vi "TI sbRIO Main (RT).vi"() -> ()   [LabVIEW 2013]
uses:
  Type Defs/Controller Names.ctl
  Controls/Alarm Config.ctl
  Controls/Alarm Definition.ctl
  Controls/Alarm Profile Config.ctl
  Type Defs/App Config.ctl
  SubVIs/Data Logger/Data Log Init.ctl
  Type Defs/Sequence States.ctl
  Type Defs/Controller List.ctl
  Controls/Tank CMDs.ctl
  Controls/Controller Config.ctl
  Controls/Pump Data.ctl
  Controls/Tank Data.ctl
  Controls/HMI Cluster.ctl
  Controls/HMI Header.ctl
  Controls/HMI Tog Buttons.ctl
  Controls/HMI Mom Buttons.ctl
  Controls/App Global Mode.ctl
  SubVIs/Data Logger/Data Logger Mode.ctl
  SubVIs/Data Logger/Data Log Start.ctl
  Controls/Power Supply Global Mode.ctl
  Controls/RPi HMI Mode.ctl
  Controls/Email Mode.ctl
  Type Defs/Pump Data Mode.ctl
  SubVIs/Watlow Modbus/Modbus Mode.ctl
  SubVIs/Watlow Modbus/Modbus Variable.ctl
  Controls/HMI Global Mode.ctl
  <vilib>/FPGAPlugInAG/sbRIO-9626/niLvFpga_Open_sbRIO-9626.vi
  <vilib>/Utility/error.llb/Error Cluster From Error Code.vi
  <vilib>/rvi/errors/niLvFpgaAdjustHostInterfaceError.vi
  <vilib>/Utility/file.llb/Write To Spreadsheet File (string).vi
  <vilib>/rvi/interface/nirviOpenFPGA/nirviOpenFPGA.xnode
  Controls/FPGA_Reference.ctl
  FPGA/bitfiles/TI sbRIO PWM (FPGA) v1.0.lvbitx
  <vilib>/rvi/interface/nirviReadWriteControl/nirviReadWriteControl.xnode
  NiFpgaLv.dll
  <vilib>/Utility/config.llb/NI_LVConfig.lvlib
panel:
  out "Read Inputs (ms)":u32
  out "Update Screen (ms)":u32
  out "Run Step (ms)":u32
  in  "Fuel Change Tab":enum32{"Page 1", "Page 2"}(tab)
  in  "pb.Fuel Change OK":bool
  in  "Reset Tab":enum32{"Page 1", "Page 2"}(tab)
  in  "pb.Reset OK":bool
  in  "pb.Reset Cancel":bool
  in  "Save As Tab":enum32{"Page 1", "Page 2"}(tab)
  in  "New Profile Name:":string
  in  "pb.Save As OK":bool
  in  "pb.Save As Cancel":bool
  in  "Alarm Tab":enum32{"Page 1", "Page 2"}(tab)
  out "Alarm Message":string
  in  "pb.Alarm OK":bool
  in  "Set Time Tab":enum32{"Page 1", "Page 2"}(tab)
  in  "pb.Set Time OK":bool
  in  "pb.Set Time Cancel":bool
  in  "New Time":dbl format="%<%H:%M:%S>t"
  in  "Pump Timers Tab":enum32{"Page 1", "Page 2"}(tab)
  in  "pb.Time Reset All":bool
  out "Elapsed Time:":dbl[](array[numeric])=[7.1, 7.1, 7.1, 458133.45, 458138.85000000003, 458126.75] format="%<%H:%M:%S>t"
  in  "pb.Resets":bool[](array[boolean])=[FALSE, FALSE, FALSE, FALSE, FALSE, FALSE]
  in  "pb.Sets":bool[](array[boolean])=[FALSE, FALSE, FALSE, FALSE, FALSE, FALSE]
  out "CPU Usage:":dbl=7.74131899555212 format="%.1f"
  in  "Live Data Tab":enum32{"Page 1", "Page 2"}(tab)
  in  "Controller\nCMD":dbl[](array[numeric])=[0.0, 0.0, 0.0, 0.0, 0.0, 0.0] min=0.0 max=1.0 step=1.0 format="%#.2f"
  out "Speed":dbl[](array[numeric]) caption="Speed\n(RPM)" format="%#.0f"
  out "ControllerCurrent":dbl[](array[numeric])=[0.015201568603515625, 0.00335693359375, 0.003021240234375, 0.12260055541992188, 0.06085968017578125, 0.052234649658203125] caption="Controller\nCurrent\n(DC)" format="%.1f"
  out "PumpCurrent":dbl[](array[numeric])=[0.015201568603515625, 0.00335693359375, 0.003021240234375, 0.12260055541992188, 0.06085968017578125, 0.052234649658203125] caption="Pump\nCurrent\n(DC)" format="%.1f"
  out "Flow":dbl[](array[numeric])=[0.0, 0.0, 0.0, 0.125, 0.0625, 0.0625] caption="Flow\n(L/H)" format="%#.0f"
  out "Pressure":dbl[](array[numeric])=[0.015201568603515625, 0.00335693359375, 0.003021240234375, 0.12260055541992188, 0.06085968017578125, 0.052234649658203125] caption="Pressure\n(kPa)" format="%#.0f"
  out "Ave. Speed":dbl=7.74131899555212 format="%.1f"
  out "Voltages":dbl[](array[numeric])=[0.015201568603515625, 0.00335693359375, 0.003021240234375, 0.12260055541992188, 0.06085968017578125, 0.052234649658203125] caption="Pump\nVoltage\n(V)" format="%.1f"
  in  "App Config":T1={"Location"="Tanks 162-163", "Profiles Path"=path "c:/Profiles", "Current Profile"="", "CA Number"="", "Cycles Completed"=0, "Controller Type:"=enum."Kuhnke", "Stagger Time (ms)"=0, "Tank 1 Fuel"="", "Tank 2 Fuel"="", "Serial Numbers"={"Position 1 SN"="", "Position 2 SN"="", "Poaition 3 SN"="", "Position 4 SN"="", "Position 5 SN"="", "Position 6 SN"=""}, "Pumps Present"={"Pump 1"=FALSE, "Pump 2"=FALSE, "Pump 3"=FALSE, "Pump 4"=FALSE, "Pump 5"=FALSE, "Pump 6"=FALSE}, "VoltCtrlRef"="", "VoltageSelect"=FALSE, "Watlow Present"=TRUE, "Temp 1"=0.0, "Temp 2"=0.0, "V_Run PI?"=FALSE, "Voltage Limits"={"V_Step"=1e-05, "V_CmdMax"=0.0, "V_CmdMin"=0.0}, "Voltage Far PI"={"V_FarSlew"=10.0, "V_FarKp"=0.0, "V_FarKi"=0.0}, "Voltage Mid PI"={"V_MidSlew"=10.0, "V_MidKp"=0.0, "V_MidKi"=0.0}, "Voltage Close PI"={"V_CloseSlew"=10.0, "V_CloseKp"=0.0, "V_CloseKi"=0.0}, "Voltage Scale"={"V_FFm"=0.0, "V_FFb"=0.0}, "Voltage Cutoffs"={"V_MidCutoff"=0.0, "V_CloseCutoff"=0.0}, "Pressure Scale"={"Pres_FFm"=1e-05, "Pres_FFb"=0.0}, "Temp Format"=0, "Temp Tolerance"=0.0, "Target Voltage"=0.0, "Target Pressure"=0.0, "Data Log Init"={"Data Path"=path "u:/Data", "Data Log Rate (S/s)"=1, "AKLH Rate (Hours/S)"=0.1, "Sync Time Offset (min)"=180, "IP Last 3"=0, "WebDAV IP"="10.31.176.36"}, "Email Handler IP"="10.30.189.34", "ADC Check"=FALSE}
  in  "Monitoring Tab":enum32{"Page 1", "Page 2"}(tab)
  out "Avg Press:":dbl=7.74131899555212
  in  "pb.E Stop":bool
  in  "Ignition Relay":T4
  in  "Power Relay":T4
  out "Temp2":dbl caption="Tank 2 Temp (C):" format="%.1f"
  out "Temp1":dbl caption="Tank 1 Temp (C):" format="%.1f"
  out "PS Actual (V):":dbl format="%.2f"
  in  "Power Supply Cmd:":dbl min=0.0 max=20.0 format="%#.2f"
  in  "PressureCMD":dbl caption="Pressure Cmd:" min=0.0 max=825.0 format="%#.2f"
  in  "Pumps Present":T4={"Pump 1"=TRUE, "Pump 2"=TRUE, "Pump 3"=TRUE, "Pump 4"=TRUE, "Pump 5"=TRUE, "Pump 6"=TRUE}
  in  "Tank 1 Temp Cmd:":dbl caption="deg C"
  in  "Tank 2 Temp Cmd:":dbl caption="deg C"
  in  "Title Tab":enum32{"Page 1", "Page 2"}(tab)
  in  "Title":string="TI Automotive sbRIO, v3.0"
  out "Time/Date":string
  in  "Login":bool
  in  "pb.Stop Profile":bool
  in  "Main Tab":T5(tab)
  out "Email Alarms Disabled":bool
  in  "Target Pressure:":dbl
  in  "Target Voltage:":dbl
  out "Recording":bool
  in  "Controller Type:":T2
  in  "Tank 1 Fuel Type:":string
  in  "Tank 2 Fuel Type:":string
  in  "Stagger Time (ms):":i32
  in  "CA Number:":string
  in  "Profile Name:":string(combo)="test"
  in  "pb.Save As":bool
  out "Current Step:":i32=2
  out "Step Time Left:":dbl=0.21101045608520508
  out "Cycles Completed:":u32=17
  in  "pb.Cycle Reset":bool
  out "Location:":string
  in  "pb.Run Profile":bool
  in  "Serial Numbers":T6
  in  "Profile:":string[][](table)=[["1", "2.0", "0.0", "0.0", "0.0", "67.6", "67.6", "67.6"], ["2", "1.0", "0.0", "0.0", "0.0", "10.0", "10.0", "10.0"]]
  in  "Disable Alarm Email":bool
  in  "Temp Tolerance":dbl=3.0 min=0.0 max=999999.0 step=1.0
  in  "Thermocouple":enum16{"2 TC/2 Tanks", "1 TC/1 Tank"}(ring)
  out "ADC Errors":i32
  in  "pb.Tare Pressure":bool
  in  "Data Log Enabled":bool=TRUE
  in  "RPMhyst":fxp<+,25,6>=1.0
  in  "pb.FuelChange":bool
  in  "Alarm Config":T7
  in  "WebDAV Push":bool
  in  "Concat Data":bool
  in  "Cutoffs":cluster{"Mid Range":dbl, "Close Range":dbl} {"Close Range" min=-100000.0 max=100000.0 step=1e-05 format="%#.5f"; "Mid Range" min=-100000.0 max=100000.0 step=1e-05 format="%#.5f"}
  in  "Mid PI":cluster{"Slew Rate":dbl, "Kp":dbl, "Ki":dbl}={"Slew Rate"=10.0, "Kp"=0.0, "Ki"=0.0} {"Ki" min=-100000.0 max=100000.0 step=1e-05 format="%#.5f"; "Kp" min=-100000.0 max=100000.0 step=1e-05 format="%#.5f"; "Slew Rate" min=0.0 max=1000000.0 step=0.01 format="%#.5f"}
  in  "Close PI":cluster{"Slew Rate":dbl, "Kp":dbl, "Ki":dbl}={"Slew Rate"=10.0, "Kp"=0.0, "Ki"=0.0} {"Ki" min=-100000.0 max=100000.0 step=1e-05 format="%#.5f"; "Kp" min=-100000.0 max=100000.0 step=1e-05 format="%#.5f"; "Slew Rate" min=0.0 max=1000000.0 step=0.01 format="%#.5f"}
  in  "Pressure Scale":cluster{"M":dbl, "B":dbl}={"M"=1e-05, "B"=0.0} {"B" min=-100000.0 max=100000.0 step=1e-05 format="%#.5f"; "M" min=-100000.0 max=100000.0 step=1e-05 format="%#.5f"}
  in  "Closed Loop Voltage":bool
  in  "Voltage Limits":cluster{"Step":dbl, "Max":dbl, "Min":dbl}={"Step"=1e-05, "Max"=0.0, "Min"=0.0} {"Min" min=0.0 max=10.0 step=1e-05 format="%#.5f"; "Max" min=0.0 max=10.0 step=1e-05 format="%#.5f"; "Step" min=0.0 max=100.0 step=1e-05 format="%#.5f"}
  in  "Far PI":cluster{"Slew Rate":dbl, "Kp":dbl, "Ki":dbl}={"Slew Rate"=10.0, "Kp"=0.0, "Ki"=0.0} {"Ki" min=-100000.0 max=100000.0 step=1e-05 format="%#.5f"; "Kp" min=-100000.0 max=100000.0 step=1e-05 format="%#.5f"; "Slew Rate" min=0.0 max=1000000.0 step=0.01 format="%#.5f"}
  in  "Voltage Scale":cluster{"M":dbl, "B":dbl} {"B" min=-100000.0 max=100000.0 step=1e-05 format="%#.5f"; "M" min=-100000.0 max=100000.0 step=1e-05 format="%#.5f"}
  # "Fuel Change was logged."
  # "Are you sure you want to reset?"
  # "Enter a new elapsed time."
  # "Pump Timers"
  # "Live Data"
  # "Manual Control"
  # "V"
  # "kPa"
  # "degC"
  # "degC"
  # "Voltage Control"
  # "Pressure Control"
  # "Data Server"
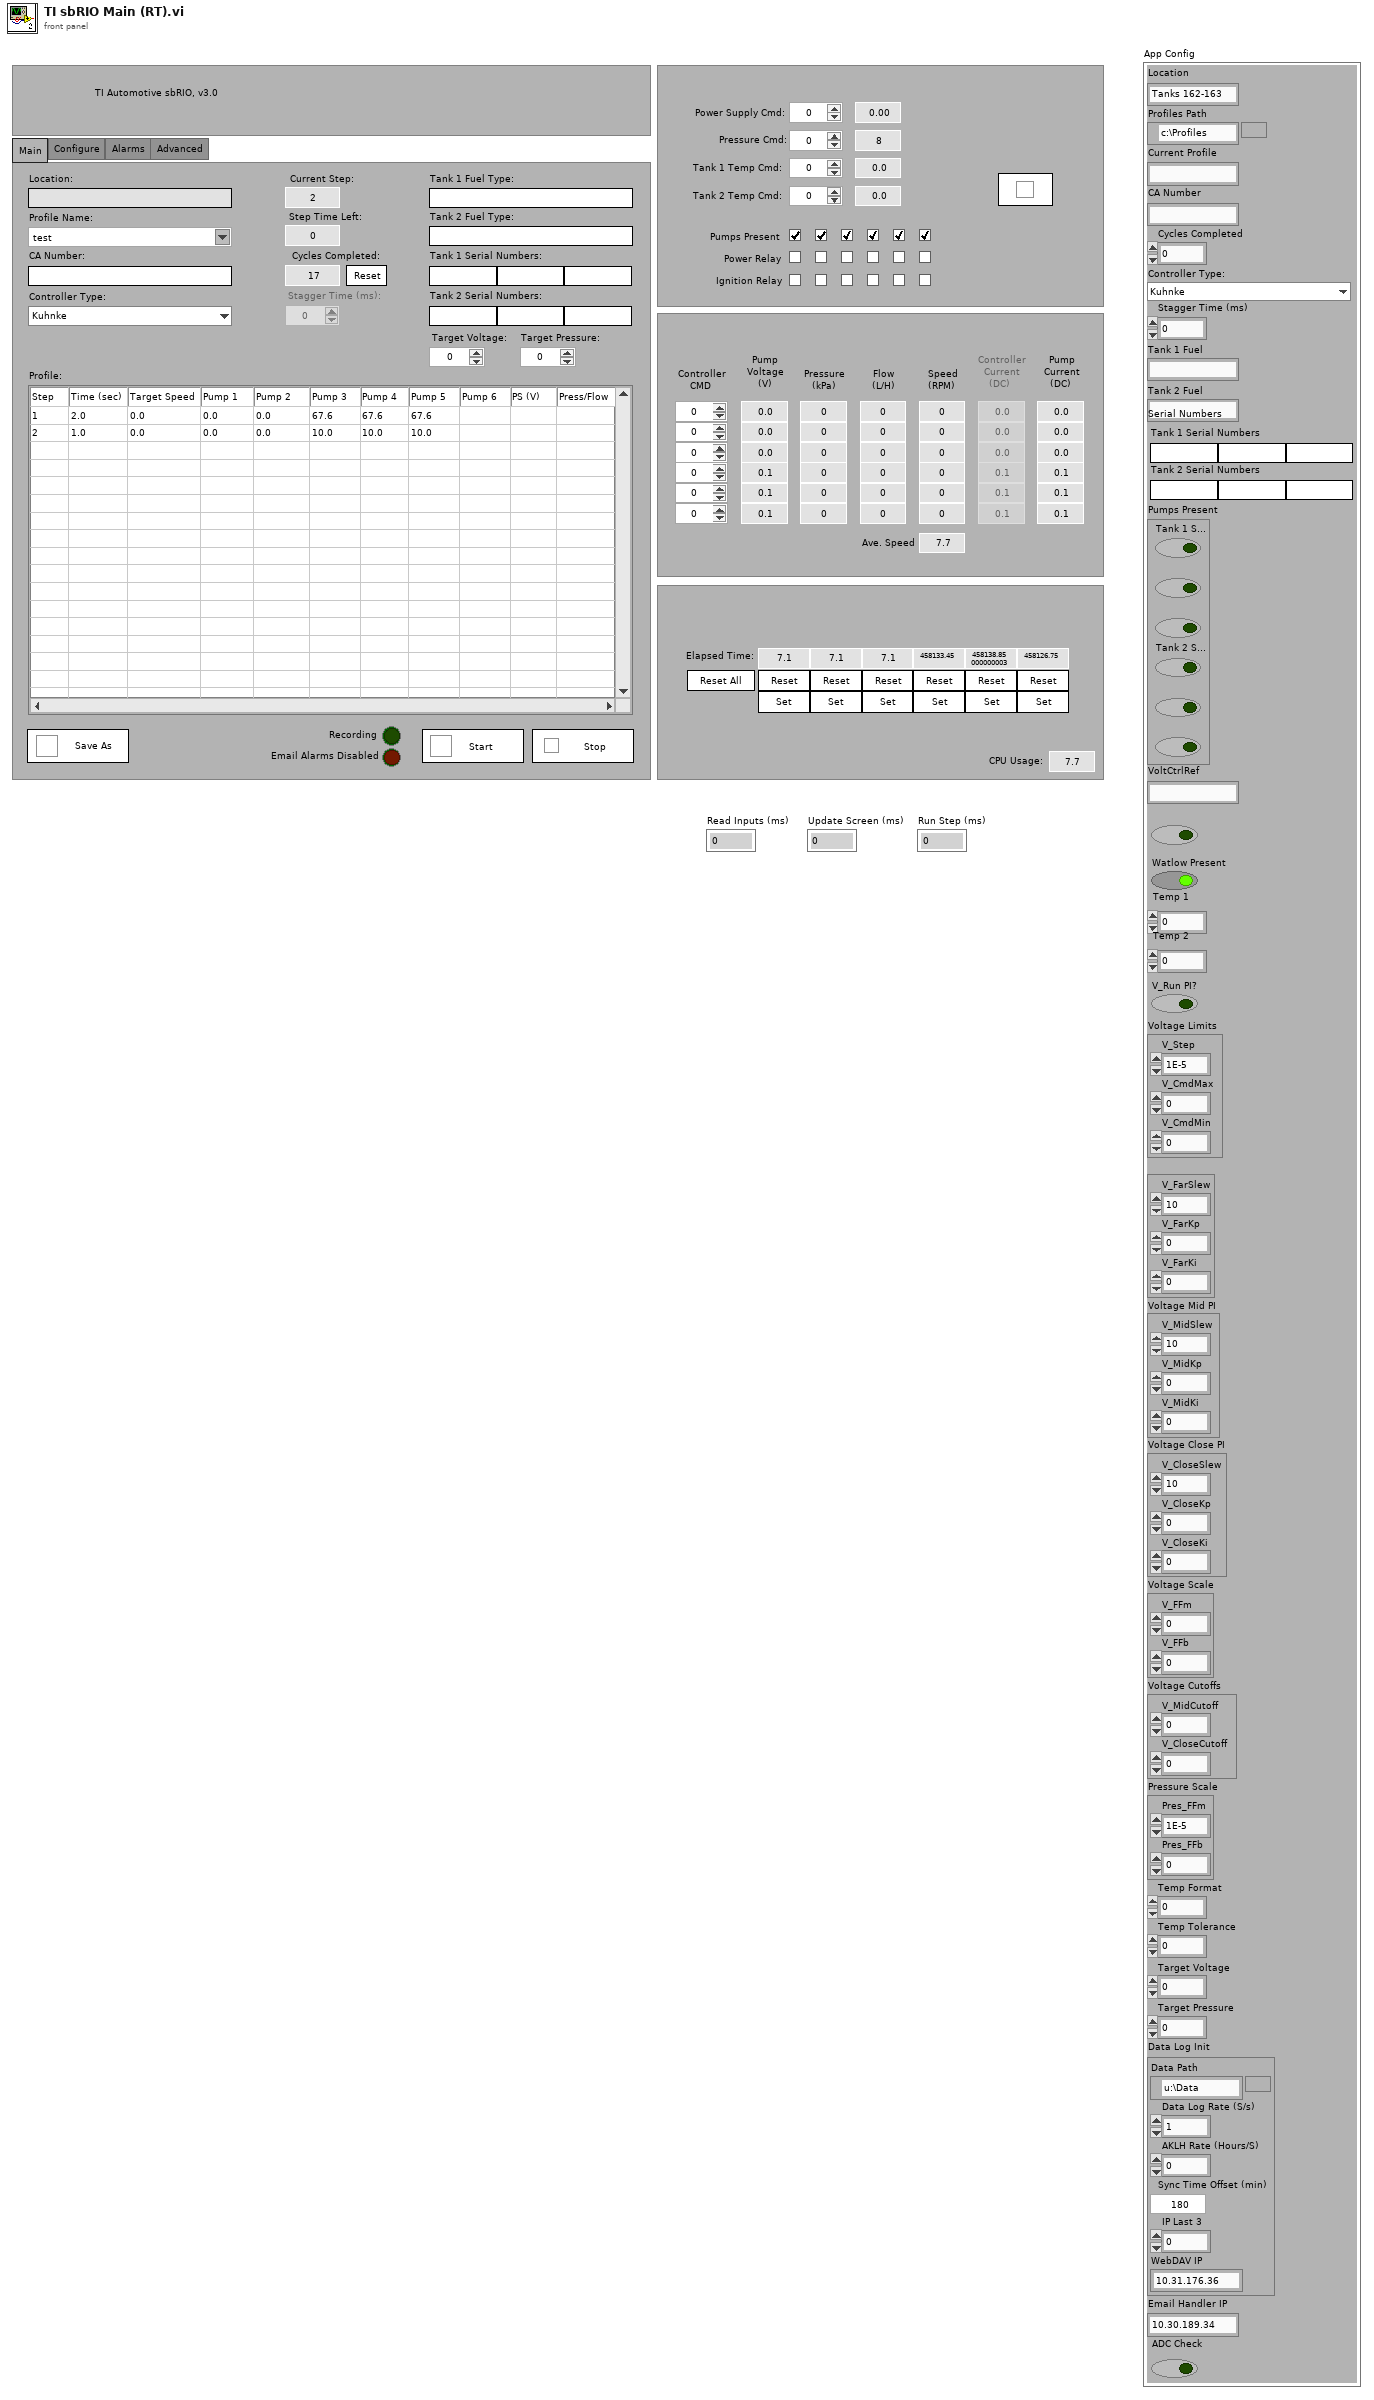
[diagram p1: front panel]
types:
  T1 = typedef "App Config.ctl" = cluster{"Location":string, "Profiles Path":path, "Current Profile":string, "CA Number":string, "Cycles Completed":u32, "Controller Type:":T2, "Stagger Time (ms)":i32, "Tank 1 Fuel":string, "Tank 2 Fuel":string, "Serial Numbers":cluster{"Position 1 SN":string, "Position 2 SN":string, "Poaition 3 SN":string, "Position 4 SN":string, "Position 5 SN":string, "Position 6 SN":string}, "Pumps Present":cluster{"Pump 1":bool, "Pump 2":bool, "Pump 3":bool, "Pump 4":bool, "Pump 5":bool, "Pump 6":bool}, "VoltCtrlRef":string, "VoltageSelect":bool, "Watlow Present":bool, "Temp 1":dbl, "Temp 2":dbl, "V_Run PI?":bool, "Voltage Limits":cluster{"V_Step":dbl, "V_CmdMax":dbl, "V_CmdMin":dbl}, "Voltage Far PI":cluster{"V_FarSlew":dbl, "V_FarKp":dbl, "V_FarKi":dbl}, "Voltage Mid PI":cluster{"V_MidSlew":dbl, "V_MidKp":dbl, "V_MidKi":dbl}, "Voltage Close PI":cluster{"V_CloseSlew":dbl, "V_CloseKp":dbl, "V_CloseKi":dbl}, "Voltage Scale":cluster{"V_FFm":dbl, "V_FFb":dbl}, "Voltage Cutoffs":cluster{"V_MidCutoff":dbl, "V_CloseCutoff":dbl}, "Pressure Scale":cluster{"Pres_FFm":dbl, "Pres_FFb":dbl}, "Temp Format":i32, "Temp Tolerance":dbl, "Target Voltage":dbl, "Target Pressure":dbl, "Data Log Init":T3, "Email Handler IP":string, "ADC Check":bool}
  T2 = typedef "Controller Names.ctl" = enum16{"Kuhnke", "Helbako BLDC", "Conti", "Hella BLDC OL PWM", "Hella BLDC Turbine OL PWM", "Hella BLDC Pressure", "Helbako (old)", "TI PWM", "PSA", "Hella Gas", "Hella Diesel", "8 Comm", "10 Comm", "8 Comm Hella", "10 Comm Hella", "8 Comm Omron", "10 Comm Omron", "8 Comm Nissan", "10 Comm Nissan"}
  T3 = typedef "Data Log Init.ctl" = cluster{"Data Path":path, "Data Log Rate (S/s)":u32, "AKLH Rate (Hours/S)":dbl, "Sync Time Offset (min)":u32, "IP Last 3":u32, "WebDAV IP":string}
  T4 = cluster{"Pump 1":bool, "Pump 2":bool, "Pump 3":bool, "Pump 4":bool, "Pump 5":bool, "Pump 6":bool}
  T5 = enum32{"Main", "Configure", "Alarms", "Advanced"}
  T6 = cluster{"Position 1 SN":string, "Position 2 SN":string, "Position 3 SN":string, "Position 4 SN":string, "Position 5 SN":string, "Position 6 SN":string}
  T7 = typedef "Alarm Config.ctl" = cluster{"Alarms:":T8[], "Profile Sync:":T9}
  T8 = typedef "Alarm Definition.ctl" = cluster{"Description:":string, "Enabled:":bool, "Data Index:":i32, "Data Type:":string, "Low Limit:":dbl, "High Limit:":dbl, "Trip Time:":u32, "Profile Sync:":bool}
  T9 = typedef "Alarm Profile Config.ctl" = cluster{"Trip Time:":u32, "Consecutive Trips:":i32}
  T10 = typedef "HMI Cluster.ctl" = cluster{"Error":errorcluster, "COM Ref":refnum<visa-resource-name>, "Pump Data":T11, "Tank Data":cluster{"PS Actual (V):":dbl, "Temp1":dbl, "Temp2":dbl}, "Power Relays":cluster{"Pump 1":bool, "Pump 2":bool, "Pump 3":bool, "Pump 4":bool, "Pump 5":bool, "Pump 6":bool}, "Pump CMDs":dbl[], "HMI Header":T12, "Tank CMDs":T13, "HMI Tog Buttons":T14, "In Test":bool, "HMI Command":bool, "HMI Mom Buttons":T15, "Controller Config":T16, "Alarm":bool, "Alarm Message 1":string, "Alarm Message 2":string, "Recording":bool, "Serial Numbers":string[], "Pumps Present":bool[]}
  T11 = typedef "Pump Data.ctl" = cluster{"Voltages":dbl[], "PumpCurrent":dbl[], "Speed":dbl[], "ControllerCurrent":dbl[], "Pressure":dbl[], "Flow":dbl[], "Elapsed Time:":dbl[], "Avg Pressure":dbl, "Avg Speed":dbl}
  T12 = typedef "HMI Header.ctl" = cluster{"Line 1":string, "Line 2":string, "Line 3":string, "Line 4":string}
  T13 = typedef "Tank CMDs.ctl" = cluster{"PS CMD":dbl, "Press CMD":dbl, "Temp 1 CMD":dbl, "Temp 2 CMD":dbl}
  T14 = typedef "HMI Tog Buttons.ctl" = cluster{"Start Test":bool, "Toggle Spare 1":bool, "Toggle Spare 2":bool, "Toggle Spare 3":bool, "Toggle Spare 4":bool, "Toggle Spare 5":bool}
  T15 = typedef "HMI Mom Buttons.ctl" = cluster{"Stop":bool, "Reset Timers":bool, "Log Fuel Change":bool, "Alarm Dismiss":bool}
  T16 = typedef "Controller Config.ctl" = cluster{"Controller Name":T2, "CommSeg":i32, "PWM?":bool, "Frequency":i32, "Low Command":dbl, "High Command":dbl, "Stop Command":dbl, "Command Step":dbl, "Solenoid Stop?":bool, "Controller?":bool, "Invert PWM":bool}
  T17 = typedef "Tank Data.ctl" = cluster{"PS Actual (V):":dbl, "Temp1":dbl, "Temp2":dbl}
  T18 = typedef "Controller List.ctl" = cluster{"Controller Name":T2, "CommSeg":i32, "PWM?":bool, "Frequency":i32, "Low Command":dbl, "High Command":dbl, "Stop Command":dbl, "Command Step":dbl, "Solenoid Stop?":bool, "Controller?":bool, "Invert PWM":bool}[]
  T19 = typedef "Sequence States.ctl" = enum16{"Main", "Init Files", "Init", "Unused", "Save As", "Start Profile", "Check Step Time", "Alarm", "Alarm Dismiss", "Run Step", "Stop Profile", "Cycle Reset", "Time Reset", "Time Reset All", "Time Set", "Tare CTs", "Save Profile", "Open Profile", "Get Profiles", "Update Screen", "Update Controls", "Save App Config", "Write Outputs", "Disable Background", "Enable Background", "Get/Release Control", "Log Fuel Change", "Fuel Change Popup", "Read Inputs", "Remote Timer Reset", "Controller Change", "Get Alarms", "Init Alarms", "Save Alarms", "Voltage Selection", "Set Watlow Temp 1", "Set Watlow Temp 2", "Get Pressure", "Write Tare Pressure", "Adjust Controls", "Reinit ADC", "Write Initial Times", "Write Pumps Present", "HMI Command", "Save Pump Times"}
  T20 = cluster{"Error":errorcluster, "Profile":string[][], "App Config":T1, "Profiles":string[], "Current Step":i32, "Step Time Left":dbl, "Run Profile":bool, "Step Start Time":dbl, "Step Time":dbl, " # of Steps":i32, "Screen Timer":u32, "Last Profile Time":dbl, "Controller CMDs":dbl[], "Client?":bool, "pb.Run Profile":bool, "pb.Resets":bool[], "pb.Sets":bool[], "Update Profile":bool, "Initial Times":dbl[], "Alarm":bool, "Pressure Offsets":dbl[], "Login":bool, "Stagger Counter":i32, "New Step":bool, "TenHz Path":path, "Inputs Timer":u32, "Main Tab":enum32{"Page 1", "Page 2"}, "Stop Cmd":dbl, "Tank Data":T17, "Voltage Enable":bool, "Power Relay":cluster{"Pump 1":bool, "Pump 2":bool, "Pump 3":bool, "Pump 4":bool, "Pump 5":bool, "Pump 6":bool}, "Ignition Relay":cluster{"Pump 1":bool, "Pump 2":bool, "Pump 3":bool, "Pump 4":bool, "Pump 5":bool, "Pump 6":bool}, "Controller List":T18, "Alarm Config":T7, "Alarm Config Path":path, "Trip Counters":i32[], "Previous Times":u32[], "Alarm Message 1":string, "Alarm Message 2":string, "Restart Alarm":bool, "Prev ON Times":u32[], "CalArray":dbl[][], "Tank CMDs":T13, "Controller Config":T16, "Fuel Log Path":path, "Pump Data":T11, "Alarm Latch":bool, "Time/Date":string, "Recording":bool, "HMI":T10, "WebDAV Push":bool, "Email Alarms Disabled":bool, "Concat Data":bool}
  T21 = typedef "FPGA_Reference.ctl" = refnum<k20>
  T22 = typedef "App Global Mode.ctl" = enum16{"Read", "Write Client", "Write Login"}
  T23 = typedef "Data Logger Mode.ctl" = enum16{"Init", "Main", "Start", "Stop"}
  T24 = enum16{"open", "replace", "create", "open or create", "replace or create", "replace or create with confirmation"}
  T25 = enum8{"Enabled", "Disabled", "Disabled and Grayed Out"}
  T26 = typedef "Data Log Start.ctl" = cluster{"App Config":T1, "Profile":string[][], "Controller Type":string, "Tank CMDs":T13}
  T27 = typedef "Power Supply Global Mode.ctl" = enum16{"Write Setpoint", "Write FreezePID", "Read"}
  T28 = typedef "RPi HMI Mode.ctl" = enum16{"Init", "Write Data", "Read from RPi", "Write to RPi"}
  T29 = typedef "Email Mode.ctl" = enum16{"Trigger Email", "Send Email"}
  T30 = typedef "Pump Data Mode.ctl" = enum16{"Read", "Write Data", "Write Cal", "Write Watlow Data", "Write Pressure Offsets", "Write Initial Times", "Write Pumps Present"}
  T31 = typedef "Modbus Variable.ctl" = enum16{"Temperature", "Setpoint"}
  T32 = typedef "Modbus Mode.ctl" = enum16{"Init", "Tank 1 Write", "Tank 2 Write", "Tank 1 Read", "Tank 2 Read"}
  T33 = typedef "HMI Global Mode.ctl" = enum16{"Read", "Write Cluster", "Reset Cmd"}
  T34 = cluster{"Position 1 SN":string, "Position 2 SN":string, "Poaition 3 SN":string, "Position 4 SN":string, "Position 5 SN":string, "Position 6 SN":string}
  T35 = cluster{"V_Step":dbl, "V_CmdMax":dbl, "V_CmdMin":dbl}
  T36 = cluster{"V_FarSlew":dbl, "V_FarKp":dbl, "V_FarKi":dbl}
  T37 = cluster{"V_MidSlew":dbl, "V_MidKp":dbl, "V_MidKi":dbl}
  T38 = cluster{"V_CloseSlew":dbl, "V_CloseKp":dbl, "V_CloseKi":dbl}
  T39 = typedef "NI_LVConfig.lvlib/Config Data RefNum.ctl" = refnum<k1>
  T40 = cluster{"Controller Name":T2, "CommSeg":i32, "PWM?":bool, "Frequency":i32, "Low Command":dbl, "High Command":dbl, "Stop Command":dbl, "Command Step":dbl, "Solenoid Stop?":bool, "Controller?":bool, "Invert PWM":bool}[]
  T41 = cluster{"Controller Name":T2, "CommSeg":i32, "PWM?":bool, "Frequency":i32, "Low Command":dbl, "High Command":dbl, "Stop Command":dbl, "Command Step":dbl, "Solenoid Stop?":bool, "Controller?":bool, "Invert PWM":bool}
  T42 = cluster{"[0]":bool, "[1]":bool, "[2]":bool, "[3]":bool, "[4]":bool, "[5]":bool}
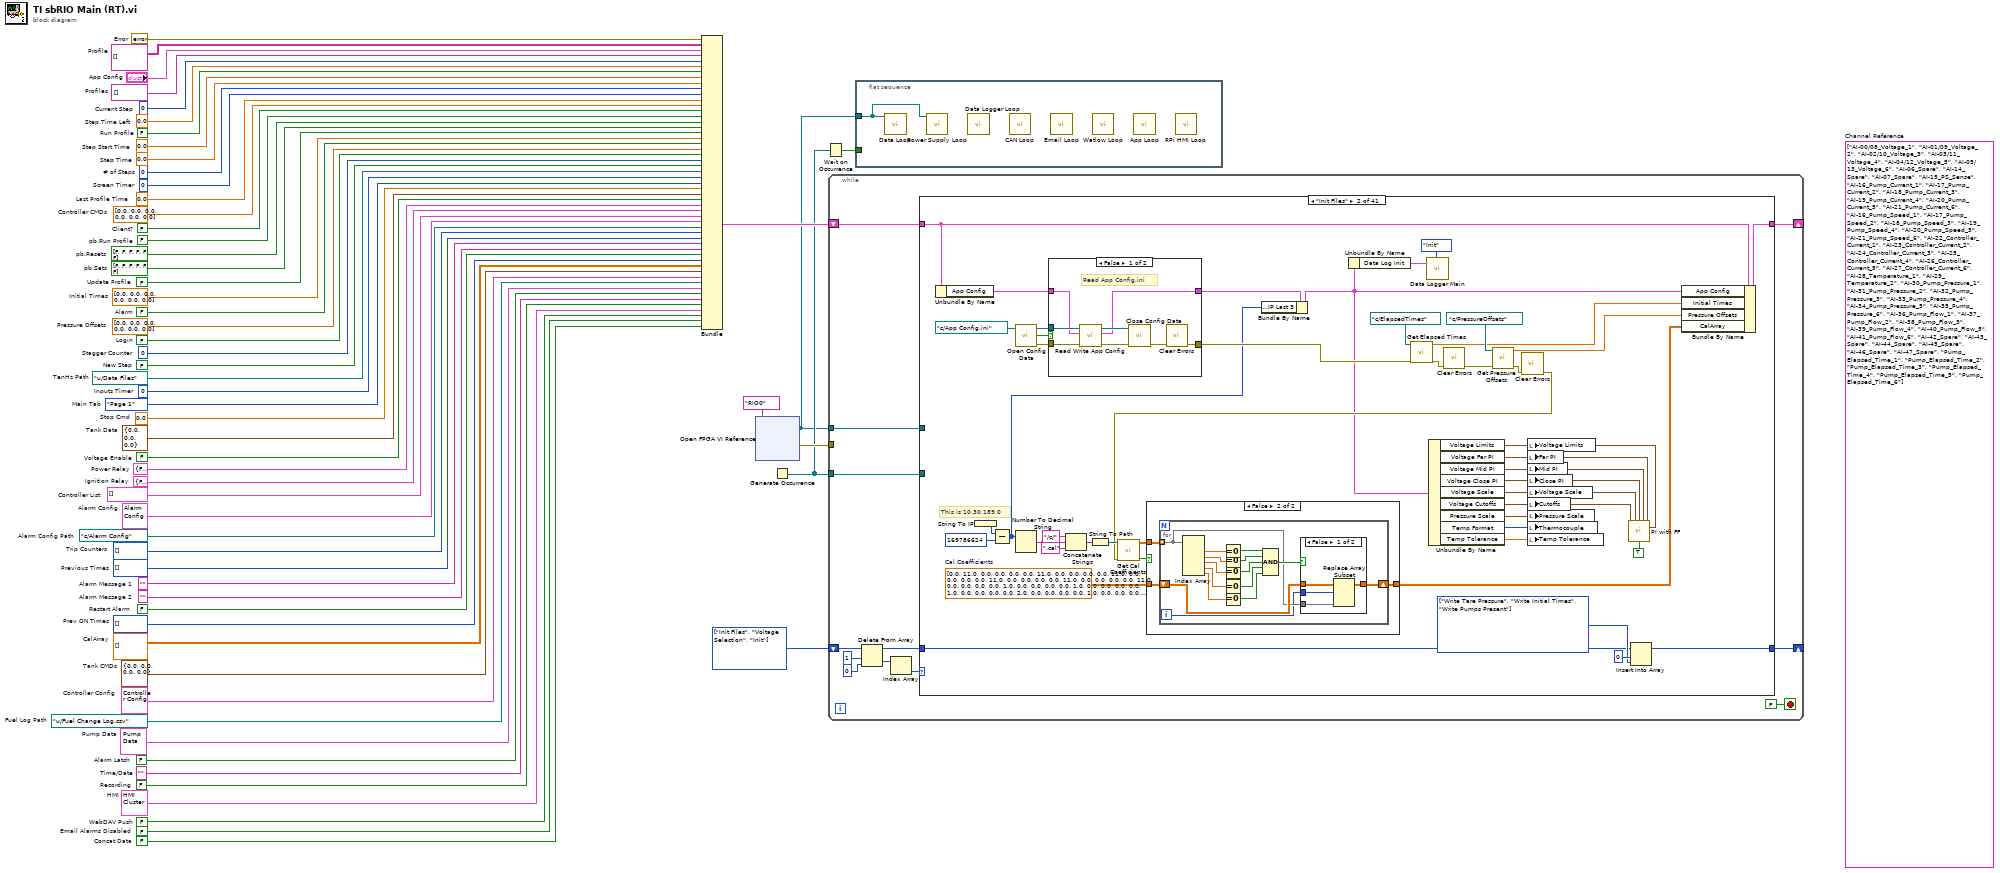
[diagram p0: block diagram]
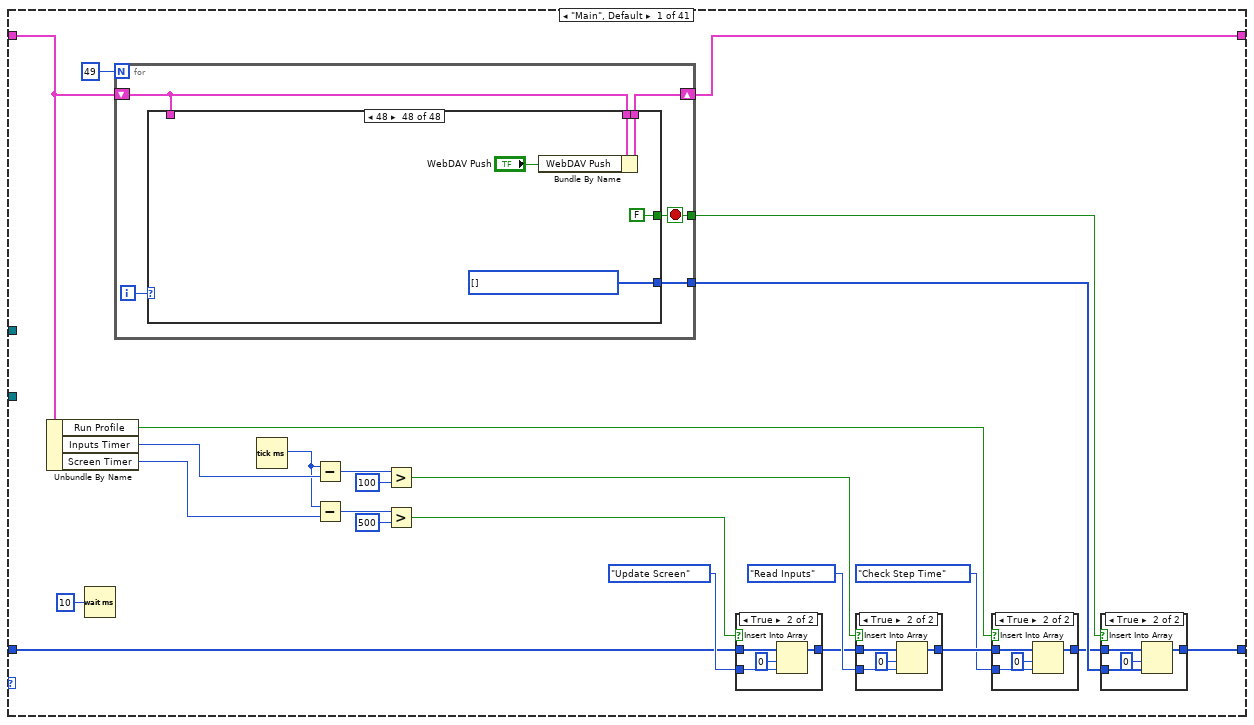
[diagram p2: hidden frame]
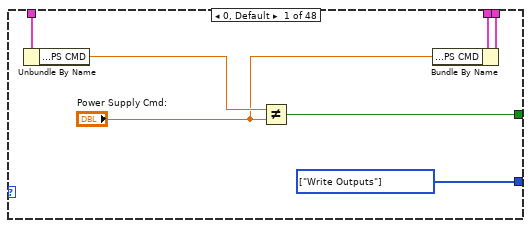
[diagram p7: hidden frame]
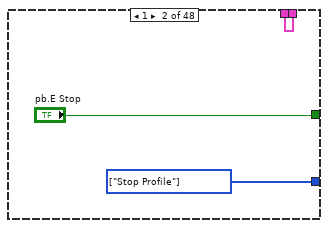
[diagram p8: hidden frame]
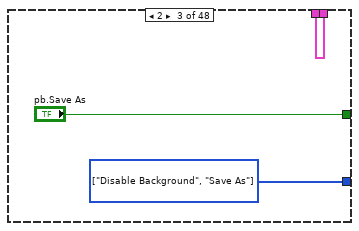
[diagram p9: hidden frame]
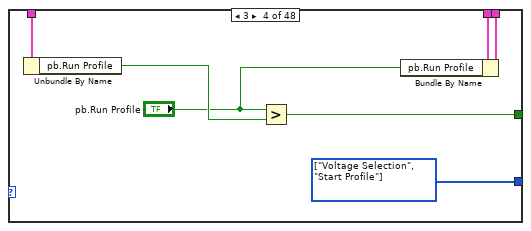
[diagram p10: hidden frame]
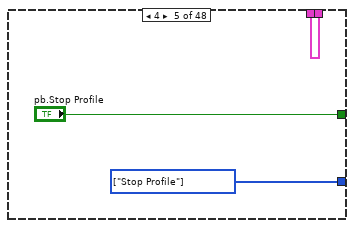
[diagram p11: hidden frame]
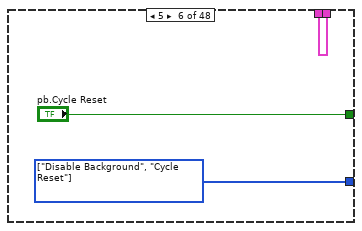
[diagram p12: hidden frame]
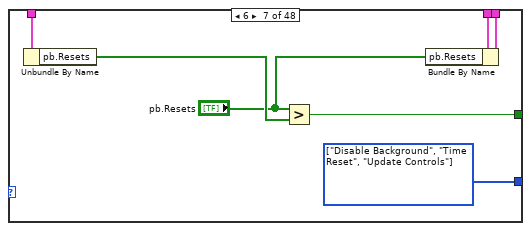
[diagram p13: hidden frame]
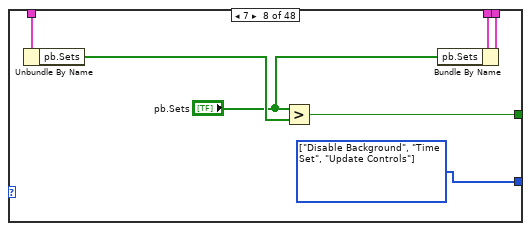
[diagram p14: hidden frame]
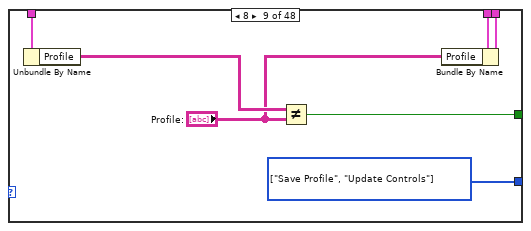
[diagram p15: hidden frame]
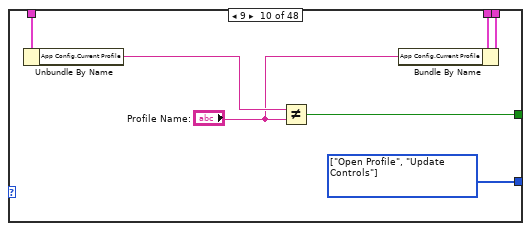
[diagram p16: hidden frame]
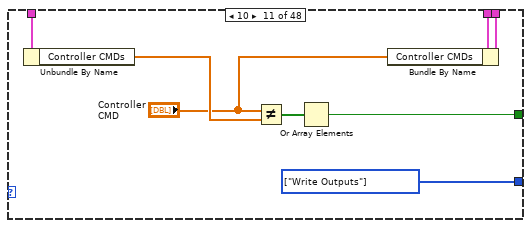
[diagram p17: hidden frame]
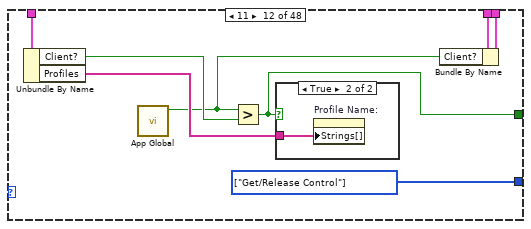
[diagram p18: hidden frame]
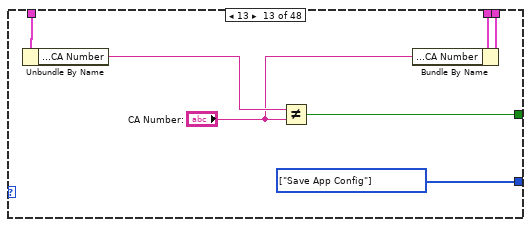
[diagram p20: hidden frame]
diagram:
  w1 = FALSE  # Concat Data
  w2 = FALSE  # Email Alarms Disabled
  w3 = FALSE  # WebDAV Push
  w4 = T10 {"Error"={"status"=FALSE, "code"=0, "source"=""}, "COM Ref"="", "Pump Data"={"Voltages"=[], "PumpCurrent"=[], "Speed"=[], "ControllerCurrent"=[], "Pressure"=[], "Flow"=[], "Elapsed Time:"=[], "Avg Pressure"=0.0, "Avg Speed"=0.0}, "Tank Data"={"PS Actual (V):"=0.0, "Temp1"=0.0, "Temp2"=0.0}, "Power Relays"={"Pump 1"=FALSE, "Pump 2"=FALSE, "Pump 3"=FALSE, "Pump 4"=FALSE, "Pump 5"=FALSE, "Pump 6"=FALSE}, "Pump CMDs"=[], "HMI Header"={"Line 1"="", "Line 2"="", "Line 3"="", "Line 4"=""}, "Tank CMDs"={"PS CMD"=0.0, "Press CMD"=0.0, "Temp 1 CMD"=0.0, "Temp 2 CMD"=0.0}, "HMI Tog Buttons"={"Start Test"=FALSE, "Toggle Spare 1"=FALSE, "Toggle Spare 2"=FALSE, "Toggle Spare 3"=FALSE, "Toggle Spare 4"=FALSE, "Toggle Spare 5"=FALSE}, "In Test"=FALSE, "HMI Command"=FALSE, "HMI Mom Buttons"={"Stop"=FALSE, "Reset Timers"=FALSE, "Log Fuel Change"=FALSE, "Alarm Dismiss"=FALSE}, "Controller Config"={"Controller Name"=enum."Kuhnke", "CommSeg"=0, "PWM?"=FALSE, "Frequency"=0, "Low Command"=0.0, "High Command"=0.0, "Stop Command"=0.0, "Command Step"=0.0, "Solenoid Stop?"=FALSE, "Controller?"=FALSE, "Invert PWM"=FALSE}, "Alarm"=FALSE, "Alarm Message 1"="", "Alarm Message 2"="", "Recording"=FALSE, "Serial Numbers"=[], "Pumps Present"=[]}  # HMI
  w8 = T17 {"PS Actual (V):"=0.0, "Temp1"=0.0, "Temp2"=0.0}  # Tank Data
  w9 = FALSE  # Recording
  w10 = ""  # Time/Date
  w11 = ""  # Alarm Message 2
  w12 = FALSE  # Alarm Latch
  w13 = T11 {"Voltages"=[0.015201568603515625, 0.00335693359375, 0.003021240234375, 0.12260055541992188, 0.06085968017578125, 0.052234649658203125], "PumpCurrent"=[0.015201568603515625, 0.00335693359375, 0.003021240234375, 0.12260055541992188, 0.06085968017578125, 0.052234649658203125], "Speed"=[0.0, 0.0, 0.0, 0.0, 0.0, 0.0], "ControllerCurrent"=[0.015201568603515625, 0.00335693359375, 0.003021240234375, 0.12260055541992188, 0.06085968017578125, 0.052234649658203125], "Pressure"=[0.015201568603515625, 0.00335693359375, 0.003021240234375, 0.12260055541992188, 0.06085968017578125, 0.052234649658203125], "Flow"=[0.0, 0.0, 0.0, 0.125, 0.0625, 0.0625], "Elapsed Time:"=[7.1, 7.1, 7.1, 458133.45, 458138.85000000003, 458126.75], "Avg Pressure"=0.0, "Avg Speed"=0.0}  # Pump Data
  w14 = path "u:/Fuel Change Log.csv"  # Fuel Log Path
  w15 = T16 {"Controller Name"=enum."Kuhnke", "CommSeg"=0, "PWM?"=FALSE, "Frequency"=0, "Low Command"=0.0, "High Command"=0.0, "Stop Command"=0.0, "Command Step"=0.0, "Solenoid Stop?"=FALSE, "Controller?"=FALSE, "Invert PWM"=FALSE}  # Controller Config
  w16 = T13 {"PS CMD"=0.0, "Press CMD"=0.0, "Temp 1 CMD"=0.0, "Temp 2 CMD"=0.0}  # Tank CMDs
  w17 = dbl[][] []  # CalArray
  w18 = u32[] []  # Prev ON Times
  w19 = FALSE  # Restart Alarm
  w20 = ""  # Alarm Message 1
  w21 = u32[] []  # Previous Times
  w22 = i32[] []  # Trip Counters
  w23 = path "c:/Alarm Config"  # Alarm Config Path
  w24 = T7 {"Alarms:"=[{"Description:"="", "Enabled:"=FALSE, "Data Index:"=0, "Data Type:"="", "Low Limit:"=0.0, "High Limit:"=0.0, "Trip Time:"=0, "Profile Sync:"=FALSE}, {"Description:"="", "Enabled:"=FALSE, "Data Index:"=0, "Data Type:"="", "Low Limit:"=0.0, "High Limit:"=0.0, "Trip Time:"=0, "Profile Sync:"=FALSE}, {"Description:"="", "Enabled:"=FALSE, "Data Index:"=0, "Data Type:"="", "Low Limit:"=0.0, "High Limit:"=0.0, "Trip Time:"=0, "Profile Sync:"=FALSE}, {"Description:"="", "Enabled:"=FALSE, "Data Index:"=0, "Data Type:"="", "Low Limit:"=0.0, "High Limit:"=0.0, "Trip Time:"=0, "Profile Sync:"=FALSE}, {"Description:"="", "Enabled:"=FALSE, "Data Index:"=0, "Data Type:"="", "Low Limit:"=0.0, "High Limit:"=0.0, "Trip Time:"=0, "Profile Sync:"=FALSE}, {"Description:"="", "Enabled:"=FALSE, "Data Index:"=0, "Data Type:"="", "Low Limit:"=0.0, "High Limit:"=0.0, "Trip Time:"=0, "Profile Sync:"=FALSE}, {"Description:"="", "Enabled:"=FALSE, "Data Index:"=0, "Data Type:"="", "Low Limit:"=0.0, "High Limit:"=0.0, "Trip Time:"=0, "Profile Sync:"=FALSE}, {"Description:"="", "Enabled:"=FALSE, "Data Index:"=0, "Data Type:"="", "Low Limit:"=0.0, "High Limit:"=0.0, "Trip Time:"=0, "Profile Sync:"=FALSE}], "Profile Sync:"={"Trip Time:"=0, "Consecutive Trips:"=0}}  # Alarm Config
  w25 = T18 []  # Controller List
  w26 = T4 {"Pump 1"=FALSE, "Pump 2"=FALSE, "Pump 3"=FALSE, "Pump 4"=FALSE, "Pump 5"=FALSE, "Pump 6"=FALSE}  # Ignition Relay
  w27 = T4 {"Pump 1"=FALSE, "Pump 2"=FALSE, "Pump 3"=FALSE, "Pump 4"=FALSE, "Pump 5"=FALSE, "Pump 6"=FALSE}  # Power Relay
  (unwired) string[] ["AI-00/08_Voltage_1", "AI-01/09_Voltage_2", "AI-02/10_Voltage_3", "AI-03/11_Voltage_4", "AI-04/12_Voltage_5", "AI-05/13_Voltage_6", "AI-06_Spare", "AI-14_Spare", "AI-07_Spare", "AI-15_PS_Sense", "AI-16_Pump_Current_1", "AI-17_Pump_Current_2", "AI-18_Pump_Current_3", "AI-19_Pump_Current_4", "AI-20_Pump_Current_5", "AI-21_Pump_Current_6", "AI-16_Pump_Speed_1", "AI-17_Pump_Speed_2", "AI-18_Pump_Speed_3", "AI-19_Pump_Speed_4", "AI-20_Pump_Speed_5", "AI-21_Pump_Speed_6", "AI-22_Controller_Current_1", "AI-23_Controller_Current_2", "AI-24_Controller_Current_3", "AI-25_Controller_Current_4", "AI-26_Controller_Current_5", "AI-27_Controller_Current_6", "AI-28_Temperature_1", "AI-29_Temperature_2", "AI-30_Pump_Pressure_1", "AI-31_Pump_Pressure_2", "AI-32_Pump_Pressure_3", "AI-33_Pump_Pressure_4", "AI-34_Pump_Pressure_5", "AI-35_Pump_Pressure_6", "AI-36_Pump_Flow_1", "AI-37_Pump_Flow_2", "AI-38_Pump_Flow_3", "AI-39_Pump_Flow_4", "AI-40_Pump_Flow_5", "AI-41_Pump_Flow_6", "AI-42_Spare", "AI-43_Spare", "AI-44_Spare", "AI-45_Spare", "AI-46_Spare", "AI-47_Spare", "Pump_Elapsed_Time_1", "Pump_Elapsed_Time_2", "Pump_Elapsed_Time_3", "Pump_Elapsed_Time_4", "Pump_Elapsed_Time_5", "Pump_Elapsed_Time_6"]  # Channel Reference
  w30 = FALSE  # Voltage Enable
  w31 = 0.0  # Stop Cmd
  w32 = enum32{"Page 1", "Page 2"}."Page 1"  # Main Tab
  w33 = u32 0  # Inputs Timer
  w34 = path "u:/Data Files"  # TenHz Path
  w35 = dbl[] [0.0, 0.0, 0.0, 0.0, 0.0, 0.0]  # Pressure Offsets
  w36 = T19[] [enum."Init Files", enum."Voltage Selection", enum."Init"] items=["Main", "Init Files", "Init", "Unused", "Save As", "Start Profile", "Check Step Time", "Alarm", "Alarm Dismiss", "Run Step", "Stop Profile", "Cycle Reset", "Time Reset", "Time Reset All", "Time Set", "Tare CTs", "Save Profile", "Open Profile", "Get Profiles", "Update Screen", "Update Controls", "Save App Config", "Write Outputs", "Disable Background", "Enable Background", "Get/Release Control", "Log Fuel Change", "Fuel Change Popup", "Read Inputs", "Remote Timer Reset", "Controller Change", "Get Alarms", "Init Alarms", "Save Alarms", "Voltage Selection", "Set Watlow Temp 1", "Set Watlow Temp 2", "Get Pressure", "Write Tare Pressure", "Adjust Controls", "Reinit ADC", "Write Initial Times", "Write Pumps Present", "HMI Command", "Save Pump Times"]
  w38 = FALSE  # New Step
  w39 = 0  # Stagger Counter
  w40 = FALSE  # Login
  w41 = FALSE  # Alarm
  w42 = dbl[] [0.0, 0.0, 0.0, 0.0, 0.0, 0.0]  # Initial Times
  w43 = FALSE  # Update Profile
  w44 = bool[] [FALSE, FALSE, FALSE, FALSE, FALSE, FALSE]  # pb.Sets
  w45 = bool[] [FALSE, FALSE, FALSE, FALSE, FALSE, FALSE]  # pb.Resets
  w46 = FALSE  # pb.Run Profile
  w47 = FALSE  # Client?
  w48 = dbl[] [0.0, 0.0, 0.0, 0.0, 0.0, 0.0]  # Controller CMDs
  w49 = 0.0  # Last Profile Time
  w50 = u32 0  # Screen Timer
  w51 = 0  # # of Steps
  w52 = 0.0  # Step Time
  w53 = 0.0  # Step Start Time
  w54 = FALSE  # Run Profile
  w56 = 0  # Current Step
  w55 = 0.0  # Step Time Left
  w57 = string[] []  # Profiles
  w59 = string[][] []  # Profile
  w60 = errorcluster {"status"=FALSE, "code"=0, "source"=""}  # Error
  n1 = Bundle("Error"=w60, "Profile"=w59, "App Config"="App Config", "Profiles"=w57, "Current Step"=w56, "Step Time Left"=w55, "Run Profile"=w54, "Step Start Time"=w53, "Step Time"=w52, "# of Steps"=w51, "Screen Timer"=w50, "Last Profile Time"=w49, "Controller CMDs"=w48, "Client?"=w47, "pb.Run Profile"=w46, "pb.Resets"=w45, "pb.Sets"=w44, "Update Profile"=w43, "Initial Times"=w42, "Alarm"=w41, "Pressure Offsets"=w35, "Login"=w40, "Stagger Counter"=w39, "New Step"=w38, "TenHz Path"=w34, "Inputs Timer"=w33, "Main Tab"=w32, "Stop Cmd"=w31, "Tank Data"=w8, "Voltage Enable"=w30, "Power Relay"=w27, "Ignition Relay"=w26, "Controller List"=w25, "Alarm Config"=w24, "Alarm Config Path"=w23, "Trip Counters"=w22, "Previous Times"=w21, "Alarm Message 1"=w20, "Alarm Message 2"=w11, "Restart Alarm"=w19, "Prev ON Times"=w18, "CalArray"=w17, "Tank CMDs"=w16, "Controller Config"=w15, "Fuel Log Path"=w14, "Pump Data"=w13, "Alarm Latch"=w12, "Time/Date"=w10, "Recording"=w9, "HMI"=w4, "WebDAV Push"=w3, "Email Alarms Disabled"=w2, "Concat Data"=w1) -> (w37:T20)  [unwired: 1 in]
  n2 = xnode "Open FPGA VI Reference"("resource name"=tag "RIO0") -> ("FPGA VI Reference Out"=w5:T21, "error out"=w29:errorcluster)  [unwired: 1 in]
  n3 = Generate Occurrence() -> (w7:refnum<k4>)
  n4 = Wait on Occurrence(2:w7) -> (0:w6:bool)  [unwired: 2 in]
  n5 = while {
    shift-right: [w69] -> _
    shift-left: w36 -> [w67]
    shift-right: [w70] -> _
    shift-left: w37 -> [w71]
    tunnel: w5 -> [w68]
    tunnel: w7 -> [w62]
    tunnel: w29 -> [_]
    stop <- FALSE stop-if-true
    n6 = Delete From Array(array=w67, length=1, index=0 ("length")) -> (deleted portion=w63:T19[], array with subset deleted=w66:T19[])
    n7 = Index Array(array=w63) -> (element=w61:T19)  [unwired: 1 in]
    n8 = case shown="\"Init Files\"" w61 {
      selector: w61 -> [_ _ _ _ _ _ _ _ _ _ _ _ _ _ _ _ _ _ _ _ _ _ _ w997 _ _ _ _ _ _ _ _ _ w1209 _ _ _ _ _ _ _]
      tunnel: [w76 w478 w548 w555 w562 w584 w604 w612 w628 w643 w666 w698 w737 w762 w812 w853 w900 w927 w948 w972 w978 w986 w992 w1007 w1051 w1065 w1085 w1114 w1121 w1131 w1134 w1144 w1194 w1214 w1232 w1246 w1255 w1264 w1266 w1272 w1287] -> w70
      tunnel: w71 -> [w96 w479 w542 w555 w563 w585 w604 w613 w629 w644 w655 w699 w738 w763 w838 w854 w900 w934 w949 w972 w978 w986 w992 w998 w1052 w1066 w1084 w1112 w1121 w1131 w1134 w1145 w1194 w1214 w1231 w1246 w1255 w1264 w1266 w1273 w1288]
      tunnel: [w90 w462 w537 w554 w559 w588 w605 w606 w617 w638 w658 w676 w732 w746 w807 w878 w913 w937 w943 w973 w979 w985 w988 w995 w1042 w1067 w1071 w1104 w1119 w1130 w1135 w1142 w1193 w1215 w1235 w1247 w1256 w1263 w1268 w1281 w1296] -> w69
      tunnel: w68 -> [_ _ w530 _ _ _ _ _ _ _ _ _ _ w757 w819 _ _ _ _ _ _ _ w991 w1001 _ _ w1077 w1113 _ _ _ w1146 _ _ _ _ _ w1259 _ _ _]
      tunnel: w66 -> [w83 w460 _ w554 w558 w588 w605 w607 w618 w638 w659 w677 w733 w747 w823 w877 w912 w938 w944 w973 w979 w985 w988 w996 w1043 w1068 w1072 w1103 w1119 w1130 w1136 w1143 w1193 w1215 w1236 w1247 w1256 w1263 w1268 w1282 w1297]
      tunnel: w62 -> [_ _ w532 _ _ _ _ _ _ _ _ _ _ _ _ _ _ _ _ _ _ _ _ _ _ _ _ _ _ _ _ _ _ _ _ _ _ _ _ _ _]
      frame "Main", Default {
        n9 = Unbundle By Name(w96) -> ("Run Profile"=w75:bool, "Inputs Timer"=w82:u32, "Screen Timer"=w81:u32)
        n10 = Wait (ms)(milliseconds to wait=u32 10) -> ()  [unwired: 1 out]
        n11 = for {
          N: 49 -> [_]
          shift-right: [w121] -> w76
          shift-left: w96 -> [w120]
          tunnel: [w119] -> w92
          tunnel: [w118] -> w91
          i -> [w117]
          stop <- w118 stop-if-true
          n12 = case shown="48" w117 {
            tunnel: w120 -> [w128 w130 w132 w141 w143 w145 w153 w160 w168 w175 w183 w191 w199 w206 w209 w210 w218 w226 w233 w241 w242 w250 w257 w264 w272 w276 w282 w298 w306 w313 w317 w320 w327 w336 w345 w354 w363 w372 w381 w390 w398 w405 w412 w419 w422 w429 w435 w440]
            tunnel: [w127 w130 w132 w140 w143 w145 w152 w159 w167 w174 w182 w190 w198 w205 w209 w210 w217 w225 w232 w240 w242 w249 w256 w263 w271 w275 w281 w297 w305 w312 w317 w320 w326 w335 w344 w353 w362 w371 w380 w389 w397 w404 w411 w418 w422 w428 w434 w439] -> w121
            tunnel: w120 -> [w126 _ _ w139 _ _ w150 w157 w166 w173 w181 w189 w197 w204 _ _ w215 w223 w230 w239 _ w248 w255 w262 w270 w277 w284 w299 w307 w314 _ _ w328 w337 w346 w355 w364 w373 w382 w391 w399 w406 w410 w417 _ w430 _ _]
            tunnel: [w125 w131 w133 w138 w144 w147 w148 w155 w163 w169 w180 w187 w193 w201 w208 w212 w214 w222 w229 w238 w244 w251 w258 w265 w269 w279 w289 w301 w308 w315 w318 w321 w323 w333 w338 w347 w356 w365 w374 w387 w395 w402 w413 w420 w424 w431 w436 w441] -> w119
            tunnel: [w122 "pb.E Stop" "pb.Save As" w135 "pb.Stop Profile" "pb.Cycle Reset" w151 w158 w164 w171 w176 w185 w195 w202 FALSE ("pb.Tare Pressure") "pb.Time Reset All" w216 w224 w231 w235 "pb.FuelChange" w245 w254 w259 w266 w278 w285 w300 w302 w309 "pb.Alarm OK" "pb.Tare Pressure" w324 w329 w339 w349 w358 w366 w376 w384 w394 w400 w408 w415 w421 w425 FALSE ("HMI Command") FALSE ("HMI Command")] -> w118
            frame 0, Default {
              w125 = T19[] [enum."Write Outputs"] items=["Main", "Init Files", "Init", "Unused", "Save As", "Start Profile", "Check Step Time", "Alarm", "Alarm Dismiss", "Run Step", "Stop Profile", "Cycle Reset", "Time Reset", "Time Reset All", "Time Set", "Tare CTs", "Save Profile", "Open Profile", "Get Profiles", "Update Screen", "Update Controls", "Save App Config", "Write Outputs", "Disable Background", "Enable Background", "Get/Release Control", "Log Fuel Change", "Fuel Change Popup", "Read Inputs", "Remote Timer Reset", "Controller Change", "Get Alarms", "Init Alarms", "Save Alarms", "Voltage Selection", "Set Watlow Temp 1", "Set Watlow Temp 2", "Get Pressure", "Write Tare Pressure", "Adjust Controls", "Reinit ADC", "Write Initial Times", "Write Pumps Present", "HMI Command", "Save Pump Times"]
              n13 = Unbundle By Name(w126) -> ("Tank CMDs.PS CMD"=w124:dbl)
              n14 = Not Equal?(x=w124, y="Power Supply Cmd:") -> (x != y?=w122:bool)
              n15 = Bundle By Name(cluster=w128, "Tank CMDs.PS CMD"="Power Supply Cmd:") -> (w127:T20)
            }
            frame 1 {
              w131 = T19[] [enum."Stop Profile"] items=["Main", "Init Files", "Init", "Unused", "Save As", "Start Profile", "Check Step Time", "Alarm", "Alarm Dismiss", "Run Step", "Stop Profile", "Cycle Reset", "Time Reset", "Time Reset All", "Time Set", "Tare CTs", "Save Profile", "Open Profile", "Get Profiles", "Update Screen", "Update Controls", "Save App Config", "Write Outputs", "Disable Background", "Enable Background", "Get/Release Control", "Log Fuel Change", "Fuel Change Popup", "Read Inputs", "Remote Timer Reset", "Controller Change", "Get Alarms", "Init Alarms", "Save Alarms", "Voltage Selection", "Set Watlow Temp 1", "Set Watlow Temp 2", "Get Pressure", "Write Tare Pressure", "Adjust Controls", "Reinit ADC", "Write Initial Times", "Write Pumps Present", "HMI Command", "Save Pump Times"]
            }
            frame 2 {
              w133 = T19[] [enum."Disable Background", enum."Save As"] items=["Main", "Init Files", "Init", "Unused", "Save As", "Start Profile", "Check Step Time", "Alarm", "Alarm Dismiss", "Run Step", "Stop Profile", "Cycle Reset", "Time Reset", "Time Reset All", "Time Set", "Tare CTs", "Save Profile", "Open Profile", "Get Profiles", "Update Screen", "Update Controls", "Save App Config", "Write Outputs", "Disable Background", "Enable Background", "Get/Release Control", "Log Fuel Change", "Fuel Change Popup", "Read Inputs", "Remote Timer Reset", "Controller Change", "Get Alarms", "Init Alarms", "Save Alarms", "Voltage Selection", "Set Watlow Temp 1", "Set Watlow Temp 2", "Get Pressure", "Write Tare Pressure", "Adjust Controls", "Reinit ADC", "Write Initial Times", "Write Pumps Present", "HMI Command", "Save Pump Times"]
            }
            frame 3 {
              w138 = T19[] [enum."Voltage Selection", enum."Start Profile"] items=["Main", "Init Files", "Init", "Unused", "Save As", "Start Profile", "Check Step Time", "Alarm", "Alarm Dismiss", "Run Step", "Stop Profile", "Cycle Reset", "Time Reset", "Time Reset All", "Time Set", "Tare CTs", "Save Profile", "Open Profile", "Get Profiles", "Update Screen", "Update Controls", "Save App Config", "Write Outputs", "Disable Background", "Enable Background", "Get/Release Control", "Log Fuel Change", "Fuel Change Popup", "Read Inputs", "Remote Timer Reset", "Controller Change", "Get Alarms", "Init Alarms", "Save Alarms", "Voltage Selection", "Set Watlow Temp 1", "Set Watlow Temp 2", "Get Pressure", "Write Tare Pressure", "Adjust Controls", "Reinit ADC", "Write Initial Times", "Write Pumps Present", "HMI Command", "Save Pump Times"]
              n16 = Unbundle By Name(w139) -> ("pb.Run Profile"=w137:bool)
              n17 = Greater?(x="pb.Run Profile", y=w137) -> (0:w135:bool)
              n18 = Bundle By Name(cluster=w141, "pb.Run Profile"="pb.Run Profile") -> (w140:T20)
            }
            frame 4 {
              w144 = T19[] [enum."Stop Profile"] items=["Main", "Init Files", "Init", "Unused", "Save As", "Start Profile", "Check Step Time", "Alarm", "Alarm Dismiss", "Run Step", "Stop Profile", "Cycle Reset", "Time Reset", "Time Reset All", "Time Set", "Tare CTs", "Save Profile", "Open Profile", "Get Profiles", "Update Screen", "Update Controls", "Save App Config", "Write Outputs", "Disable Background", "Enable Background", "Get/Release Control", "Log Fuel Change", "Fuel Change Popup", "Read Inputs", "Remote Timer Reset", "Controller Change", "Get Alarms", "Init Alarms", "Save Alarms", "Voltage Selection", "Set Watlow Temp 1", "Set Watlow Temp 2", "Get Pressure", "Write Tare Pressure", "Adjust Controls", "Reinit ADC", "Write Initial Times", "Write Pumps Present", "HMI Command", "Save Pump Times"]
            }
            frame 5 {
              w147 = T19[] [enum."Disable Background", enum."Cycle Reset"] items=["Main", "Init Files", "Init", "Unused", "Save As", "Start Profile", "Check Step Time", "Alarm", "Alarm Dismiss", "Run Step", "Stop Profile", "Cycle Reset", "Time Reset", "Time Reset All", "Time Set", "Tare CTs", "Save Profile", "Open Profile", "Get Profiles", "Update Screen", "Update Controls", "Save App Config", "Write Outputs", "Disable Background", "Enable Background", "Get/Release Control", "Log Fuel Change", "Fuel Change Popup", "Read Inputs", "Remote Timer Reset", "Controller Change", "Get Alarms", "Init Alarms", "Save Alarms", "Voltage Selection", "Set Watlow Temp 1", "Set Watlow Temp 2", "Get Pressure", "Write Tare Pressure", "Adjust Controls", "Reinit ADC", "Write Initial Times", "Write Pumps Present", "HMI Command", "Save Pump Times"]
            }
            frame 6 {
              w148 = T19[] [enum."Disable Background", enum."Time Reset", enum."Update Controls"] items=["Main", "Init Files", "Init", "Unused", "Save As", "Start Profile", "Check Step Time", "Alarm", "Alarm Dismiss", "Run Step", "Stop Profile", "Cycle Reset", "Time Reset", "Time Reset All", "Time Set", "Tare CTs", "Save Profile", "Open Profile", "Get Profiles", "Update Screen", "Update Controls", "Save App Config", "Write Outputs", "Disable Background", "Enable Background", "Get/Release Control", "Log Fuel Change", "Fuel Change Popup", "Read Inputs", "Remote Timer Reset", "Controller Change", "Get Alarms", "Init Alarms", "Save Alarms", "Voltage Selection", "Set Watlow Temp 1", "Set Watlow Temp 2", "Get Pressure", "Write Tare Pressure", "Adjust Controls", "Reinit ADC", "Write Initial Times", "Write Pumps Present", "HMI Command", "Save Pump Times"]
              n19 = Unbundle By Name(w150) -> ("pb.Resets"=w154:bool[])
              n20 = Greater?(x="pb.Resets", y=w154) -> (0:w151:bool)
              n21 = Bundle By Name(cluster=w153, "pb.Resets"="pb.Resets") -> (w152:T20)
            }
            frame 7 {
              w155 = T19[] [enum."Disable Background", enum."Time Set", enum."Update Controls"] items=["Main", "Init Files", "Init", "Unused", "Save As", "Start Profile", "Check Step Time", "Alarm", "Alarm Dismiss", "Run Step", "Stop Profile", "Cycle Reset", "Time Reset", "Time Reset All", "Time Set", "Tare CTs", "Save Profile", "Open Profile", "Get Profiles", "Update Screen", "Update Controls", "Save App Config", "Write Outputs", "Disable Background", "Enable Background", "Get/Release Control", "Log Fuel Change", "Fuel Change Popup", "Read Inputs", "Remote Timer Reset", "Controller Change", "Get Alarms", "Init Alarms", "Save Alarms", "Voltage Selection", "Set Watlow Temp 1", "Set Watlow Temp 2", "Get Pressure", "Write Tare Pressure", "Adjust Controls", "Reinit ADC", "Write Initial Times", "Write Pumps Present", "HMI Command", "Save Pump Times"]
              n22 = Unbundle By Name(w157) -> ("pb.Sets"=w161:bool[])
              n23 = Greater?(x="pb.Sets", y=w161) -> (0:w158:bool)
              n24 = Bundle By Name(cluster=w160, "pb.Sets"="pb.Sets") -> (w159:T20)
            }
            frame 8 {
              w163 = T19[] [enum."Save Profile", enum."Update Controls"] items=["Main", "Init Files", "Init", "Unused", "Save As", "Start Profile", "Check Step Time", "Alarm", "Alarm Dismiss", "Run Step", "Stop Profile", "Cycle Reset", "Time Reset", "Time Reset All", "Time Set", "Tare CTs", "Save Profile", "Open Profile", "Get Profiles", "Update Screen", "Update Controls", "Save App Config", "Write Outputs", "Disable Background", "Enable Background", "Get/Release Control", "Log Fuel Change", "Fuel Change Popup", "Read Inputs", "Remote Timer Reset", "Controller Change", "Get Alarms", "Init Alarms", "Save Alarms", "Voltage Selection", "Set Watlow Temp 1", "Set Watlow Temp 2", "Get Pressure", "Write Tare Pressure", "Adjust Controls", "Reinit ADC", "Write Initial Times", "Write Pumps Present", "HMI Command", "Save Pump Times"]
              n25 = Unbundle By Name(w166) -> ("Profile"=w165:string[][])
              n26 = Not Equal?(x=w165, y="Profile:") -> (x != y?=w164:bool)
              n27 = Bundle By Name(cluster=w168, "Profile"="Profile:") -> (w167:T20)
            }
            frame 9 {
              w169 = T19[] [enum."Open Profile", enum."Update Controls"] items=["Main", "Init Files", "Init", "Unused", "Save As", "Start Profile", "Check Step Time", "Alarm", "Alarm Dismiss", "Run Step", "Stop Profile", "Cycle Reset", "Time Reset", "Time Reset All", "Time Set", "Tare CTs", "Save Profile", "Open Profile", "Get Profiles", "Update Screen", "Update Controls", "Save App Config", "Write Outputs", "Disable Background", "Enable Background", "Get/Release Control", "Log Fuel Change", "Fuel Change Popup", "Read Inputs", "Remote Timer Reset", "Controller Change", "Get Alarms", "Init Alarms", "Save Alarms", "Voltage Selection", "Set Watlow Temp 1", "Set Watlow Temp 2", "Get Pressure", "Write Tare Pressure", "Adjust Controls", "Reinit ADC", "Write Initial Times", "Write Pumps Present", "HMI Command", "Save Pump Times"]
              n28 = Unbundle By Name(w173) -> ("App Config.Current Profile"=w172:string)
              n29 = Not Equal?(x=w172, y="Profile Name:") -> (x != y?=w171:bool)
              n30 = Bundle By Name(cluster=w175, "App Config.Current Profile"="Profile Name:") -> (w174:T20)
            }
            frame 10 {
              w180 = T19[] [enum."Write Outputs"] items=["Main", "Init Files", "Init", "Unused", "Save As", "Start Profile", "Check Step Time", "Alarm", "Alarm Dismiss", "Run Step", "Stop Profile", "Cycle Reset", "Time Reset", "Time Reset All", "Time Set", "Tare CTs", "Save Profile", "Open Profile", "Get Profiles", "Update Screen", "Update Controls", "Save App Config", "Write Outputs", "Disable Background", "Enable Background", "Get/Release Control", "Log Fuel Change", "Fuel Change Popup", "Read Inputs", "Remote Timer Reset", "Controller Change", "Get Alarms", "Init Alarms", "Save Alarms", "Voltage Selection", "Set Watlow Temp 1", "Set Watlow Temp 2", "Get Pressure", "Write Tare Pressure", "Adjust Controls", "Reinit ADC", "Write Initial Times", "Write Pumps Present", "HMI Command", "Save Pump Times"]
              n31 = Unbundle By Name(w181) -> ("Controller CMDs"=w179:dbl[])
              n32 = Not Equal?(x="Controller\nCMD", y=w179) -> (x != y?=w177:bool[])
              n33 = Or Array Elements(Boolean array=w177) -> (logical OR=w176:bool)
              n34 = Bundle By Name(cluster=w183, "Controller CMDs"="Controller\nCMD") -> (w182:T20)
            }
            frame 11 {
              w187 = T19[] [enum."Get/Release Control"] items=["Main", "Init Files", "Init", "Unused", "Save As", "Start Profile", "Check Step Time", "Alarm", "Alarm Dismiss", "Run Step", "Stop Profile", "Cycle Reset", "Time Reset", "Time Reset All", "Time Set", "Tare CTs", "Save Profile", "Open Profile", "Get Profiles", "Update Screen", "Update Controls", "Save App Config", "Write Outputs", "Disable Background", "Enable Background", "Get/Release Control", "Log Fuel Change", "Fuel Change Popup", "Read Inputs", "Remote Timer Reset", "Controller Change", "Get Alarms", "Init Alarms", "Save Alarms", "Voltage Selection", "Set Watlow Temp 1", "Set Watlow Temp 2", "Get Pressure", "Write Tare Pressure", "Adjust Controls", "Reinit ADC", "Write Initial Times", "Write Pumps Present", "HMI Command", "Save Pump Times"]
              n35 = Unbundle By Name(w189) -> ("Client?"=w186:bool, "Profiles"=w188:string[])
              n36 = call "App Global.vi"() -> ("Client? OUT"=w184:bool)  [unwired: 9 in, 2 out]
              n37 = Greater?(x=w184, y=w186) -> (0:w185:bool)
              n38 = case shown="True" w185 {
                tunnel: w188 -> [_ w192]
                frame False {
                }
                frame True {
                  n39 = property on="Profile Name:" class="CmbBox"("Strings[]"=w192) -> ()  [unwired: 2 in, 2 out]
                }
              }
              n40 = Bundle By Name(cluster=w191, "Client?"=w184) -> (w190:T20)
            }
            frame 13 {
              w193 = T19[] [enum."Save App Config"] items=["Main", "Init Files", "Init", "Unused", "Save As", "Start Profile", "Check Step Time", "Alarm", "Alarm Dismiss", "Run Step", "Stop Profile", "Cycle Reset", "Time Reset", "Time Reset All", "Time Set", "Tare CTs", "Save Profile", "Open Profile", "Get Profiles", "Update Screen", "Update Controls", "Save App Config", "Write Outputs", "Disable Background", "Enable Background", "Get/Release Control", "Log Fuel Change", "Fuel Change Popup", "Read Inputs", "Remote Timer Reset", "Controller Change", "Get Alarms", "Init Alarms", "Save Alarms", "Voltage Selection", "Set Watlow Temp 1", "Set Watlow Temp 2", "Get Pressure", "Write Tare Pressure", "Adjust Controls", "Reinit ADC", "Write Initial Times", "Write Pumps Present", "HMI Command", "Save Pump Times"]
              n41 = Unbundle By Name(w197) -> ("App Config.CA Number"=w196:string)
              n42 = Not Equal?(x=w196, y="CA Number:") -> (x != y?=w195:bool)
              n43 = Bundle By Name(cluster=w199, "App Config.CA Number"="CA Number:") -> (w198:T20)
            }
            frame 14 {
              w201 = T19[] [enum."Save App Config", enum."Controller Change"] items=["Main", "Init Files", "Init", "Unused", "Save As", "Start Profile", "Check Step Time", "Alarm", "Alarm Dismiss", "Run Step", "Stop Profile", "Cycle Reset", "Time Reset", "Time Reset All", "Time Set", "Tare CTs", "Save Profile", "Open Profile", "Get Profiles", "Update Screen", "Update Controls", "Save App Config", "Write Outputs", "Disable Background", "Enable Background", "Get/Release Control", "Log Fuel Change", "Fuel Change Popup", "Read Inputs", "Remote Timer Reset", "Controller Change", "Get Alarms", "Init Alarms", "Save Alarms", "Voltage Selection", "Set Watlow Temp 1", "Set Watlow Temp 2", "Get Pressure", "Write Tare Pressure", "Adjust Controls", "Reinit ADC", "Write Initial Times", "Write Pumps Present", "HMI Command", "Save Pump Times"]
              n44 = Unbundle By Name(w204) -> ("App Config.Controller Type:"=w203:T2)
              n45 = Not Equal?(x=w203, y="Controller Type:") -> (x != y?=w202:bool)
              n46 = Bundle By Name(cluster=w206, "App Config.Controller Type:"="Controller Type:") -> (w205:T20)
            }
            frame 15 {
              w208 = T19[] [] items=["Main", "Init Files", "Init", "Unused", "Save As", "Start Profile", "Check Step Time", "Alarm", "Alarm Dismiss", "Run Step", "Stop Profile", "Cycle Reset", "Time Reset", "Time Reset All", "Time Set", "Tare CTs", "Save Profile", "Open Profile", "Get Profiles", "Update Screen", "Update Controls", "Save App Config", "Write Outputs", "Disable Background", "Enable Background", "Get/Release Control", "Log Fuel Change", "Fuel Change Popup", "Read Inputs", "Remote Timer Reset", "Controller Change", "Get Alarms", "Init Alarms", "Save Alarms", "Voltage Selection", "Set Watlow Temp 1", "Set Watlow Temp 2", "Get Pressure", "Write Tare Pressure", "Adjust Controls", "Reinit ADC", "Write Initial Times", "Write Pumps Present", "HMI Command", "Save Pump Times"]
            }
            frame 16 {
              w212 = T19[] [enum."Disable Background", enum."Time Reset All", enum."Update Controls"] items=["Main", "Init Files", "Init", "Unused", "Save As", "Start Profile", "Check Step Time", "Alarm", "Alarm Dismiss", "Run Step", "Stop Profile", "Cycle Reset", "Time Reset", "Time Reset All", "Time Set", "Tare CTs", "Save Profile", "Open Profile", "Get Profiles", "Update Screen", "Update Controls", "Save App Config", "Write Outputs", "Disable Background", "Enable Background", "Get/Release Control", "Log Fuel Change", "Fuel Change Popup", "Read Inputs", "Remote Timer Reset", "Controller Change", "Get Alarms", "Init Alarms", "Save Alarms", "Voltage Selection", "Set Watlow Temp 1", "Set Watlow Temp 2", "Get Pressure", "Write Tare Pressure", "Adjust Controls", "Reinit ADC", "Write Initial Times", "Write Pumps Present", "HMI Command", "Save Pump Times"]
            }
            frame 17 {
              w214 = T19[] [enum."Save App Config", enum."Write Pumps Present"] items=["Main", "Init Files", "Init", "Unused", "Save As", "Start Profile", "Check Step Time", "Alarm", "Alarm Dismiss", "Run Step", "Stop Profile", "Cycle Reset", "Time Reset", "Time Reset All", "Time Set", "Tare CTs", "Save Profile", "Open Profile", "Get Profiles", "Update Screen", "Update Controls", "Save App Config", "Write Outputs", "Disable Background", "Enable Background", "Get/Release Control", "Log Fuel Change", "Fuel Change Popup", "Read Inputs", "Remote Timer Reset", "Controller Change", "Get Alarms", "Init Alarms", "Save Alarms", "Voltage Selection", "Set Watlow Temp 1", "Set Watlow Temp 2", "Get Pressure", "Write Tare Pressure", "Adjust Controls", "Reinit ADC", "Write Initial Times", "Write Pumps Present", "HMI Command", "Save Pump Times"]
              n47 = Unbundle By Name(w215) -> ("App Config.Pumps Present"=w219:T4)
              n48 = Not Equal?(x="Pumps Present", y=w219) -> (x != y?=w216:bool)
              n49 = Bundle By Name(cluster=w218, "App Config.Pumps Present"="Pumps Present") -> (w217:T20)
            }
            frame 18 {
              w222 = T19[] [enum."Get/Release Control"] items=["Main", "Init Files", "Init", "Unused", "Save As", "Start Profile", "Check Step Time", "Alarm", "Alarm Dismiss", "Run Step", "Stop Profile", "Cycle Reset", "Time Reset", "Time Reset All", "Time Set", "Tare CTs", "Save Profile", "Open Profile", "Get Profiles", "Update Screen", "Update Controls", "Save App Config", "Write Outputs", "Disable Background", "Enable Background", "Get/Release Control", "Log Fuel Change", "Fuel Change Popup", "Read Inputs", "Remote Timer Reset", "Controller Change", "Get Alarms", "Init Alarms", "Save Alarms", "Voltage Selection", "Set Watlow Temp 1", "Set Watlow Temp 2", "Get Pressure", "Write Tare Pressure", "Adjust Controls", "Reinit ADC", "Write Initial Times", "Write Pumps Present", "HMI Command", "Save Pump Times"]
              n50 = Unbundle By Name(w223) -> ("Login"=w227:bool)
              n51 = call "App Global.vi"("Mode"=App_Global_Mode."Write Login", "Login"="Login") -> ()  [unwired: 7 in, 3 out]
              n52 = Not Equal?(x="Login", y=w227) -> (x != y?=w224:bool)
              n53 = Bundle By Name(cluster=w226, "Login"="Login") -> (w225:T20)
            }
            frame 19 {
              w229 = T19[] [enum."Save App Config"] items=["Main", "Init Files", "Init", "Unused", "Save As", "Start Profile", "Check Step Time", "Alarm", "Alarm Dismiss", "Run Step", "Stop Profile", "Cycle Reset", "Time Reset", "Time Reset All", "Time Set", "Tare CTs", "Save Profile", "Open Profile", "Get Profiles", "Update Screen", "Update Controls", "Save App Config", "Write Outputs", "Disable Background", "Enable Background", "Get/Release Control", "Log Fuel Change", "Fuel Change Popup", "Read Inputs", "Remote Timer Reset", "Controller Change", "Get Alarms", "Init Alarms", "Save Alarms", "Voltage Selection", "Set Watlow Temp 1", "Set Watlow Temp 2", "Get Pressure", "Write Tare Pressure", "Adjust Controls", "Reinit ADC", "Write Initial Times", "Write Pumps Present", "HMI Command", "Save Pump Times"]
              n54 = Unbundle By Name(w230) -> ("App Config.Stagger Time (ms)"=w234:i32)
              n55 = Not Equal?(x="Stagger Time (ms):", y=w234) -> (x != y?=w231:bool)
              n56 = Bundle By Name(cluster=w233, "App Config.Stagger Time (ms)"="Stagger Time (ms):") -> (w232:T20)
            }
            frame 20 {
              w238 = T19[] [enum."Write Outputs"] items=["Main", "Init Files", "Init", "Unused", "Save As", "Start Profile", "Check Step Time", "Alarm", "Alarm Dismiss", "Run Step", "Stop Profile", "Cycle Reset", "Time Reset", "Time Reset All", "Time Set", "Tare CTs", "Save Profile", "Open Profile", "Get Profiles", "Update Screen", "Update Controls", "Save App Config", "Write Outputs", "Disable Background", "Enable Background", "Get/Release Control", "Log Fuel Change", "Fuel Change Popup", "Read Inputs", "Remote Timer Reset", "Controller Change", "Get Alarms", "Init Alarms", "Save Alarms", "Voltage Selection", "Set Watlow Temp 1", "Set Watlow Temp 2", "Get Pressure", "Write Tare Pressure", "Adjust Controls", "Reinit ADC", "Write Initial Times", "Write Pumps Present", "HMI Command", "Save Pump Times"]
              n57 = Unbundle By Name(w239) -> ("Tank CMDs.Press CMD"=w237:dbl)
              n58 = Not Equal?(x="PressureCMD", y=w237) -> (x != y?=w235:bool)
              n59 = Bundle By Name(cluster=w241, "Tank CMDs.Press CMD"="PressureCMD") -> (w240:T20)
            }
            frame 21 {
              w244 = T19[] [enum."Disable Background", enum."Log Fuel Change", enum."Fuel Change Popup"] items=["Main", "Init Files", "Init", "Unused", "Save As", "Start Profile", "Check Step Time", "Alarm", "Alarm Dismiss", "Run Step", "Stop Profile", "Cycle Reset", "Time Reset", "Time Reset All", "Time Set", "Tare CTs", "Save Profile", "Open Profile", "Get Profiles", "Update Screen", "Update Controls", "Save App Config", "Write Outputs", "Disable Background", "Enable Background", "Get/Release Control", "Log Fuel Change", "Fuel Change Popup", "Read Inputs", "Remote Timer Reset", "Controller Change", "Get Alarms", "Init Alarms", "Save Alarms", "Voltage Selection", "Set Watlow Temp 1", "Set Watlow Temp 2", "Get Pressure", "Write Tare Pressure", "Adjust Controls", "Reinit ADC", "Write Initial Times", "Write Pumps Present", "HMI Command", "Save Pump Times"]
            }
            frame 22 {
              w251 = T19[] [enum."Save App Config"] items=["Main", "Init Files", "Init", "Unused", "Save As", "Start Profile", "Check Step Time", "Alarm", "Alarm Dismiss", "Run Step", "Stop Profile", "Cycle Reset", "Time Reset", "Time Reset All", "Time Set", "Tare CTs", "Save Profile", "Open Profile", "Get Profiles", "Update Screen", "Update Controls", "Save App Config", "Write Outputs", "Disable Background", "Enable Background", "Get/Release Control", "Log Fuel Change", "Fuel Change Popup", "Read Inputs", "Remote Timer Reset", "Controller Change", "Get Alarms", "Init Alarms", "Save Alarms", "Voltage Selection", "Set Watlow Temp 1", "Set Watlow Temp 2", "Get Pressure", "Write Tare Pressure", "Adjust Controls", "Reinit ADC", "Write Initial Times", "Write Pumps Present", "HMI Command", "Save Pump Times"]
              n60 = Unbundle By Name(w248) -> ("App Config.Tank 1 Fuel"=w247:string)
              n61 = Not Equal?(x=w247, y="Tank 1 Fuel Type:") -> (x != y?=w245:bool)
              n62 = Bundle By Name(cluster=w250, "App Config.Tank 1 Fuel"="Tank 1 Fuel Type:") -> (w249:T20)
            }
            frame 23 {
              w258 = T19[] [enum."Save App Config"] items=["Main", "Init Files", "Init", "Unused", "Save As", "Start Profile", "Check Step Time", "Alarm", "Alarm Dismiss", "Run Step", "Stop Profile", "Cycle Reset", "Time Reset", "Time Reset All", "Time Set", "Tare CTs", "Save Profile", "Open Profile", "Get Profiles", "Update Screen", "Update Controls", "Save App Config", "Write Outputs", "Disable Background", "Enable Background", "Get/Release Control", "Log Fuel Change", "Fuel Change Popup", "Read Inputs", "Remote Timer Reset", "Controller Change", "Get Alarms", "Init Alarms", "Save Alarms", "Voltage Selection", "Set Watlow Temp 1", "Set Watlow Temp 2", "Get Pressure", "Write Tare Pressure", "Adjust Controls", "Reinit ADC", "Write Initial Times", "Write Pumps Present", "HMI Command", "Save Pump Times"]
              n63 = Unbundle By Name(w255) -> ("App Config.Tank 2 Fuel"=w253:string)
              n64 = Not Equal?(x=w253, y="Tank 2 Fuel Type:") -> (x != y?=w254:bool)
              n65 = Bundle By Name(cluster=w257, "App Config.Tank 2 Fuel"="Tank 2 Fuel Type:") -> (w256:T20)
            }
            frame 24 {
              w265 = T19[] [enum."Save App Config"] items=["Main", "Init Files", "Init", "Unused", "Save As", "Start Profile", "Check Step Time", "Alarm", "Alarm Dismiss", "Run Step", "Stop Profile", "Cycle Reset", "Time Reset", "Time Reset All", "Time Set", "Tare CTs", "Save Profile", "Open Profile", "Get Profiles", "Update Screen", "Update Controls", "Save App Config", "Write Outputs", "Disable Background", "Enable Background", "Get/Release Control", "Log Fuel Change", "Fuel Change Popup", "Read Inputs", "Remote Timer Reset", "Controller Change", "Get Alarms", "Init Alarms", "Save Alarms", "Voltage Selection", "Set Watlow Temp 1", "Set Watlow Temp 2", "Get Pressure", "Write Tare Pressure", "Adjust Controls", "Reinit ADC", "Write Initial Times", "Write Pumps Present", "HMI Command", "Save Pump Times"]
              n66 = Unbundle By Name(w262) -> ("App Config.Serial Numbers"=w261:T34)
              n67 = Not Equal?(x=w261, y="Serial Numbers") -> (x != y?=w259:bool)
              n68 = Bundle By Name(cluster=w264, "App Config.Serial Numbers"="Serial Numbers") -> (w263:T20)
            }
            frame 25 {
              w269 = T19[] [enum."Write Pumps Present", enum."Save App Config"] items=["Main", "Init Files", "Init", "Unused", "Save As", "Start Profile", "Check Step Time", "Alarm", "Alarm Dismiss", "Run Step", "Stop Profile", "Cycle Reset", "Time Reset", "Time Reset All", "Time Set", "Tare CTs", "Save Profile", "Open Profile", "Get Profiles", "Update Screen", "Update Controls", "Save App Config", "Write Outputs", "Disable Background", "Enable Background", "Get/Release Control", "Log Fuel Change", "Fuel Change Popup", "Read Inputs", "Remote Timer Reset", "Controller Change", "Get Alarms", "Init Alarms", "Save Alarms", "Voltage Selection", "Set Watlow Temp 1", "Set Watlow Temp 2", "Get Pressure", "Write Tare Pressure", "Adjust Controls", "Reinit ADC", "Write Initial Times", "Write Pumps Present", "HMI Command", "Save Pump Times"]
              n69 = Unbundle By Name(w270) -> ("Power Relay"=w268:T4)
              n70 = Not Equal?(x="Power Relay", y=w268) -> (x != y?=w266:bool)
              n71 = Bundle By Name(cluster=w272, "Power Relay"="Power Relay") -> (w271:T20)
            }
            frame 26 {
              w279 = T19[] [enum."Write Pumps Present", enum."Save App Config"] items=["Main", "Init Files", "Init", "Unused", "Save As", "Start Profile", "Check Step Time", "Alarm", "Alarm Dismiss", "Run Step", "Stop Profile", "Cycle Reset", "Time Reset", "Time Reset All", "Time Set", "Tare CTs", "Save Profile", "Open Profile", "Get Profiles", "Update Screen", "Update Controls", "Save App Config", "Write Outputs", "Disable Background", "Enable Background", "Get/Release Control", "Log Fuel Change", "Fuel Change Popup", "Read Inputs", "Remote Timer Reset", "Controller Change", "Get Alarms", "Init Alarms", "Save Alarms", "Voltage Selection", "Set Watlow Temp 1", "Set Watlow Temp 2", "Get Pressure", "Write Tare Pressure", "Adjust Controls", "Reinit ADC", "Write Initial Times", "Write Pumps Present", "HMI Command", "Save Pump Times"]
              n72 = Unbundle By Name(w277) -> ("Ignition Relay"=w274:T4)
              n73 = Not Equal?(x="Ignition Relay", y=w274) -> (x != y?=w278:bool)
              n74 = Bundle By Name(cluster=w276, "Ignition Relay"="Ignition Relay") -> (w275:T20)
            }
            frame 27 {
              n75 = Unbundle By Name(w284) -> ("HMI.HMI Mom Buttons"=w283:T15)
              n76 = Cluster To Array(cluster=w283) -> (array=w288:bool[])
              n77 = Search 1D Array(1D array=w288, element=TRUE) -> (index of element=w286:i32)  [unwired: 1 in]
              n78 = case shown="1" w286 {
                tunnel: [w290 w291 w292 w293 w294] -> w289
                frame -1, Default {
                  w290 = T19[] [] items=["Main", "Init Files", "Init", "Unused", "Save As", "Start Profile", "Check Step Time", "Alarm", "Alarm Dismiss", "Run Step", "Stop Profile", "Cycle Reset", "Time Reset", "Time Reset All", "Time Set", "Tare CTs", "Save Profile", "Open Profile", "Get Profiles", "Update Screen", "Update Controls", "Save App Config", "Write Outputs", "Disable Background", "Enable Background", "Get/Release Control", "Log Fuel Change", "Fuel Change Popup", "Read Inputs", "Remote Timer Reset", "Controller Change", "Get Alarms", "Init Alarms", "Save Alarms", "Voltage Selection", "Set Watlow Temp 1", "Set Watlow Temp 2", "Get Pressure", "Write Tare Pressure", "Adjust Controls", "Reinit ADC", "Write Initial Times", "Write Pumps Present", "HMI Command", "Save Pump Times"]
                }
                frame 0 {
                  w291 = T19[] [enum."Stop Profile"] items=["Main", "Init Files", "Init", "Unused", "Save As", "Start Profile", "Check Step Time", "Alarm", "Alarm Dismiss", "Run Step", "Stop Profile", "Cycle Reset", "Time Reset", "Time Reset All", "Time Set", "Tare CTs", "Save Profile", "Open Profile", "Get Profiles", "Update Screen", "Update Controls", "Save App Config", "Write Outputs", "Disable Background", "Enable Background", "Get/Release Control", "Log Fuel Change", "Fuel Change Popup", "Read Inputs", "Remote Timer Reset", "Controller Change", "Get Alarms", "Init Alarms", "Save Alarms", "Voltage Selection", "Set Watlow Temp 1", "Set Watlow Temp 2", "Get Pressure", "Write Tare Pressure", "Adjust Controls", "Reinit ADC", "Write Initial Times", "Write Pumps Present", "HMI Command", "Save Pump Times"]
                }
                frame 1 {
                  w292 = T19[] [enum."Remote Timer Reset"] items=["Main", "Init Files", "Init", "Unused", "Save As", "Start Profile", "Check Step Time", "Alarm", "Alarm Dismiss", "Run Step", "Stop Profile", "Cycle Reset", "Time Reset", "Time Reset All", "Time Set", "Tare CTs", "Save Profile", "Open Profile", "Get Profiles", "Update Screen", "Update Controls", "Save App Config", "Write Outputs", "Disable Background", "Enable Background", "Get/Release Control", "Log Fuel Change", "Fuel Change Popup", "Read Inputs", "Remote Timer Reset", "Controller Change", "Get Alarms", "Init Alarms", "Save Alarms", "Voltage Selection", "Set Watlow Temp 1", "Set Watlow Temp 2", "Get Pressure", "Write Tare Pressure", "Adjust Controls", "Reinit ADC", "Write Initial Times", "Write Pumps Present", "HMI Command", "Save Pump Times"]
                }
                frame 2 {
                  w293 = T19[] [enum."Log Fuel Change"] items=["Main", "Init Files", "Init", "Unused", "Save As", "Start Profile", "Check Step Time", "Alarm", "Alarm Dismiss", "Run Step", "Stop Profile", "Cycle Reset", "Time Reset", "Time Reset All", "Time Set", "Tare CTs", "Save Profile", "Open Profile", "Get Profiles", "Update Screen", "Update Controls", "Save App Config", "Write Outputs", "Disable Background", "Enable Background", "Get/Release Control", "Log Fuel Change", "Fuel Change Popup", "Read Inputs", "Remote Timer Reset", "Controller Change", "Get Alarms", "Init Alarms", "Save Alarms", "Voltage Selection", "Set Watlow Temp 1", "Set Watlow Temp 2", "Get Pressure", "Write Tare Pressure", "Adjust Controls", "Reinit ADC", "Write Initial Times", "Write Pumps Present", "HMI Command", "Save Pump Times"]
                }
                frame 3 {
                  w294 = T19[] [enum."Alarm Dismiss"] items=["Main", "Init Files", "Init", "Unused", "Save As", "Start Profile", "Check Step Time", "Alarm", "Alarm Dismiss", "Run Step", "Stop Profile", "Cycle Reset", "Time Reset", "Time Reset All", "Time Set", "Tare CTs", "Save Profile", "Open Profile", "Get Profiles", "Update Screen", "Update Controls", "Save App Config", "Write Outputs", "Disable Background", "Enable Background", "Get/Release Control", "Log Fuel Change", "Fuel Change Popup", "Read Inputs", "Remote Timer Reset", "Controller Change", "Get Alarms", "Init Alarms", "Save Alarms", "Voltage Selection", "Set Watlow Temp 1", "Set Watlow Temp 2", "Get Pressure", "Write Tare Pressure", "Adjust Controls", "Reinit ADC", "Write Initial Times", "Write Pumps Present", "HMI Command", "Save Pump Times"]
                }
              }
              n79 = Greater Or Equal To 0?(x=w286) -> (x >= 0?=w285:bool)
              n80 = Bundle By Name(cluster=w282, "HMI.HMI Mom Buttons"=T15 {"Stop"=FALSE, "Reset Timers"=FALSE, "Log Fuel Change"=FALSE, "Alarm Dismiss"=FALSE}) -> (w281:T20)
            }
            frame 28 {
              w301 = T19[] [enum."Save Alarms"] items=["Main", "Init Files", "Init", "Unused", "Save As", "Start Profile", "Check Step Time", "Alarm", "Alarm Dismiss", "Run Step", "Stop Profile", "Cycle Reset", "Time Reset", "Time Reset All", "Time Set", "Tare CTs", "Save Profile", "Open Profile", "Get Profiles", "Update Screen", "Update Controls", "Save App Config", "Write Outputs", "Disable Background", "Enable Background", "Get/Release Control", "Log Fuel Change", "Fuel Change Popup", "Read Inputs", "Remote Timer Reset", "Controller Change", "Get Alarms", "Init Alarms", "Save Alarms", "Voltage Selection", "Set Watlow Temp 1", "Set Watlow Temp 2", "Get Pressure", "Write Tare Pressure", "Adjust Controls", "Reinit ADC", "Write Initial Times", "Write Pumps Present", "HMI Command", "Save Pump Times"]
              n81 = Unbundle By Name(w299) -> ("Alarm Config"=w296:T7)
              n82 = Not Equal?(x="Alarm Config", y=w296) -> (x != y?=w300:bool)
              n83 = Bundle By Name(cluster=w298, "Alarm Config"="Alarm Config") -> (w297:T20)
            }
            frame 29 {
              w308 = T19[] [enum."Set Watlow Temp 1", enum."Save App Config"] items=["Main", "Init Files", "Init", "Unused", "Save As", "Start Profile", "Check Step Time", "Alarm", "Alarm Dismiss", "Run Step", "Stop Profile", "Cycle Reset", "Time Reset", "Time Reset All", "Time Set", "Tare CTs", "Save Profile", "Open Profile", "Get Profiles", "Update Screen", "Update Controls", "Save App Config", "Write Outputs", "Disable Background", "Enable Background", "Get/Release Control", "Log Fuel Change", "Fuel Change Popup", "Read Inputs", "Remote Timer Reset", "Controller Change", "Get Alarms", "Init Alarms", "Save Alarms", "Voltage Selection", "Set Watlow Temp 1", "Set Watlow Temp 2", "Get Pressure", "Write Tare Pressure", "Adjust Controls", "Reinit ADC", "Write Initial Times", "Write Pumps Present", "HMI Command", "Save Pump Times"]
              n84 = Unbundle By Name(w307) -> ("Tank CMDs.Temp 1 CMD"=w304:dbl)
              n85 = Not Equal?(x="Tank 1 Temp Cmd:", y=w304) -> (x != y?=w302:bool)
              n86 = Bundle By Name(cluster=w306, "Tank CMDs.Temp 1 CMD"="Tank 1 Temp Cmd:", "App Config.Temp 1"="Tank 1 Temp Cmd:") -> (w305:T20)
            }
            frame 30 {
              w315 = T19[] [enum."Set Watlow Temp 2", enum."Save App Config"] items=["Main", "Init Files", "Init", "Unused", "Save As", "Start Profile", "Check Step Time", "Alarm", "Alarm Dismiss", "Run Step", "Stop Profile", "Cycle Reset", "Time Reset", "Time Reset All", "Time Set", "Tare CTs", "Save Profile", "Open Profile", "Get Profiles", "Update Screen", "Update Controls", "Save App Config", "Write Outputs", "Disable Background", "Enable Background", "Get/Release Control", "Log Fuel Change", "Fuel Change Popup", "Read Inputs", "Remote Timer Reset", "Controller Change", "Get Alarms", "Init Alarms", "Save Alarms", "Voltage Selection", "Set Watlow Temp 1", "Set Watlow Temp 2", "Get Pressure", "Write Tare Pressure", "Adjust Controls", "Reinit ADC", "Write Initial Times", "Write Pumps Present", "HMI Command", "Save Pump Times"]
              n87 = Unbundle By Name(w314) -> ("Tank CMDs.Temp 2 CMD"=w311:dbl)
              n88 = Not Equal?(x="Tank 2 Temp Cmd:", y=w311) -> (x != y?=w309:bool)
              n89 = Bundle By Name(cluster=w313, "Tank CMDs.Temp 2 CMD"="Tank 2 Temp Cmd:", "App Config.Temp 2"="Tank 2 Temp Cmd:") -> (w312:T20)
            }
            frame 31 {
              w318 = T19[] [enum."Alarm Dismiss"] items=["Main", "Init Files", "Init", "Unused", "Save As", "Start Profile", "Check Step Time", "Alarm", "Alarm Dismiss", "Run Step", "Stop Profile", "Cycle Reset", "Time Reset", "Time Reset All", "Time Set", "Tare CTs", "Save Profile", "Open Profile", "Get Profiles", "Update Screen", "Update Controls", "Save App Config", "Write Outputs", "Disable Background", "Enable Background", "Get/Release Control", "Log Fuel Change", "Fuel Change Popup", "Read Inputs", "Remote Timer Reset", "Controller Change", "Get Alarms", "Init Alarms", "Save Alarms", "Voltage Selection", "Set Watlow Temp 1", "Set Watlow Temp 2", "Get Pressure", "Write Tare Pressure", "Adjust Controls", "Reinit ADC", "Write Initial Times", "Write Pumps Present", "HMI Command", "Save Pump Times"]
            }
            frame 32 {
              w321 = T19[] [enum."Get Pressure"] items=["Main", "Init Files", "Init", "Unused", "Save As", "Start Profile", "Check Step Time", "Alarm", "Alarm Dismiss", "Run Step", "Stop Profile", "Cycle Reset", "Time Reset", "Time Reset All", "Time Set", "Tare CTs", "Save Profile", "Open Profile", "Get Profiles", "Update Screen", "Update Controls", "Save App Config", "Write Outputs", "Disable Background", "Enable Background", "Get/Release Control", "Log Fuel Change", "Fuel Change Popup", "Read Inputs", "Remote Timer Reset", "Controller Change", "Get Alarms", "Init Alarms", "Save Alarms", "Voltage Selection", "Set Watlow Temp 1", "Set Watlow Temp 2", "Get Pressure", "Write Tare Pressure", "Adjust Controls", "Reinit ADC", "Write Initial Times", "Write Pumps Present", "HMI Command", "Save Pump Times"]
            }
            frame 33 {
              w323 = T19[] [enum."Save App Config"] items=["Main", "Init Files", "Init", "Unused", "Save As", "Start Profile", "Check Step Time", "Alarm", "Alarm Dismiss", "Run Step", "Stop Profile", "Cycle Reset", "Time Reset", "Time Reset All", "Time Set", "Tare CTs", "Save Profile", "Open Profile", "Get Profiles", "Update Screen", "Update Controls", "Save App Config", "Write Outputs", "Disable Background", "Enable Background", "Get/Release Control", "Log Fuel Change", "Fuel Change Popup", "Read Inputs", "Remote Timer Reset", "Controller Change", "Get Alarms", "Init Alarms", "Save Alarms", "Voltage Selection", "Set Watlow Temp 1", "Set Watlow Temp 2", "Get Pressure", "Write Tare Pressure", "Adjust Controls", "Reinit ADC", "Write Initial Times", "Write Pumps Present", "HMI Command", "Save Pump Times"]
              n90 = Unbundle By Name(w328) -> ("App Config.V_Run PI?"=w325:bool)
              n91 = Not Equal?(x="Closed Loop Voltage", y=w325) -> (x != y?=w324:bool)
              n92 = Bundle By Name(cluster=w327, "App Config.V_Run PI?"="Closed Loop Voltage") -> (w326:T20)
            }
            frame 34 {
              w333 = T19[] [enum."Adjust Controls", enum."Save App Config"] items=["Main", "Init Files", "Init", "Unused", "Save As", "Start Profile", "Check Step Time", "Alarm", "Alarm Dismiss", "Run Step", "Stop Profile", "Cycle Reset", "Time Reset", "Time Reset All", "Time Set", "Tare CTs", "Save Profile", "Open Profile", "Get Profiles", "Update Screen", "Update Controls", "Save App Config", "Write Outputs", "Disable Background", "Enable Background", "Get/Release Control", "Log Fuel Change", "Fuel Change Popup", "Read Inputs", "Remote Timer Reset", "Controller Change", "Get Alarms", "Init Alarms", "Save Alarms", "Voltage Selection", "Set Watlow Temp 1", "Set Watlow Temp 2", "Get Pressure", "Write Tare Pressure", "Adjust Controls", "Reinit ADC", "Write Initial Times", "Write Pumps Present", "HMI Command", "Save Pump Times"]
              n93 = Unbundle By Name(w337) -> ("App Config.Voltage Limits"=w334:T35)
              n94 = Not Equal?(x="Voltage Limits", y=w334) -> (x != y?=w330:cluster{bool, bool, bool})
              n95 = Cluster To Array(cluster=w330) -> (array=w331:bool[])
              n96 = Or Array Elements(Boolean array=w331) -> (logical OR=w329:bool)
              n97 = Bundle By Name(cluster=w336, "App Config.Voltage Limits"="Voltage Limits") -> (w335:T20)
            }
            frame 35 {
              w338 = T19[] [enum."Adjust Controls", enum."Save App Config"] items=["Main", "Init Files", "Init", "Unused", "Save As", "Start Profile", "Check Step Time", "Alarm", "Alarm Dismiss", "Run Step", "Stop Profile", "Cycle Reset", "Time Reset", "Time Reset All", "Time Set", "Tare CTs", "Save Profile", "Open Profile", "Get Profiles", "Update Screen", "Update Controls", "Save App Config", "Write Outputs", "Disable Background", "Enable Background", "Get/Release Control", "Log Fuel Change", "Fuel Change Popup", "Read Inputs", "Remote Timer Reset", "Controller Change", "Get Alarms", "Init Alarms", "Save Alarms", "Voltage Selection", "Set Watlow Temp 1", "Set Watlow Temp 2", "Get Pressure", "Write Tare Pressure", "Adjust Controls", "Reinit ADC", "Write Initial Times", "Write Pumps Present", "HMI Command", "Save Pump Times"]
              n98 = Unbundle By Name(w346) -> ("App Config.Voltage Far PI"=w343:T36)
              n99 = Not Equal?(x="Far PI", y=w343) -> (x != y?=w340:cluster{bool, bool, bool})
              n100 = Cluster To Array(cluster=w340) -> (array=w341:bool[])
              n101 = Or Array Elements(Boolean array=w341) -> (logical OR=w339:bool)
              n102 = Bundle By Name(cluster=w345, "App Config.Voltage Far PI"="Far PI") -> (w344:T20)
            }
            frame 36 {
              w347 = T19[] [enum."Adjust Controls", enum."Save App Config"] items=["Main", "Init Files", "Init", "Unused", "Save As", "Start Profile", "Check Step Time", "Alarm", "Alarm Dismiss", "Run Step", "Stop Profile", "Cycle Reset", "Time Reset", "Time Reset All", "Time Set", "Tare CTs", "Save Profile", "Open Profile", "Get Profiles", "Update Screen", "Update Controls", "Save App Config", "Write Outputs", "Disable Background", "Enable Background", "Get/Release Control", "Log Fuel Change", "Fuel Change Popup", "Read Inputs", "Remote Timer Reset", "Controller Change", "Get Alarms", "Init Alarms", "Save Alarms", "Voltage Selection", "Set Watlow Temp 1", "Set Watlow Temp 2", "Get Pressure", "Write Tare Pressure", "Adjust Controls", "Reinit ADC", "Write Initial Times", "Write Pumps Present", "HMI Command", "Save Pump Times"]
              n103 = Unbundle By Name(w355) -> ("App Config.Voltage Mid PI"=w352:T37)
              n104 = Not Equal?(x="Mid PI", y=w352) -> (x != y?=w350:cluster{bool, bool, bool})
              n105 = Cluster To Array(cluster=w350) -> (array=w351:bool[])
              n106 = Or Array Elements(Boolean array=w351) -> (logical OR=w349:bool)
              n107 = Bundle By Name(cluster=w354, "App Config.Voltage Mid PI"="Mid PI") -> (w353:T20)
            }
            frame 37 {
              w356 = T19[] [enum."Adjust Controls", enum."Save App Config"] items=["Main", "Init Files", "Init", "Unused", "Save As", "Start Profile", "Check Step Time", "Alarm", "Alarm Dismiss", "Run Step", "Stop Profile", "Cycle Reset", "Time Reset", "Time Reset All", "Time Set", "Tare CTs", "Save Profile", "Open Profile", "Get Profiles", "Update Screen", "Update Controls", "Save App Config", "Write Outputs", "Disable Background", "Enable Background", "Get/Release Control", "Log Fuel Change", "Fuel Change Popup", "Read Inputs", "Remote Timer Reset", "Controller Change", "Get Alarms", "Init Alarms", "Save Alarms", "Voltage Selection", "Set Watlow Temp 1", "Set Watlow Temp 2", "Get Pressure", "Write Tare Pressure", "Adjust Controls", "Reinit ADC", "Write Initial Times", "Write Pumps Present", "HMI Command", "Save Pump Times"]
              n108 = Unbundle By Name(w364) -> ("App Config.Voltage Close PI"=w361:T38)
              n109 = Not Equal?(x="Close PI", y=w361) -> (x != y?=w359:cluster{bool, bool, bool})
              n110 = Cluster To Array(cluster=w359) -> (array=w360:bool[])
              n111 = Or Array Elements(Boolean array=w360) -> (logical OR=w358:bool)
              n112 = Bundle By Name(cluster=w363, "App Config.Voltage Close PI"="Close PI") -> (w362:T20)
            }
            frame 38 {
              w365 = T19[] [enum."Adjust Controls", enum."Save App Config"] items=["Main", "Init Files", "Init", "Unused", "Save As", "Start Profile", "Check Step Time", "Alarm", "Alarm Dismiss", "Run Step", "Stop Profile", "Cycle Reset", "Time Reset", "Time Reset All", "Time Set", "Tare CTs", "Save Profile", "Open Profile", "Get Profiles", "Update Screen", "Update Controls", "Save App Config", "Write Outputs", "Disable Background", "Enable Background", "Get/Release Control", "Log Fuel Change", "Fuel Change Popup", "Read Inputs", "Remote Timer Reset", "Controller Change", "Get Alarms", "Init Alarms", "Save Alarms", "Voltage Selection", "Set Watlow Temp 1", "Set Watlow Temp 2", "Get Pressure", "Write Tare Pressure", "Adjust Controls", "Reinit ADC", "Write Initial Times", "Write Pumps Present", "HMI Command", "Save Pump Times"]
              n113 = Unbundle By Name(w373) -> ("App Config.Voltage Scale"=w370:cluster{"V_FFm":dbl, "V_FFb":dbl})
              n114 = Not Equal?(x="Voltage Scale", y=w370) -> (x != y?=w368:cluster{bool, bool})
              n115 = Cluster To Array(cluster=w368) -> (array=w367:bool[])
              n116 = Or Array Elements(Boolean array=w367) -> (logical OR=w366:bool)
              n117 = Bundle By Name(cluster=w372, "App Config.Voltage Scale"="Voltage Scale") -> (w371:T20)
            }
            frame 39 {
              w374 = T19[] [enum."Adjust Controls", enum."Save App Config"] items=["Main", "Init Files", "Init", "Unused", "Save As", "Start Profile", "Check Step Time", "Alarm", "Alarm Dismiss", "Run Step", "Stop Profile", "Cycle Reset", "Time Reset", "Time Reset All", "Time Set", "Tare CTs", "Save Profile", "Open Profile", "Get Profiles", "Update Screen", "Update Controls", "Save App Config", "Write Outputs", "Disable Background", "Enable Background", "Get/Release Control", "Log Fuel Change", "Fuel Change Popup", "Read Inputs", "Remote Timer Reset", "Controller Change", "Get Alarms", "Init Alarms", "Save Alarms", "Voltage Selection", "Set Watlow Temp 1", "Set Watlow Temp 2", "Get Pressure", "Write Tare Pressure", "Adjust Controls", "Reinit ADC", "Write Initial Times", "Write Pumps Present", "HMI Command", "Save Pump Times"]
              n118 = Unbundle By Name(w382) -> ("App Config.Voltage Cutoffs"=w379:cluster{"V_MidCutoff":dbl, "V_CloseCutoff":dbl})
              n119 = Not Equal?(x="Cutoffs", y=w379) -> (x != y?=w378:cluster{bool, bool})
              n120 = Cluster To Array(cluster=w378) -> (array=w377:bool[])
              n121 = Or Array Elements(Boolean array=w377) -> (logical OR=w376:bool)
              n122 = Bundle By Name(cluster=w381, "App Config.Voltage Cutoffs"="Cutoffs") -> (w380:T20)
            }
            frame 40 {
              w387 = T19[] [enum."Save App Config"] items=["Main", "Init Files", "Init", "Unused", "Save As", "Start Profile", "Check Step Time", "Alarm", "Alarm Dismiss", "Run Step", "Stop Profile", "Cycle Reset", "Time Reset", "Time Reset All", "Time Set", "Tare CTs", "Save Profile", "Open Profile", "Get Profiles", "Update Screen", "Update Controls", "Save App Config", "Write Outputs", "Disable Background", "Enable Background", "Get/Release Control", "Log Fuel Change", "Fuel Change Popup", "Read Inputs", "Remote Timer Reset", "Controller Change", "Get Alarms", "Init Alarms", "Save Alarms", "Voltage Selection", "Set Watlow Temp 1", "Set Watlow Temp 2", "Get Pressure", "Write Tare Pressure", "Adjust Controls", "Reinit ADC", "Write Initial Times", "Write Pumps Present", "HMI Command", "Save Pump Times"]
              n123 = Unbundle By Name(w391) -> ("App Config.Pressure Scale"=w388:cluster{"Pres_FFm":dbl, "Pres_FFb":dbl})
              n124 = Not Equal?(x="Pressure Scale", y=w388) -> (x != y?=w386:cluster{bool, bool})
              n125 = Cluster To Array(cluster=w386) -> (array=w385:bool[])
              n126 = Or Array Elements(Boolean array=w385) -> (logical OR=w384:bool)
              n127 = Bundle By Name(cluster=w390, "App Config.Pressure Scale"="Pressure Scale") -> (w389:T20)
            }
            frame 41 {
              w395 = T19[] [enum."Save App Config"] items=["Main", "Init Files", "Init", "Unused", "Save As", "Start Profile", "Check Step Time", "Alarm", "Alarm Dismiss", "Run Step", "Stop Profile", "Cycle Reset", "Time Reset", "Time Reset All", "Time Set", "Tare CTs", "Save Profile", "Open Profile", "Get Profiles", "Update Screen", "Update Controls", "Save App Config", "Write Outputs", "Disable Background", "Enable Background", "Get/Release Control", "Log Fuel Change", "Fuel Change Popup", "Read Inputs", "Remote Timer Reset", "Controller Change", "Get Alarms", "Init Alarms", "Save Alarms", "Voltage Selection", "Set Watlow Temp 1", "Set Watlow Temp 2", "Get Pressure", "Write Tare Pressure", "Adjust Controls", "Reinit ADC", "Write Initial Times", "Write Pumps Present", "HMI Command", "Save Pump Times"]
              n128 = Unbundle By Name(w399) -> ("App Config.Temp Format"=w396:i32)
              n129 = To Long Integer(number="Thermocouple") -> (32bit integer=w392:i32)
              n130 = Not Equal?(x=w392, y=w396) -> (x != y?=w394:bool)
              n131 = Bundle By Name(cluster=w398, "App Config.Temp Format"=w392) -> (w397:T20)
            }
            frame 42 {
              w402 = T19[] [enum."Save App Config"] items=["Main", "Init Files", "Init", "Unused", "Save As", "Start Profile", "Check Step Time", "Alarm", "Alarm Dismiss", "Run Step", "Stop Profile", "Cycle Reset", "Time Reset", "Time Reset All", "Time Set", "Tare CTs", "Save Profile", "Open Profile", "Get Profiles", "Update Screen", "Update Controls", "Save App Config", "Write Outputs", "Disable Background", "Enable Background", "Get/Release Control", "Log Fuel Change", "Fuel Change Popup", "Read Inputs", "Remote Timer Reset", "Controller Change", "Get Alarms", "Init Alarms", "Save Alarms", "Voltage Selection", "Set Watlow Temp 1", "Set Watlow Temp 2", "Get Pressure", "Write Tare Pressure", "Adjust Controls", "Reinit ADC", "Write Initial Times", "Write Pumps Present", "HMI Command", "Save Pump Times"]
              n132 = Unbundle By Name(w406) -> ("App Config.Temp Tolerance"=w403:dbl)
              n133 = Not Equal?(x="Temp Tolerance", y=w403) -> (x != y?=w400:bool)
              n134 = Bundle By Name(cluster=w405, "App Config.Temp Tolerance"="Temp Tolerance") -> (w404:T20)
            }
            frame 43 {
              w413 = T19[] [enum."Save App Config"] items=["Main", "Init Files", "Init", "Unused", "Save As", "Start Profile", "Check Step Time", "Alarm", "Alarm Dismiss", "Run Step", "Stop Profile", "Cycle Reset", "Time Reset", "Time Reset All", "Time Set", "Tare CTs", "Save Profile", "Open Profile", "Get Profiles", "Update Screen", "Update Controls", "Save App Config", "Write Outputs", "Disable Background", "Enable Background", "Get/Release Control", "Log Fuel Change", "Fuel Change Popup", "Read Inputs", "Remote Timer Reset", "Controller Change", "Get Alarms", "Init Alarms", "Save Alarms", "Voltage Selection", "Set Watlow Temp 1", "Set Watlow Temp 2", "Get Pressure", "Write Tare Pressure", "Adjust Controls", "Reinit ADC", "Write Initial Times", "Write Pumps Present", "HMI Command", "Save Pump Times"]
              n135 = Unbundle By Name(w410) -> ("App Config.Target Voltage"=w409:dbl)
              n136 = Not Equal?(x=w409, y="Target Voltage:") -> (x != y?=w408:bool)
              n137 = Bundle By Name(cluster=w412, "App Config.Target Voltage"="Target Voltage:") -> (w411:T20)
            }
            frame 44 {
              w420 = T19[] [enum."Save App Config"] items=["Main", "Init Files", "Init", "Unused", "Save As", "Start Profile", "Check Step Time", "Alarm", "Alarm Dismiss", "Run Step", "Stop Profile", "Cycle Reset", "Time Reset", "Time Reset All", "Time Set", "Tare CTs", "Save Profile", "Open Profile", "Get Profiles", "Update Screen", "Update Controls", "Save App Config", "Write Outputs", "Disable Background", "Enable Background", "Get/Release Control", "Log Fuel Change", "Fuel Change Popup", "Read Inputs", "Remote Timer Reset", "Controller Change", "Get Alarms", "Init Alarms", "Save Alarms", "Voltage Selection", "Set Watlow Temp 1", "Set Watlow Temp 2", "Get Pressure", "Write Tare Pressure", "Adjust Controls", "Reinit ADC", "Write Initial Times", "Write Pumps Present", "HMI Command", "Save Pump Times"]
              n138 = Unbundle By Name(w417) -> ("App Config.Target Pressure"=w416:dbl)
              n139 = Not Equal?(x=w416, y="Target Pressure:") -> (x != y?=w415:bool)
              n140 = Bundle By Name(cluster=w419, "App Config.Target Pressure"="Target Pressure:") -> (w418:T20)
            }
            frame 45 {
              w424 = T19[] [enum."HMI Command"] items=["Main", "Init Files", "Init", "Unused", "Save As", "Start Profile", "Check Step Time", "Alarm", "Alarm Dismiss", "Run Step", "Stop Profile", "Cycle Reset", "Time Reset", "Time Reset All", "Time Set", "Tare CTs", "Save Profile", "Open Profile", "Get Profiles", "Update Screen", "Update Controls", "Save App Config", "Write Outputs", "Disable Background", "Enable Background", "Get/Release Control", "Log Fuel Change", "Fuel Change Popup", "Read Inputs", "Remote Timer Reset", "Controller Change", "Get Alarms", "Init Alarms", "Save Alarms", "Voltage Selection", "Set Watlow Temp 1", "Set Watlow Temp 2", "Get Pressure", "Write Tare Pressure", "Adjust Controls", "Reinit ADC", "Write Initial Times", "Write Pumps Present", "HMI Command", "Save Pump Times"]
              n141 = call "RPi HMI Global.vi"() -> ("HMI Cluster OUT"=w423:T10)  [unwired: 11 in]
              n142 = Unbundle By Name(w423) -> ("HMI Command"=w421:bool)
            }
            frame 46 {
              w431 = T19[] [enum."Update Controls"] items=["Main", "Init Files", "Init", "Unused", "Save As", "Start Profile", "Check Step Time", "Alarm", "Alarm Dismiss", "Run Step", "Stop Profile", "Cycle Reset", "Time Reset", "Time Reset All", "Time Set", "Tare CTs", "Save Profile", "Open Profile", "Get Profiles", "Update Screen", "Update Controls", "Save App Config", "Write Outputs", "Disable Background", "Enable Background", "Get/Release Control", "Log Fuel Change", "Fuel Change Popup", "Read Inputs", "Remote Timer Reset", "Controller Change", "Get Alarms", "Init Alarms", "Save Alarms", "Voltage Selection", "Set Watlow Temp 1", "Set Watlow Temp 2", "Get Pressure", "Write Tare Pressure", "Adjust Controls", "Reinit ADC", "Write Initial Times", "Write Pumps Present", "HMI Command", "Save Pump Times"]
              n143 = Unbundle By Name(w430) -> ("Email Alarms Disabled"=w427:bool)
              n144 = Greater?(x="Disable Alarm Email", y=w427) -> (0:w425:bool)
              n145 = Bundle By Name(cluster=w429, "Email Alarms Disabled"="Disable Alarm Email") -> (w428:T20)
            }
            frame 47 {
              w436 = T19[] [] items=["Main", "Init Files", "Init", "Unused", "Save As", "Start Profile", "Check Step Time", "Alarm", "Alarm Dismiss", "Run Step", "Stop Profile", "Cycle Reset", "Time Reset", "Time Reset All", "Time Set", "Tare CTs", "Save Profile", "Open Profile", "Get Profiles", "Update Screen", "Update Controls", "Save App Config", "Write Outputs", "Disable Background", "Enable Background", "Get/Release Control", "Log Fuel Change", "Fuel Change Popup", "Read Inputs", "Remote Timer Reset", "Controller Change", "Get Alarms", "Init Alarms", "Save Alarms", "Voltage Selection", "Set Watlow Temp 1", "Set Watlow Temp 2", "Get Pressure", "Write Tare Pressure", "Adjust Controls", "Reinit ADC", "Write Initial Times", "Write Pumps Present", "HMI Command", "Save Pump Times"]
              n146 = Bundle By Name(cluster=w435, "Concat Data"="Concat Data") -> (w434:T20)
            }
            frame 48 {
              w441 = T19[] [] items=["Main", "Init Files", "Init", "Unused", "Save As", "Start Profile", "Check Step Time", "Alarm", "Alarm Dismiss", "Run Step", "Stop Profile", "Cycle Reset", "Time Reset", "Time Reset All", "Time Set", "Tare CTs", "Save Profile", "Open Profile", "Get Profiles", "Update Screen", "Update Controls", "Save App Config", "Write Outputs", "Disable Background", "Enable Background", "Get/Release Control", "Log Fuel Change", "Fuel Change Popup", "Read Inputs", "Remote Timer Reset", "Controller Change", "Get Alarms", "Init Alarms", "Save Alarms", "Voltage Selection", "Set Watlow Temp 1", "Set Watlow Temp 2", "Get Pressure", "Write Tare Pressure", "Adjust Controls", "Reinit ADC", "Write Initial Times", "Write Pumps Present", "HMI Command", "Save Pump Times"]
              n147 = Bundle By Name(cluster=w440, "WebDAV Push"="WebDAV Push") -> (w439:T20)
            }
          }
        }
        n148 = Tick Count (ms)() -> (millisecond timer value=w80:u32)
        n149 = Subtract(x=w80, y=w82) -> (x-y=w79:u32)
        n150 = Subtract(x=w80, y=w81) -> (x-y=w78:u32)
        n151 = Greater?(x=w79, y=u32 100) -> (0:w74:bool)
        n152 = Greater?(x=w78, y=u32 500) -> (0:w73:bool)
        n153 = case shown="True" w73 {
          tunnel: w83 -> [w97 w101]
          tunnel: Sequence_States."Update Screen" -> [_ w100]
          tunnel: [w97 w98] -> w85
          frame False {
          }
          frame True {
            n154 = Insert Into Array(array=w101, index=0, new element=w100) -> (w98:T19[])
          }
        }
        n155 = case shown="True" w74 {
          tunnel: w85 -> [w102 w106]
          tunnel: Sequence_States."Read Inputs" -> [_ w105]
          tunnel: [w102 w103] -> w88
          frame False {
          }
          frame True {
            n156 = Insert Into Array(array=w106, index=0, new element=w105) -> (w103:T19[])
          }
        }
        n157 = case shown="True" w75 {
          tunnel: w88 -> [w107 w111]
          tunnel: Sequence_States."Check Step Time" -> [_ w110]
          tunnel: [w107 w108] -> w89
          frame False {
          }
          frame True {
            n158 = Insert Into Array(array=w111, index=0, new element=w110) -> (w108:T19[])
          }
        }
        n159 = case shown="True" w91 {
          tunnel: w89 -> [w112 w116]
          tunnel: w92 -> [_ w115]
          tunnel: [w112 w113] -> w90
          frame False {
          }
          frame True {
            n160 = Insert Into Array(array=w116, index=0, new element=w115) -> (w113:T19[])
          }
        }
      }
      frame "Init Files" {
        w461 = T19[] [enum."Write Tare Pressure", enum."Write Initial Times", enum."Write Pumps Present"] items=["Main", "Init Files", "Init", "Unused", "Save As", "Start Profile", "Check Step Time", "Alarm", "Alarm Dismiss", "Run Step", "Stop Profile", "Cycle Reset", "Time Reset", "Time Reset All", "Time Set", "Tare CTs", "Save Profile", "Open Profile", "Get Profiles", "Update Screen", "Update Controls", "Save App Config", "Write Outputs", "Disable Background", "Enable Background", "Get/Release Control", "Log Fuel Change", "Fuel Change Popup", "Read Inputs", "Remote Timer Reset", "Controller Change", "Get Alarms", "Init Alarms", "Save Alarms", "Voltage Selection", "Set Watlow Temp 1", "Set Watlow Temp 2", "Get Pressure", "Write Tare Pressure", "Adjust Controls", "Reinit ADC", "Write Initial Times", "Write Pumps Present", "HMI Command", "Save Pump Times"]
        w470 = dbl[][] [[0.0, 11.0, 0.0, 0.0, 0.0], [0.0, 11.0, 0.0, 0.0, 0.0], [0.0, 11.0, 0.0, 0.0, 0.0], [0.0, 11.0, 0.0, 0.0, 0.0], [0.0, 11.0, 0.0, 0.0, 0.0], [0.0, 11.0, 0.0, 0.0, 0.0], [0.0, 1.0, 0.0, 0.0, 0.0], [0.0, 1.0, 0.0, 0.0, 0.0], [0.0, 1.0, 0.0, 0.0, 0.0], [0.0, 2.0, 0.0, 0.0, 0.0], [0.0, 1.0, 0.0, 0.0, 0.0], [0.0, 1.0, 0.0, 0.0, 0.0], [0.0, 1.0, 0.0, 0.0, 0.0], [0.0, 1.0, 0.0, 0.0, 0.0], [0.0, 1.0, 0.0, 0.0, 0.0], [0.0, 1.0, 0.0, 0.0, 0.0], [0.0, 1.0, 0.0, 0.0, 0.0], [0.0, 1.0, 0.0, 0.0, 0.0], [0.0, 1.0, 0.0, 0.0, 0.0], [0.0, 1.0, 0.0, 0.0, 0.0], [0.0, 1.0, 0.0, 0.0, 0.0], [0.0, 1.0, 0.0, 0.0, 0.0], [-60.0, 24.0, 0.0, 0.0, 0.0], [-60.0, 24.0, 0.0, 0.0, 0.0], [-60.0, 24.0, 0.0, 0.0, 0.0], [-60.0, 24.0, 0.0, 0.0, 0.0], [-60.0, 24.0, 0.0, 0.0, 0.0], [-60.0, 24.0, 0.0, 0.0, 0.0], [-660.0, 200.0, 0.0, 0.0, 0.0], [-660.0, 200.0, 0.0, 0.0, 0.0], [-258.5, 258.5, 0.0, 0.0, 0.0], [-258.5, 258.5, 0.0, 0.0, 0.0], [-258.5, 258.5, 0.0, 0.0, 0.0], [-258.5, 258.5, 0.0, 0.0, 0.0], [-258.5, 258.5, 0.0, 0.0, 0.0], [-258.5, 258.5, 0.0, 0.0, 0.0], [-150.0, 150.0, 0.0, 0.0, 0.0], [-150.0, 150.0, 0.0, 0.0, 0.0], [-150.0, 150.0, 0.0, 0.0, 0.0], [-150.0, 150.0, 0.0, 0.0, 0.0], [-150.0, 150.0, 0.0, 0.0, 0.0], [-150.0, 150.0, 0.0, 0.0, 0.0], [0.0, 1.0, 0.0, 0.0, 0.0], [0.0, 1.0, 0.0, 0.0, 0.0], [0.0, 1.0, 0.0, 0.0, 0.0], [0.0, 1.0, 0.0, 0.0, 0.0], [0.0, 1.0, 0.0, 0.0, 0.0], [0.0, 1.0, 0.0, 0.0, 0.0], [0.0, 11.0, 0.0, 0.0, 0.0], [0.0, 11.0, 0.0, 0.0, 0.0], [0.0, 11.0, 0.0, 0.0, 0.0], [0.0, 11.0, 0.0, 0.0, 0.0], [0.0, 11.0, 0.0, 0.0, 0.0], [0.0, 11.0, 0.0, 0.0, 0.0], [0.0, 0.0001, 0.0, 0.0, 0.0], [0.0, 0.0001, 0.0, 0.0, 0.0], [0.0, 0.0001, 0.0, 0.0, 0.0], [0.0, 0.0001, 0.0, 0.0, 0.0], [0.0, 0.0001, 0.0, 0.0, 0.0], [0.0, 0.0001, 0.0, 0.0, 0.0]]  # Cal Coefficients
        # "This is 10.30.189.0"
        n161 = Unbundle By Name(w479) -> ("App Config"=w464:T1)
        n162 = String To IP() -> (0:w474:u32)  [unwired: 1 in]
        n163 = Subtract(x=w474, y=u32 169786624) -> (x-y=w442:u32)
        n164 = call <vilib>:"Open Config Data.vi"("configuration file path"=path "c:/App Config.ini") -> ("error out"=w486:errorcluster, "file created?"=w484:bool, "refnum"=w487:T39)  [unwired: 8 in]
        n165 = Number To Decimal String(number=w442) -> (decimal integer string=w473:string)  [unwired: 1 in]
        n166 = case shown="False" w484 {
          tunnel: w487 -> [w518 w523]
          tunnel: w486 -> [w516 w521]
          tunnel: w464 -> [w513 w520]
          tunnel: [w514 w520] -> w444
          tunnel: [w512 w522] -> w447
          frame False {
            # "Read App Config.ini"
            n167 = call "Read Write App Config.vi"("Error IN"=w516, "App Config"=w513, "Refnum in"=w518) -> ("Error OUT"=w515:errorcluster, "App Config OUT"=w514:T1, "Refnum out"=w517:T39)  [unwired: 6 in]
            n168 = call <vilib>:"Close Config Data.vi"("error in (no error)"=w515, "refnum"=w517) -> ("error out"=w519:errorcluster)  [unwired: 8 in, 1 out]
            n169 = call <vilib>:"Clear Errors.vi"("error in (no error)"=w519) -> ("error out"=w512:errorcluster)  [unwired: 6 in]
          }
          frame True {
            # "Doesn't exists, so create."
            n170 = call "Read Write App Config.vi"("Write (F)"=TRUE, "Error IN"=w521, "App Config"=w520, "Refnum in"=w523) -> ("Error OUT"=w525:errorcluster, "Refnum out"=w526:T39)  [unwired: 5 in, 1 out]
            n171 = call <vilib>:"Close Config Data.vi"("error in (no error)"=w525, "refnum"=w526) -> ("error out"=w522:errorcluster)  [unwired: 8 in, 1 out]
          }
        }
        n172 = Concatenate Strings("/c/" ("string"), w473, ".cal" ("string")) -> (w465:string)
        n173 = String To Path(string=w465) -> (path=w466:path)
        n174 = Bundle By Name(cluster=w444, "Data Log Init.IP Last 3"=w442) -> (w443:T1)
        n175 = Unbundle By Name(w443) -> ("Data Log Init"=w445:T3)
        n176 = call "Get Elapsed Times.vi"("Error In"=w447, "Path"=path "c:/ElapsedTimes" ("file (use dialog)")) -> ("Error Out"=w468:errorcluster, "Elapsed Times"=w480:dbl[])  [unwired: 8 in]
        n177 = call "Data Logger Main.vi"("Data Logger Mode"=Data_Logger_Mode."Init", "Data Log Init"=w445) -> ()  [unwired: 18 in]
        n178 = Unbundle By Name(w443) -> ("Voltage Limits"=w450:T35, "Voltage Far PI"=w457:T36, "Voltage Mid PI"=w456:T37, "Voltage Close PI"=w455:T38, "Voltage Scale"=w454:cluster{"V_FFm":dbl, "V_FFb":dbl}, "Voltage Cutoffs"=w453:cluster{"V_MidCutoff":dbl, "V_CloseCutoff":dbl}, "Pressure Scale"=w452:cluster{"Pres_FFm":dbl, "Pres_FFb":dbl}, "Temp Format"=w449:i32, "Temp Tolerance"=w448:dbl)
        n179 = call <vilib>:"Clear Errors.vi"("error in (no error)"=w468) -> ("error out"=w469:errorcluster)  [unwired: 6 in]
        n180 = call "Get Pressure Offsets.vi"("Error In"=w469, "Path"=path "c:/PressureOffsets" ("file (use dialog)")) -> ("Error Out"=w467:errorcluster, "Pressure Offsets"=w481:dbl[])  [unwired: 8 in]
        n181 = call <vilib>:"Clear Errors.vi"("error in (no error)"=w467) -> ("error out"=w459:errorcluster)  [unwired: 6 in]
        n182 = call "Get Cal Coefficients.vi"("Error In"=w459, "Path"=w466) -> ("Error"=w476:bool, "Cal Coefficients"=w477:dbl[][])  [unwired: 7 in, 1 out]
        n183 = case shown="False" w476 {
          tunnel: w477 -> [_ w491]
          tunnel: [w488 w490] -> w451
          tunnel: w470 -> [w488 w489]
          frame True {
          }
          frame False {
            n184 = for {
              tunnel: w491 -> [w493] mode=indexing
              shift-right: [w494] -> w490
              shift-left: w489 -> [w495]
              i -> [w492]
              n185 = Index Array(array=w493) -> (element #1=w506:dbl, element #2=w505:dbl, element #3=w504:dbl, element #4=w500:dbl, element #5=w499:dbl)  [unwired: 5 in]
              n186 = Equal To 0?(x=w506) -> (x = 0?=w503:bool)
              n187 = Equal To 0?(x=w505) -> (x = 0?=w502:bool)
              n188 = Equal To 0?(x=w504) -> (x = 0?=w501:bool)
              n189 = Equal To 0?(x=w500) -> (x = 0?=w498:bool)
              n190 = Equal To 0?(x=w499) -> (x = 0?=w497:bool)
              n191 = Compound Arithmetic op=AND(w503, w502, w501, w498, w497) -> (w496:bool)
              n192 = case shown="False" w496 {
                tunnel: w495 -> [w510 w511]
                tunnel: [w509 w511] -> w494
                tunnel: w493 -> [w508 _]
                tunnel: w492 -> [w507 _]
                frame False {
                  n193 = Replace Array Subset(array=w510, new element=w508, index (row)=w507) -> (w509:dbl[][])  [unwired: 1 in]
                }
                frame True {
                }
              }
            }
          }
        }
        n194 = local write "Voltage Limits"(w450) -> ()
        n195 = local write "Far PI"(w457) -> ()
        n196 = local write "Mid PI"(w456) -> ()
        n197 = local write "Close PI"(w455) -> ()
        n198 = local write "Voltage Scale"(w454) -> ()
        n199 = local write "Cutoffs"(w453) -> ()
        n200 = local write "Pressure Scale"(w452) -> ()
        n201 = local write "Thermocouple"(w449) -> ()
        n202 = local write "Temp Tolerance"(w448) -> ()
        n203 = call "PI with FF.vi"("Cutoffs"=w453, "FFcluster"=w454, "ClosePIcluster"=w455, "MidPIcluster"=w456, "FarPIcluster"=w457, "LimitCluster"=w450, "Init (F)"=TRUE) -> ()  [unwired: 8 in, 1 out]
        n204 = Insert Into Array(array=w460, index=0, new element=w461) -> (w462:T19[])
        n205 = Bundle By Name(cluster=w479, "App Config"=w443, "Initial Times"=w480, "Pressure Offsets"=w481, "CalArray"=w451) -> (w478:T20)
      }
      frame "Init" {
        w536 = T40 [{"Controller Name"=enum."Kuhnke", "CommSeg"=1, "PWM?"=TRUE, "Frequency"=100, "Low Command"=10.0, "High Command"=100.0, "Stop Command"=10.0, "Command Step"=0.1, "Solenoid Stop?"=FALSE, "Controller?"=TRUE, "Invert PWM"=TRUE}, {"Controller Name"=enum."Helbako BLDC", "CommSeg"=1, "PWM?"=TRUE, "Frequency"=100, "Low Command"=10.0, "High Command"=100.0, "Stop Command"=10.0, "Command Step"=0.1, "Solenoid Stop?"=FALSE, "Controller?"=TRUE, "Invert PWM"=TRUE}, {"Controller Name"=enum."Conti", "CommSeg"=1, "PWM?"=FALSE, "Frequency"=100, "Low Command"=0.0, "High Command"=800.0, "Stop Command"=0.0, "Command Step"=1.0, "Solenoid Stop?"=FALSE, "Controller?"=TRUE, "Invert PWM"=FALSE}, {"Controller Name"=enum."Hella BLDC OL PWM", "CommSeg"=1, "PWM?"=FALSE, "Frequency"=100, "Low Command"=0.0, "High Command"=100.0, "Stop Command"=0.0, "Command Step"=0.1, "Solenoid Stop?"=FALSE, "Controller?"=TRUE, "Invert PWM"=FALSE}, {"Controller Name"=enum."Hella BLDC Turbine OL PWM", "CommSeg"=1, "PWM?"=FALSE, "Frequency"=100, "Low Command"=0.0, "High Command"=100.0, "Stop Command"=0.0, "Command Step"=0.1, "Solenoid Stop?"=FALSE, "Controller?"=TRUE, "Invert PWM"=FALSE}, {"Controller Name"=enum."Hella BLDC Pressure", "CommSeg"=1, "PWM?"=FALSE, "Frequency"=100, "Low Command"=0.0, "High Command"=100.0, "Stop Command"=0.0, "Command Step"=0.1, "Solenoid Stop?"=FALSE, "Controller?"=TRUE, "Invert PWM"=FALSE}, {"Controller Name"=enum."Helbako (old)", "CommSeg"=1, "PWM?"=FALSE, "Frequency"=100, "Low Command"=0.0, "High Command"=100.0, "Stop Command"=0.0, "Command Step"=0.1, "Solenoid Stop?"=FALSE, "Controller?"=TRUE, "Invert PWM"=FALSE}, {"Controller Name"=enum."TI PWM", "CommSeg"=1, "PWM?"=TRUE, "Frequency"=100, "Low Command"=0.0, "High Command"=100.0, "Stop Command"=0.0, "Command Step"=0.1, "Solenoid Stop?"=FALSE, "Controller?"=TRUE, "Invert PWM"=FALSE}, {"Controller Name"=enum."PSA", "CommSeg"=1, "PWM?"=TRUE, "Frequency"=100, "Low Command"=5.0, "High Command"=95.0, "Stop Command"=5.0, "Command Step"=0.1, "Solenoid Stop?"=FALSE, "Controller?"=TRUE, "Invert PWM"=FALSE}, {"Controller Name"=enum."Hella Gas", "CommSeg"=1, "PWM?"=FALSE, "Frequency"=100, "Low Command"=0.0, "High Command"=800.0, "Stop Command"=0.0, "Command Step"=1.0, "Solenoid Stop?"=TRUE, "Controller?"=TRUE, "Invert PWM"=FALSE}, {"Controller Name"=enum."Hella Diesel", "CommSeg"=1, "PWM?"=FALSE, "Frequency"=100, "Low Command"=370.0, "High Command"=461.0, "Stop Command"=370.0, "Command Step"=1.0, "Solenoid Stop?"=TRUE, "Controller?"=TRUE, "Invert PWM"=FALSE}, {"Controller Name"=enum."8 Comm", "CommSeg"=4, "PWM?"=FALSE, "Frequency"=100, "Low Command"=0.0, "High Command"=1.0, "Stop Command"=0.0, "Command Step"=1.0, "Solenoid Stop?"=FALSE, "Controller?"=FALSE, "Invert PWM"=FALSE}, {"Controller Name"=enum."10 Comm", "CommSeg"=5, "PWM?"=FALSE, "Frequency"=100, "Low Command"=0.0, "High Command"=1.0, "Stop Command"=0.0, "Command Step"=1.0, "Solenoid Stop?"=FALSE, "Controller?"=FALSE, "Invert PWM"=FALSE}, {"Controller Name"=enum."8 Comm Hella", "CommSeg"=4, "PWM?"=TRUE, "Frequency"=150, "Low Command"=0.0, "High Command"=50.0, "Stop Command"=80.0, "Command Step"=0.1, "Solenoid Stop?"=FALSE, "Controller?"=TRUE, "Invert PWM"=FALSE}, {"Controller Name"=enum."10 Comm Hella", "CommSeg"=5, "PWM?"=TRUE, "Frequency"=150, "Low Command"=0.0, "High Command"=50.0, "Stop Command"=80.0, "Command Step"=0.1, "Solenoid Stop?"=FALSE, "Controller?"=TRUE, "Invert PWM"=FALSE}, {"Controller Name"=enum."8 Comm Omron", "CommSeg"=4, "PWM?"=TRUE, "Frequency"=150, "Low Command"=5.0, "High Command"=50.0, "Stop Command"=75.0, "Command Step"=0.1, "Solenoid Stop?"=FALSE, "Controller?"=TRUE, "Invert PWM"=FALSE}, {"Controller Name"=enum."10 Comm Omron", "CommSeg"=5, "PWM?"=TRUE, "Frequency"=150, "Low Command"=5.0, "High Command"=50.0, "Stop Command"=75.0, "Command Step"=0.1, "Solenoid Stop?"=FALSE, "Controller?"=TRUE, "Invert PWM"=FALSE}, {"Controller Name"=enum."8 Comm Nissan", "CommSeg"=4, "PWM?"=TRUE, "Frequency"=10, "Low Command"=50.0, "High Command"=90.0, "Stop Command"=50.0, "Command Step"=0.1, "Solenoid Stop?"=TRUE, "Controller?"=TRUE, "Invert PWM"=FALSE}, {"Controller Name"=enum."10 Comm Nissan", "CommSeg"=5, "PWM?"=TRUE, "Frequency"=10, "Low Command"=50.0, "High Command"=90.0, "Stop Command"=50.0, "Command Step"=0.1, "Solenoid Stop?"=TRUE, "Controller?"=TRUE, "Invert PWM"=FALSE}]  # Controller List
        w537 = T19[] [enum."Get Profiles", enum."Enable Background", enum."Get/Release Control", enum."Get Pressure", enum."Get Alarms", enum."Controller Change", enum."Set Watlow Temp 1", enum."Set Watlow Temp 2", enum."Update Controls"] items=["Main", "Init Files", "Init", "Unused", "Save As", "Start Profile", "Check Step Time", "Alarm", "Alarm Dismiss", "Run Step", "Stop Profile", "Cycle Reset", "Time Reset", "Time Reset All", "Time Set", "Tare CTs", "Save Profile", "Open Profile", "Get Profiles", "Update Screen", "Update Controls", "Save App Config", "Write Outputs", "Disable Background", "Enable Background", "Get/Release Control", "Log Fuel Change", "Fuel Change Popup", "Read Inputs", "Remote Timer Reset", "Controller Change", "Get Alarms", "Init Alarms", "Save Alarms", "Voltage Selection", "Set Watlow Temp 1", "Set Watlow Temp 2", "Get Pressure", "Write Tare Pressure", "Adjust Controls", "Reinit ADC", "Write Initial Times", "Write Pumps Present", "HMI Command", "Save Pump Times"]
        n206 = Unbundle By Name(w542) -> ("App Config.Profiles Path"=w546:path, "App Config.Controller Type:"=w540:T2)
        n207 = Unbundle By Name(w542) -> ("App Config.Watlow Present"=w529:bool, "App Config.Temp 1"=w539:dbl, "App Config.Temp 2"=w538:dbl, "App Config.Location"=→"Location:":string)
        n208 = local write "Main Tab"(T5."Main" ("Main Tab")) -> ()
        n209 = local write "pb.Run Profile"(FALSE ("pb.Run Profile")) -> ()
        n210 = Index Array(array=w536, index=w540) -> (element=w541:T41)
        n211 = local write "Controller Type:"(w540) -> ()
        n212 = call "Watlow Global.vi"("Write (F)"=TRUE, "Watlow Present"=w529) -> ()  [unwired: 9 in, 1 out]
        n213 = Unbundle By Name(w541) -> ("High Command"=w545:dbl, "Low Command"=w544:dbl, "Command Step"=w543:dbl, "Stop Command"=w547:dbl)
        n214 = local write "Tank 1 Temp Cmd:"(w539) -> ()
        n215 = local write "Tank 2 Temp Cmd:"(w538) -> ()
        n216 = property on="Manual CMD" class="DigNum (strict)"("Maximum"=w545, "Minimum"=w544, "Increment"=w543) -> ()  [unwired: 2 in, 2 out]
        n217 = call "Init FPGA.vi"("FPGA Ref"=w530) -> ("error out"=w534:errorcluster, "FPGA Ref Out"=w535:T21)  [unwired: 9 in]
        n218 = call "Init ADCs.vi"("Error IN"=w534, "FPGA Ref"=w535) -> ("error out"=w533:errorcluster)  [unwired: 7 in, 2 out]
        n219 = flat-sequence {
          tunnel: w533 -> [_]
          tunnel: w532 -> [w552]
          frame #0 {
            n220 = Set Occurrence(w552) -> ()
          }
        }
        n221 = call <vilib>:"Check if File or Folder Exists.vi"("path"=w546) -> ("file or folder exists?"=w551:bool, "dup path"=w550:path)  [unwired: 8 in, 1 out]
        n222 = case shown="False" w551 {
          tunnel: w550 -> [w553 _]
          frame False {
            n223 = Create Folder(path (use dialog)=w553) -> ()  [unwired: 2 in, 3 out]
          }
          frame True {
          }
        }
        n224 = Bundle By Name(cluster=w542, "Controller List"=w536, "Controller Config"=w541, "Stop Cmd"=w547, "Tank CMDs.Temp 1 CMD"=w539, "Tank CMDs.Temp 2 CMD"=w538) -> (w548:T20)
      }
      frame "Unused" {
      }
      frame "Get Alarms" {
        n225 = Unbundle By Name(w563) -> ("Alarm Config"=w564:T7, "Alarm Config Path"=w561:path)
        n226 = call <vilib>:"Check if File or Folder Exists.vi"("path"=w561) -> ("file or folder exists?"=w566:bool, "dup path"=w565:path)  [unwired: 8 in, 1 out]
        n227 = case shown="False" w566 {
          tunnel: w565 -> [w571 w578]
          tunnel: w564 -> [_ w576]
          tunnel: [T7 {"Alarms:"=[{"Description:"="PS/E-Stop/Float Switch", "Enabled:"=TRUE, "Data Index:"=9, "Data Type:"="Tank", "Low Limit:"=5.0, "High Limit:"=20.0, "Trip Time:"=1000, "Profile Sync:"=FALSE}, {"Description:"="Voltage (pump or ctrl)", "Enabled:"=TRUE, "Data Index:"=0, "Data Type:"="Pump", "Low Limit:"=12.0, "High Limit:"=17.0, "Trip Time:"=3000, "Profile Sync:"=TRUE}, {"Description:"="Pump Current", "Enabled:"=TRUE, "Data Index:"=10, "Data Type:"="Pump", "Low Limit:"=0.0, "High Limit:"=22.0, "Trip Time:"=1000, "Profile Sync:"=TRUE}, {"Description:"="Pump Speed", "Enabled:"=TRUE, "Data Index:"=16, "Data Type:"="Pump", "Low Limit:"=0.0, "High Limit:"=10000.0, "Trip Time:"=1000, "Profile Sync:"=TRUE}, {"Description:"="Controller Current", "Enabled:"=TRUE, "Data Index:"=22, "Data Type:"="Pump", "Low Limit:"=0.0, "High Limit:"=20.0, "Trip Time:"=1000, "Profile Sync:"=TRUE}, {"Description:"="Pump Pressure", "Enabled:"=TRUE, "Data Index:"=30, "Data Type:"="Pump", "Low Limit:"=550.0, "High Limit:"=750.0, "Trip Time:"=1000, "Profile Sync:"=TRUE}, {"Description:"="Pump Flow", "Enabled:"=FALSE, "Data Index:"=36, "Data Type:"="Pump", "Low Limit:"=0.0, "High Limit:"=400.0, "Trip Time:"=1000, "Profile Sync:"=TRUE}, {"Description:"="Tank Temperature 1", "Enabled:"=FALSE, "Data Index:"=28, "Data Type:"="Tank", "Low Limit:"=-50.0, "High Limit:"=0.0, "Trip Time:"=10000, "Profile Sync:"=FALSE}, {"Description:"="Tank Temperature 2", "Enabled:"=FALSE, "Data Index:"=29, "Data Type:"="Tank", "Low Limit:"=0.0, "High Limit:"=70.0, "Trip Time:"=10000, "Profile Sync:"=FALSE}], "Profile Sync:"={"Trip Time:"=2000, "Consecutive Trips:"=5}} ("Alarm Config") w574] -> w557
          tunnel: [w568 w573] -> w556
          frame False {
            w568 = T19[] [enum."Init Alarms", enum."Save Alarms"] items=["Main", "Init Files", "Init", "Unused", "Save As", "Start Profile", "Check Step Time", "Alarm", "Alarm Dismiss", "Run Step", "Stop Profile", "Cycle Reset", "Time Reset", "Time Reset All", "Time Set", "Tare CTs", "Save Profile", "Open Profile", "Get Profiles", "Update Screen", "Update Controls", "Save App Config", "Write Outputs", "Disable Background", "Enable Background", "Get/Release Control", "Log Fuel Change", "Fuel Change Popup", "Read Inputs", "Remote Timer Reset", "Controller Change", "Get Alarms", "Init Alarms", "Save Alarms", "Voltage Selection", "Set Watlow Temp 1", "Set Watlow Temp 2", "Get Pressure", "Write Tare Pressure", "Adjust Controls", "Reinit ADC", "Write Initial Times", "Write Pumps Present", "HMI Command", "Save Pump Times"]
            n228 = Open/Create/Replace File(file path (use dialog)=w571, operation (0:open)=T24."create") -> (refnum out=w570:refnum<file>, error out=w569:errorcluster)  [unwired: 4 in, 1 out]
            n229 = Close File(refnum=w570, error in=w569) -> ()  [unwired: 2 out]
          }
          frame True {
            w573 = T19[] [enum."Init Alarms"] items=["Main", "Init Files", "Init", "Unused", "Save As", "Start Profile", "Check Step Time", "Alarm", "Alarm Dismiss", "Run Step", "Stop Profile", "Cycle Reset", "Time Reset", "Time Reset All", "Time Set", "Tare CTs", "Save Profile", "Open Profile", "Get Profiles", "Update Screen", "Update Controls", "Save App Config", "Write Outputs", "Disable Background", "Enable Background", "Get/Release Control", "Log Fuel Change", "Fuel Change Popup", "Read Inputs", "Remote Timer Reset", "Controller Change", "Get Alarms", "Init Alarms", "Save Alarms", "Voltage Selection", "Set Watlow Temp 1", "Set Watlow Temp 2", "Get Pressure", "Write Tare Pressure", "Adjust Controls", "Reinit ADC", "Write Initial Times", "Write Pumps Present", "HMI Command", "Save Pump Times"]
            n230 = Read from Text File(file (use dialog)=w578) -> (refnum out=w575:refnum<file>, text=w577:string)  [unwired: 3 in, 2 out]
            n231 = Close File(refnum=w575) -> ()  [unwired: 1 in, 2 out]
            n232 = Unflatten From JSON(JSON string=w577, type and defaults=w576) -> (value=w574:T7)  [unwired: 5 in, 1 out]
          }
        }
        n233 = Bundle By Name(cluster=w563, "Alarm Config"=w557) -> (w562:T20)
        n234 = local write "Alarm Config"(w557) -> ()
        n235 = Insert Into Array(array=w558, index=0, new element=w556) -> (w559:T19[])
      }
      frame "Init Alarms" {
        # "Initialize alarm arrays."
        n236 = Unbundle By Name(w585) -> ("Alarm Config.Alarms:"=w587:T8[])
        n237 = for {
          tunnel: w587 -> [w594] mode=indexing
          shift-right: [w590] -> w581
          shift-left: 0 -> [w589]
          n238 = Unbundle By Name(w594) -> ("Data Type:"=w593:string, "Enabled:"=w592:bool)
          n239 = case shown="\"Pump\", Default" w593 {
            tunnel: [6 1] -> w591
            frame "Pump", Default {
            }
            frame "Tank" {
            }
          }
          n240 = case shown="True" w592 {
            tunnel: w591 -> [_ w598]
            tunnel: [w595 w597] -> w590
            tunnel: w589 -> [w595 w596]
            frame False {
            }
            frame True {
              n241 = Add(x=w598, y=w596) -> (x+y=w597:i32)
            }
          }
        }
        n242 = Tick Count (ms)() -> (millisecond timer value=w582:u32)
        n243 = Initialize Array(0, w581) -> (w580:i32[])
        n244 = Initialize Array(w582, w581) -> (w579:u32[])
        n245 = Bundle By Name(cluster=w585, "Trip Counters"=w580, "Previous Times"=w579, "Prev ON Times"=w579) -> (w584:T20)
      }
      frame "Save Alarms" {
        n246 = Unbundle By Name(w604) -> ("Alarm Config Path"=w602:path, "Alarm Config"=w603:T7)
        n247 = Flatten To JSON(anything=w603) -> (JSON string=w601:string)  [unwired: 2 in, 1 out]
        n248 = Write to Text File(file (use dialog)=w602, text=w601) -> ()  [unwired: 2 in, 3 out]
      }
      frame "Get Profiles" {
        n249 = Unbundle By Name(w613) -> ("App Config.Profiles Path"=w614:path)
        n250 = List Folder(path=w614) -> (filenames=w611:string[], error out=w610:errorcluster)  [unwired: 3 in, 2 out]
        n251 = call <vilib>:"Clear Errors.vi"("error in (no error)"=w610) -> ()  [unwired: 6 in, 1 out]
        n252 = property on="Profile Name:" class="CmbBox"("Strings[]"=w611) -> ()  [unwired: 2 in, 2 out]
        n253 = Bundle By Name(cluster=w613, "Profiles"=w611) -> (w612:T20)
        n254 = Insert Into Array(array=w607, index=0, new element=Sequence_States."Open Profile") -> (w606:T19[])
      }
      frame "Open Profile" {
        w616 = T19[] [enum."Update Screen", enum."Save App Config"] items=["Main", "Init Files", "Init", "Unused", "Save As", "Start Profile", "Check Step Time", "Alarm", "Alarm Dismiss", "Run Step", "Stop Profile", "Cycle Reset", "Time Reset", "Time Reset All", "Time Set", "Tare CTs", "Save Profile", "Open Profile", "Get Profiles", "Update Screen", "Update Controls", "Save App Config", "Write Outputs", "Disable Background", "Enable Background", "Get/Release Control", "Log Fuel Change", "Fuel Change Popup", "Read Inputs", "Remote Timer Reset", "Controller Change", "Get Alarms", "Init Alarms", "Save Alarms", "Voltage Selection", "Set Watlow Temp 1", "Set Watlow Temp 2", "Get Pressure", "Write Tare Pressure", "Adjust Controls", "Reinit ADC", "Write Initial Times", "Write Pumps Present", "HMI Command", "Save Pump Times"]
        n255 = Unbundle By Name(w629) -> ("App Config.Profiles Path"=w631:path, "App Config.Current Profile"=w630:string)
        n256 = Build Path(base path=w631, name or relative path=w630) -> (appended path=w626:path)
        n257 = Read from Text File(file (use dialog)=w626) -> (refnum out=w624:refnum<file>, text=w625:string, error out=w623:errorcluster)  [unwired: 3 in, 1 out]
        n258 = Close File(refnum=w624, error in=w623) -> (error out=w622:errorcluster)  [unwired: 1 out]
        n259 = case shown="No Error" w622 {
          tunnel: w625 -> [w633 _]
          tunnel: [w634 string[][] []] -> w615
          frame No Error {
            n260 = Spreadsheet String To Array(delimiter (Tab)=",", format string="%s", spreadsheet string=w633, array type (2D Dbl)=string[][] []) -> (array=w634:string[][])
          }
          frame Error {
          }
        }
        n261 = Array Size(array=w615) -> (size(s)=w627:i32[])
        n262 = Index Array(array=w627) -> (element=w620:i32)  [unwired: 1 in]
        n263 = Bundle By Name(cluster=w629, "Profile"=w615, "# of Steps"=w620, "Update Profile"=TRUE) -> (w628:T20)
        n264 = Insert Into Array(array=w618, index=0, new element=w616) -> (w617:T19[])
      }
      frame "Save Profile" {
        n265 = Unbundle By Name(w644) -> ("App Config.Profiles Path"=w648:path, "App Config.Current Profile"=w646:string, "Profile"=w647:string[][])
        n266 = Empty String/Path?(string/path=w646) -> (empty?=w645:bool)
        n267 = case shown="False" w645 {
          tunnel: w648 -> [w652 _]
          tunnel: w646 -> [w651 _]
          tunnel: w647 -> [w650 _]
          tunnel: [w649 string[][] [] ("Profile OUT")] -> w641
          frame False {
            n268 = call "Save Profile.vi"("Profile"=w650, "Current Profile"=w651, "Profiles Path"=w652) -> ("Profile OUT"=w649:string[][])  [unwired: 8 in]
          }
          frame True {
          }
        }
        n269 = Array Size(array=w641) -> (size(s)=w642:i32[])
        n270 = Index Array(array=w642) -> (element=w640:i32)  [unwired: 1 in]
        n271 = Bundle By Name(cluster=w644, "Profile"=w641, "# of Steps"=w640, "Update Profile"=TRUE) -> (w643:T20)
      }
      frame "Start Profile" {
        w657 = T19[] [enum."Init Alarms", enum."Check Step Time"] items=["Main", "Init Files", "Init", "Unused", "Save As", "Start Profile", "Check Step Time", "Alarm", "Alarm Dismiss", "Run Step", "Stop Profile", "Cycle Reset", "Time Reset", "Time Reset All", "Time Set", "Tare CTs", "Save Profile", "Open Profile", "Get Profiles", "Update Screen", "Update Controls", "Save App Config", "Write Outputs", "Disable Background", "Enable Background", "Get/Release Control", "Log Fuel Change", "Fuel Change Popup", "Read Inputs", "Remote Timer Reset", "Controller Change", "Get Alarms", "Init Alarms", "Save Alarms", "Voltage Selection", "Set Watlow Temp 1", "Set Watlow Temp 2", "Get Pressure", "Write Tare Pressure", "Adjust Controls", "Reinit ADC", "Write Initial Times", "Write Pumps Present", "HMI Command", "Save Pump Times"]
        w660 = 0 ("Current Step")
        n272 = case shown="True" "Data Log Enabled" {
          tunnel: w655 -> [_ w672]
          frame False {
          }
          frame True {
            n273 = Unbundle By Name(w672) -> ("App Config"=w671:T1, "Profile"=w670:string[][], "App Config.Controller Type:"=w669:T2, "Tank CMDs"=w667:T13)
            n274 = Format Into String(w669) -> (resulting string=w668:string)  [unwired: 3 in, 1 out]
            n275 = Bundle By Name(cluster=T26 {"App Config"={"Location"="", "Profiles Path"=path "", "Current Profile"="", "CA Number"="", "Cycles Completed"=0, "Controller Type:"=enum."Kuhnke", "Stagger Time (ms)"=0, "Tank 1 Fuel"="", "Tank 2 Fuel"="", "Serial Numbers"={"Position 1 SN"="", "Position 2 SN"="", "Poaition 3 SN"="", "Position 4 SN"="", "Position 5 SN"="", "Position 6 SN"=""}, "Pumps Present"={"Pump 1"=FALSE, "Pump 2"=FALSE, "Pump 3"=FALSE, "Pump 4"=FALSE, "Pump 5"=FALSE, "Pump 6"=FALSE}, "VoltCtrlRef"="", "VoltageSelect"=FALSE, "Watlow Present"=FALSE, "Temp 1"=0.0, "Temp 2"=0.0, "V_Run PI?"=FALSE, "Voltage Limits"={"V_Step"=0.0, "V_CmdMax"=0.0, "V_CmdMin"=0.0}, "Voltage Far PI"={"V_FarSlew"=0.0, "V_FarKp"=0.0, "V_FarKi"=0.0}, "Voltage Mid PI"={"V_MidSlew"=0.0, "V_MidKp"=0.0, "V_MidKi"=0.0}, "Voltage Close PI"={"V_CloseSlew"=0.0, "V_CloseKp"=0.0, "V_CloseKi"=0.0}, "Voltage Scale"={"V_FFm"=0.0, "V_FFb"=0.0}, "Voltage Cutoffs"={"V_MidCutoff"=0.0, "V_CloseCutoff"=0.0}, "Pressure Scale"={"Pres_FFm"=0.0, "Pres_FFb"=0.0}, "Temp Format"=0, "Temp Tolerance"=0.0, "Target Voltage"=0.0, "Target Pressure"=0.0, "Data Log Init"={"Data Path"=path "", "Data Log Rate (S/s)"=0, "AKLH Rate (Hours/S)"=0.0, "Sync Time Offset (min)"=0, "IP Last 3"=0, "WebDAV IP"=""}, "Email Handler IP"="", "ADC Check"=FALSE}, "Profile"=[], "Controller Type"="", "Tank CMDs"={"PS CMD"=0.0, "Press CMD"=0.0, "Temp 1 CMD"=0.0, "Temp 2 CMD"=0.0}} ("Data Log Start"), "App Config"=w671, "Profile"=w670, "Controller Type"=w668, "Tank CMDs"=w667) -> (w673:T26)
            n276 = call "Data Logger Main.vi"("Data Logger Mode"=Data_Logger_Mode."Start", "Data Log Start"=w673) -> ()  [unwired: 18 in]
          }
        }
        n277 = property on="Main Tab" class="TabCtl (strict)"("DisabledEnum"=T25."Disabled" ("Disabled")) -> ()  [unwired: 2 in, 2 out]
        n278 = Get Date/Time In Seconds() -> (seconds since 1Jan1904=w664:timestamp)
        n279 = To Double Precision Float(number=w664) -> (double precision float=w663:dbl)
        n280 = Bundle By Name(cluster=w655, "Recording"="Data Log Enabled", "Run Profile"=TRUE, "Step Start Time"=w663, "Last Profile Time"=w663, "Step Time"=0.0, "Current Step"=w660, "Stagger Counter"=w660) -> (w666:T20)
        n281 = Insert Into Array(array=w659, index=0, new element=w657) -> (w658:T19[])
      }
      frame "Check Step Time" {
        # "Time elapsed since\nstart of step."
        n282 = Unbundle By Name(w699) -> ("Step Start Time"=w702:dbl, "Step Time"=w700:dbl, "Current Step"=w696:i32, "App Config.Stagger Time (ms)"=w680:i32, "Stagger Counter"=w686:i32)
        n283 = Get Date/Time In Seconds() -> (seconds since 1Jan1904=w701:timestamp)
        n284 = Increment(x=w686) -> (x+1=w681:i32)
        n285 = To Double Precision Float(number=w701) -> (double precision float=w694:dbl)
        n286 = Multiply(x=w680, y=w681) -> (x*y=w692:i32)
        n287 = Subtract(x=w694, y=w702) -> (x-y=w691:dbl)
        n288 = To Double Precision Float(number=w692) -> (double precision float=w685:dbl)
        n289 = Divide(x=w685, y=1000.0) -> (x/y=w683:dbl)
        n290 = Not Equal To 0?(x=w680) -> (x != 0?=w679:bool)
        n291 = Greater Or Equal?(x=w691, y=w683) -> (x >= y?=w690:bool)
        n292 = Less Or Equal?(x=w686, y=4) -> (x <= y?=w688:bool)
        n293 = Subtract(x=w700, y=w691) -> (x-y=w697:dbl)
        n294 = Compound Arithmetic op=AND(w690, w688, w679) -> (w687:bool)
        n295 = Less Or Equal To 0?(x=w697) -> (x <= 0?=w682:bool)
        n296 = case shown="False" w682 {
          tunnel: [w707 w715] -> w676
          tunnel: w696 -> [w708 w717]
          tunnel: [w708 w716] -> w695
          tunnel: [w704 0 ("Stagger Counter")] -> w693
          tunnel: w687 -> [w706 _]
          tunnel: w686 -> [w705 _]
          tunnel: w677 -> [w703 _]
          frame False {
            # "There's time left.  Update screen."
            n297 = case shown="True" w706 {
              tunnel: [w709 w713] -> w707
              tunnel: w705 -> [w710 w712]
              tunnel: [w710 w711] -> w704
              tunnel: w703 -> [w709 _]
              frame False {
              }
              frame True {
                w713 = T19[] [enum."Run Step"] items=["Main", "Init Files", "Init", "Unused", "Save As", "Start Profile", "Check Step Time", "Alarm", "Alarm Dismiss", "Run Step", "Stop Profile", "Cycle Reset", "Time Reset", "Time Reset All", "Time Set", "Tare CTs", "Save Profile", "Open Profile", "Get Profiles", "Update Screen", "Update Controls", "Save App Config", "Write Outputs", "Disable Background", "Enable Background", "Get/Release Control", "Log Fuel Change", "Fuel Change Popup", "Read Inputs", "Remote Timer Reset", "Controller Change", "Get Alarms", "Init Alarms", "Save Alarms", "Voltage Selection", "Set Watlow Temp 1", "Set Watlow Temp 2", "Get Pressure", "Write Tare Pressure", "Adjust Controls", "Reinit ADC", "Write Initial Times", "Write Pumps Present", "HMI Command", "Save Pump Times"]
                n298 = Increment(x=w712) -> (x+1=w711:i32)
              }
            }
          }
          frame True {
            w715 = T19[] [enum."Run Step"] items=["Main", "Init Files", "Init", "Unused", "Save As", "Start Profile", "Check Step Time", "Alarm", "Alarm Dismiss", "Run Step", "Stop Profile", "Cycle Reset", "Time Reset", "Time Reset All", "Time Set", "Tare CTs", "Save Profile", "Open Profile", "Get Profiles", "Update Screen", "Update Controls", "Save App Config", "Write Outputs", "Disable Background", "Enable Background", "Get/Release Control", "Log Fuel Change", "Fuel Change Popup", "Read Inputs", "Remote Timer Reset", "Controller Change", "Get Alarms", "Init Alarms", "Save Alarms", "Voltage Selection", "Set Watlow Temp 1", "Set Watlow Temp 2", "Get Pressure", "Write Tare Pressure", "Adjust Controls", "Reinit ADC", "Write Initial Times", "Write Pumps Present", "HMI Command", "Save Pump Times"]
            # "No time left.  Go to next step."
            n299 = Increment(x=w717) -> (x+1=w716:i32)
          }
        }
        n300 = Bundle By Name(cluster=w699, "Last Profile Time"=w694, "Step Time Left"=w697, "New Step"=w682, "Current Step"=w695, "Stagger Counter"=w693) -> (w698:T20)
        n301 = Insert Into Array(array=w677, index=0, new element=w676) -> ()  [unwired: 1 out]
      }
      frame "Run Step" {
        w719 = T19[] [enum."Write Outputs", enum."Read Inputs", enum."Update Screen"] items=["Main", "Init Files", "Init", "Unused", "Save As", "Start Profile", "Check Step Time", "Alarm", "Alarm Dismiss", "Run Step", "Stop Profile", "Cycle Reset", "Time Reset", "Time Reset All", "Time Set", "Tare CTs", "Save Profile", "Open Profile", "Get Profiles", "Update Screen", "Update Controls", "Save App Config", "Write Outputs", "Disable Background", "Enable Background", "Get/Release Control", "Log Fuel Change", "Fuel Change Popup", "Read Inputs", "Remote Timer Reset", "Controller Change", "Get Alarms", "Init Alarms", "Save Alarms", "Voltage Selection", "Set Watlow Temp 1", "Set Watlow Temp 2", "Get Pressure", "Write Tare Pressure", "Adjust Controls", "Reinit ADC", "Write Initial Times", "Write Pumps Present", "HMI Command", "Save Pump Times"]
        n302 = Unbundle By Name(w738) -> ("Profile"=w731:string[][], "Current Step"=w730:i32, "# of Steps"=w729:i32, "App Config.Cycles Completed"=w728:u32, "App Config.Pumps Present"=w720:T4, "New Step"=w736:bool, "Step Start Time"=w735:dbl)
        n303 = call "Run Step.vi"("Profile"=w731, "Current Step in"=w730, "# of Steps"=w729, "Cycles Completed in"=w728, "Pumps Present"=w720) -> ("PS Cmd"=w727:dbl, "Press Cmd"=w726:dbl, "Ignition Relays"=w725:T4, "Current Step out"=w724:i32, "Cycles Completed out"=w723:u32, "Step Time"=w722:dbl, "Controller CMDs"=w721:dbl[])  [unwired: 16 in]
        n304 = case shown="True" w736 {
          tunnel: [w742 w743] -> w718
          tunnel: w735 -> [w742 _]
          tunnel: w721 -> [_ _]
          frame False {
          }
          frame True {
            n305 = Get Date/Time In Seconds() -> (seconds since 1Jan1904=w744:timestamp)
            n306 = To Double Precision Float(number=w744) -> (double precision float=w743:dbl)
          }
        }
        n307 = flat-sequence {
          tunnel: w718 -> [_]
          frame #0 {
            n308 = Tick Count (ms)() -> (millisecond timer value=w741:u32)
            n309 = feedback #1() -> (w740:u32)  [unwired: 1 in]
            n310 = feedback-in #1(w741) -> ()
            n311 = Subtract(x=w741, y=w740) -> (x-y=→"Run Step (ms)":u32)
          }
        }
        n312 = Bundle By Name(cluster=w738, "Tank CMDs.PS CMD"=w727, "Tank CMDs.Press CMD"=w726, "Ignition Relay"=w725, "Current Step"=w724, "App Config.Cycles Completed"=w723, "Step Time"=w722, "Controller CMDs"=w721, "Step Start Time"=w718) -> (w737:T20)
        n313 = Insert Into Array(array=w733, index=0, new element=w719) -> (w732:T19[])
      }
      frame "Write Outputs" {
        w745 = T19[] [] items=["Main", "Init Files", "Init", "Unused", "Save As", "Start Profile", "Check Step Time", "Alarm", "Alarm Dismiss", "Run Step", "Stop Profile", "Cycle Reset", "Time Reset", "Time Reset All", "Time Set", "Tare CTs", "Save Profile", "Open Profile", "Get Profiles", "Update Screen", "Update Controls", "Save App Config", "Write Outputs", "Disable Background", "Enable Background", "Get/Release Control", "Log Fuel Change", "Fuel Change Popup", "Read Inputs", "Remote Timer Reset", "Controller Change", "Get Alarms", "Init Alarms", "Save Alarms", "Voltage Selection", "Set Watlow Temp 1", "Set Watlow Temp 2", "Get Pressure", "Write Tare Pressure", "Adjust Controls", "Reinit ADC", "Write Initial Times", "Write Pumps Present", "HMI Command", "Save Pump Times"]
        n314 = Unbundle By Name(w763) -> ("App Config.Pumps Present"=w769:T4, "Controller Config.Controller Name"=w770:T2, "Controller Config.Frequency"=w768:i32, "Controller CMDs"=w767:dbl[], "Stagger Counter"=w766:i32, "App Config.Stagger Time (ms)"=w765:i32, "Run Profile"=w764:bool, "Power Relay"=w751:T4, "Ignition Relay"=w750:T4, "Tank CMDs"=w753:T13, "App Config"=w752:T1, "Voltage Enable"=w749:bool, "App Config.V_Run PI?"=w760:bool, "Tank CMDs.PS CMD"=w755:dbl, "Tank Data.PS Actual (V):"=w759:dbl, "App Config.VoltCtrlRef"=w754:string)
        n315 = call "Write FPGA Outputs.vi"("FPGA Ref"=w757, "Tank CMDs"=w753, "App Config"=w752, "Power Relay"=w751, "Ignition Relay"=w750, "Voltage Enable"=w749) -> ("FPGA Ref OUT"=w756:T21)  [unwired: 13 in]
        n316 = call "Power Supply Global.vi"("Closed Loop"=w760, "PS Global Mode"=Power_Supply_Global_Mode."Write Setpoint", "PS Cmd"=w755, "PS Voltage"=w759, "VoltCtrlRef"=w754) -> ()  [unwired: 6 in, 5 out]
        n317 = case shown="\"Conti\"..\"Hella BLDC Turbine OL PWM\"" w770 {
          selector: w770 -> [_ w782]
          tunnel: w756 -> [w777 _]
          tunnel: w769 -> [_ w786]
          tunnel: w768 -> [w776 _]
          tunnel: w767 -> [w775 w784]
          tunnel: w766 -> [w774 _]
          tunnel: w765 -> [w773 _]
          tunnel: w764 -> [w772 _]
          tunnel: [w771 w784] -> w761
          tunnel: w751 -> [_ w781]
          tunnel: w750 -> [_ w780]
          frame "Kuhnke", "Helbako BLDC", "PSA", Default {
            n318 = call "Write PWM Outputs.vi"("FPGE Ref"=w777, "Frequency"=w776, "Controller CMDs IN"=w775, "Stagger Counter"=w774, "Stagger Time (ms)"=w773, "Run Profile"=w772) -> ("Controller CMDs OUT"=w771:dbl[])  [unwired: 13 in]
          }
          frame "Conti".."Hella BLDC Turbine OL PWM" {
            n319 = Cluster To Array(cluster=w786) -> (array=w779:bool[])
            n320 = Search 1D Array(1D array=w779, element=TRUE) -> (index of element=w785:i32)  [unwired: 1 in]
            n321 = Less Than 0?(x=w785) -> (x < 0?=w790:bool)
            n322 = Select(t=0, s=w790, f=w785) -> (s? t:f=w788:i32)
            n323 = Index Array(array=w784, index=w788) -> (element=w778:dbl)
            n324 = call "CAN Global.vi"("Controller Type:"=w782, "Write (F)"=TRUE, "CAN Cmd"=w778, "Power Relay"=w781, "Ignition Relay"=w780) -> ()  [unwired: 7 in, 4 out]
          }
        }
        n325 = Bundle By Name(cluster=w763, "Controller CMDs"=w761) -> (w762:T20)
        n326 = Insert Into Array(array=w747, index=0, new element=w745) -> (w746:T19[])
      }
      frame "Read Inputs" {
        w791 = FALSE ("WebDAV Push")
        n327 = Unbundle By Name(w838) -> ("Concat Data"=w792:bool, "WebDAV Push"=w802:bool, "Current Step"=w801:i32, "Step Time Left"=w800:dbl, "Run Profile"=w821:bool, "Controller Config"=w815:T16, "Trip Counters"=w831:i32[], "Previous Times"=w830:u32[], "Prev ON Times"=w829:u32[], "Alarm Config"=w832:T7, "Alarm Message 2"=w825:string, "Alarm Message 1"=w826:string, "Alarm Latch"=w827:bool, "App Config.Pumps Present"=w813:T4, "Power Relay"=w833:T4, "Controller CMDs"=w816:dbl[], "App Config"=w817:T1, "Tank CMDs"=w818:T13, "Time/Date"=w822:string, "Run Profile"=w814:bool, "Recording"=w824:bool, "Power Relay"=w820:T4, "App Config.ADC Check"=w794:bool)
        n328 = Cluster To Array(cluster=w813) -> (array=w798:bool[])
        n329 = call "Tank Data Global.vi"() -> ("Tank Data OUT"=w837:dbl[], "Pump Data"=w804:T11, "Tank Data"=w803:T17, "Record Time (sec)"=w793:dbl)  [unwired: 12 in]
        n330 = call "Evaluate Alarms.vi"("In Test"=w821, "Controller"=w815, "Alarm Config"=w832, "Data"=w837, "Pumps Present"=w798, "Trip Counter"=w831, "Previous Times"=w830, "Manual CMDs"=w816, "Prev ON Times"=w829) -> ("Trip Counter OUT"=w836:i32[], "Previous Times OUT"=w835:u32[], "Alarm Tripped"=w806:bool, "Prev ON Times OUT"=w834:u32[], "Alarm Message 1"=w811:string, "Alarm Message 2"=w810:string)  [unwired: 13 in]
        n331 = call "RPi HMI Com.vi"("Pump Data"=w804, "Tank Data"=w803, "Power Relays"=w833, "Pump CMDs"=w816, "App Config"=w817, "Tank CMDs"=w818, "Alarm"=w827, "RPi HMI Mode"=RPi_HMI_Mode."Write Data", "In Test"=w814, "Alarm Message 1"=w826, "Controller Config"=w815, "Alarm Message 2"=w825, "Recording"=w824, "Pumps Present"=w798, "Time/Date"=w822) -> ()  [unwired: 4 in, 1 out]
        n332 = call "Freeze PID.vi"("Run Profile"=w814, "Controller CMDs"=w816, "Controller Config"=w815, "Power Relay"=w820) -> ()  [unwired: 12 in]
        n333 = call "Enable Timers.vi"("FPGA Ref"=w819, "Tank Data"=w803, "Tank CMDs"=w818, "App Config"=w817, "Controller CMDs"=w816, "Controller Config"=w815, "Run Profile"=w814, "Pumps Present"=w798) -> ("In Spec"=w799:bool[], "Reset ADCs"=w796:bool)  [unwired: 18 in]
        n334 = call "Data Logger Global.vi"("WebDAV Push"=w802, "In Spec"=w799, "Current Step"=w801, "Step Time Left"=w800, "Pump Data"=w804, "Tank Data"=w803, "Concat Data"=w792, "Record Time (sec)"=w793, "Write (F)"=TRUE) -> ()  [unwired: 3 in, 8 out]
        n335 = flat-sequence {
          frame #0 {
            n336 = Tick Count (ms)() -> (millisecond timer value=w841:u32)
            n337 = feedback #2() -> (w840:u32)  [unwired: 1 in]
            n338 = feedback-in #2(w841) -> ()
            n339 = Subtract(x=w841, y=w840) -> (x-y=→"Read Inputs (ms)":u32)
          }
        }
        n340 = And(x=w796, y=w794) -> (x .and. y?=w795:bool)
        n341 = case shown="True" w795 {
          tunnel: w823 -> [w847 w851]
          tunnel: [w847 w850] -> w808
          frame False {
          }
          frame True {
            n342 = Insert Into Array(array=w851, index=0, new element=Sequence_States."Reinit ADC" ("new element/subarray")) -> (w850:T19[])
          }
        }
        n343 = Tick Count (ms)() -> (millisecond timer value=w797:u32)
        n344 = call "Get Time and Date.vi"() -> ("Time/Date"=w809:string)  [unwired: 11 in]
        n345 = case shown="True" w806 {
          tunnel: w808 -> [w842 w846]
          tunnel: [w842 w845] -> w807
          frame False {
          }
          frame True {
            w843 = T19[] [enum."Stop Profile", enum."Update Screen", enum."Disable Background", enum."Alarm"] items=["Main", "Init Files", "Init", "Unused", "Save As", "Start Profile", "Check Step Time", "Alarm", "Alarm Dismiss", "Run Step", "Stop Profile", "Cycle Reset", "Time Reset", "Time Reset All", "Time Set", "Tare CTs", "Save Profile", "Open Profile", "Get Profiles", "Update Screen", "Update Controls", "Save App Config", "Write Outputs", "Disable Background", "Enable Background", "Get/Release Control", "Log Fuel Change", "Fuel Change Popup", "Read Inputs", "Remote Timer Reset", "Controller Change", "Get Alarms", "Init Alarms", "Save Alarms", "Voltage Selection", "Set Watlow Temp 1", "Set Watlow Temp 2", "Get Pressure", "Write Tare Pressure", "Adjust Controls", "Reinit ADC", "Write Initial Times", "Write Pumps Present", "HMI Command", "Save Pump Times"]
            n346 = Insert Into Array(array=w846, index=0, new element=w843) -> (w845:T19[])
          }
        }
        n347 = Bundle By Name(cluster=w838, "Inputs Timer"=w797, "Pump Data"=w804, "Tank Data"=w803, "Trip Counters"=w836, "Previous Times"=w835, "Alarm Latch"=w806, "Prev ON Times"=w834, "Alarm Message 1"=w811, "Alarm Message 2"=w810, "Time/Date"=w809, "WebDAV Push"=w791, "Concat Data"=w791) -> (w812:T20)
      }
      frame "Update Screen" {
        n348 = Unbundle By Name(w854) -> ("App Config.Cycles Completed"=→"Cycles Completed:":u32, "Current Step"=→"Current Step:":i32, "Step Time Left"=→"Step Time Left:":dbl, "Time/Date"=→"Time/Date":string, "Recording"=→"Recording":bool, "Pump Data"=w856:T11, "Tank Data"=w855:T17, "Run Profile"=w861:bool)
        n349 = Unbundle(w856) -> ("Voltages"=→"Voltages":dbl[], "PumpCurrent"=→"PumpCurrent":dbl[], "Speed"=→"Speed":dbl[], "ControllerCurrent"=→"ControllerCurrent":dbl[], "Pressure"=→"Pressure":dbl[], "Flow"=→"Flow":dbl[], "Elapsed Time:"=→"Elapsed Time:":dbl[], "Avg Pressure"=→"Avg Press:":dbl, "Avg Speed"=→"Ave. Speed":dbl)
        n350 = Unbundle(w855) -> ("PS Actual (V):"=→"PS Actual (V):":dbl, "Temp1"=→"Temp1":dbl, "Temp2"=→"Temp2":dbl)
        n351 = flat-sequence {
          frame #0 {
            n352 = Tick Count (ms)() -> (millisecond timer value=w881:u32)
            n353 = feedback #3() -> (w880:u32)  [unwired: 1 in]
            n354 = feedback-in #3(w881) -> ()
            n355 = Subtract(x=w881, y=w880) -> (x-y=→"Update Screen (ms)":u32)
          }
        }
        n356 = case shown="True" w861 {
          tunnel: [w882 w885] -> w878
          tunnel: w877 -> [w882 w884]
          frame False {
          }
          frame True {
            w883 = T19[] [enum."Save Pump Times", enum."Update Controls"] items=["Main", "Init Files", "Init", "Unused", "Save As", "Start Profile", "Check Step Time", "Alarm", "Alarm Dismiss", "Run Step", "Stop Profile", "Cycle Reset", "Time Reset", "Time Reset All", "Time Set", "Tare CTs", "Save Profile", "Open Profile", "Get Profiles", "Update Screen", "Update Controls", "Save App Config", "Write Outputs", "Disable Background", "Enable Background", "Get/Release Control", "Log Fuel Change", "Fuel Change Popup", "Read Inputs", "Remote Timer Reset", "Controller Change", "Get Alarms", "Init Alarms", "Save Alarms", "Voltage Selection", "Set Watlow Temp 1", "Set Watlow Temp 2", "Get Pressure", "Write Tare Pressure", "Adjust Controls", "Reinit ADC", "Write Initial Times", "Write Pumps Present", "HMI Command", "Save Pump Times"]
            n357 = Insert Into Array(array=w884, index=0, new element=w883) -> (w885:T19[])
          }
        }
        n358 = call "App Global.vi"() -> ("CPU Usage OUT"=→"CPU Usage:":dbl, "Login OUT"=w857:bool)  [unwired: 9 in, 1 out]
        n359 = Tick Count (ms)() -> (millisecond timer value=w852:u32)
        n360 = local write "Login"(w857) -> ()
        n361 = Bundle By Name(cluster=w854, "Screen Timer"=w852) -> (w853:T20)
      }
      frame "Update Controls" {
        w897 = bool[] [FALSE, FALSE, FALSE, FALSE, FALSE, FALSE] ("pb.Resets")
        w898 = T19[] [] items=["Main", "Init Files", "Init", "Unused", "Save As", "Start Profile", "Check Step Time", "Alarm", "Alarm Dismiss", "Run Step", "Stop Profile", "Cycle Reset", "Time Reset", "Time Reset All", "Time Set", "Tare CTs", "Save Profile", "Open Profile", "Get Profiles", "Update Screen", "Update Controls", "Save App Config", "Write Outputs", "Disable Background", "Enable Background", "Get/Release Control", "Log Fuel Change", "Fuel Change Popup", "Read Inputs", "Remote Timer Reset", "Controller Change", "Get Alarms", "Init Alarms", "Save Alarms", "Voltage Selection", "Set Watlow Temp 1", "Set Watlow Temp 2", "Get Pressure", "Write Tare Pressure", "Adjust Controls", "Reinit ADC", "Write Initial Times", "Write Pumps Present", "HMI Command", "Save Pump Times"]
        n362 = Unbundle By Name(w900) -> ("App Config.Stagger Time (ms)"=w909:i32, "Profile"=w910:string[][], "App Config.Current Profile"=w905:string, "App Config.CA Number"=w904:string, "App Config.Controller Type:"=w911:T2, "App Config.Pumps Present"=w901:T4, "App Config.Tank 1 Fuel"=w908:string, "App Config.Tank 2 Fuel"=w907:string, "App Config.Serial Numbers"=w906:T34, "App Config.Target Voltage"=w903:dbl, "App Config.Target Pressure"=w902:dbl, "Email Alarms Disabled"=w896:bool, "Run Profile"=w895:bool, "Recording"=w894:bool, "Tank CMDs.Press CMD"=w893:dbl, "Controller CMDs"=w892:dbl[], "Tank CMDs.PS CMD"=w891:dbl, "Power Relay"=w890:T4, "Ignition Relay"=w889:T4, "WebDAV Push"=w888:bool, "Concat Data"=w887:bool)
        n363 = local write "pb.Resets"(w897) -> ()
        n364 = local write "pb.Sets"(w897) -> ()
        n365 = case shown="False" w895 {
          tunnel: w911 -> [w925 _]
          tunnel: w910 -> [w924 _]
          tunnel: w909 -> [w923 _]
          tunnel: w908 -> [w922 _]
          tunnel: w907 -> [w921 _]
          tunnel: w906 -> [w920 _]
          tunnel: w905 -> [w919 _]
          tunnel: w904 -> [w918 _]
          tunnel: w903 -> [w917 _]
          tunnel: w902 -> [w916 _]
          tunnel: w901 -> [w915 _]
          tunnel: w896 -> [w914 _]
          frame False {
            n366 = local write "Stagger Time (ms):"(w923) -> ()
            n367 = local write "Profile:"(w924) -> ()
            n368 = local write "Profile Name:"(w919) -> ()
            n369 = local write "CA Number:"(w918) -> ()
            n370 = local write "Controller Type:"(w925) -> ()
            n371 = local write "Pumps Present"(w915) -> ()
            n372 = local write "Tank 1 Fuel Type:"(w922) -> ()
            n373 = local write "Tank 2 Fuel Type:"(w921) -> ()
            n374 = local write "Serial Numbers"(w920) -> ()
            n375 = local write "Target Voltage:"(w917) -> ()
            n376 = local write "Target Pressure:"(w916) -> ()
            n377 = local write "Disable Alarm Email"(w914) -> ()
            "Email Alarms Disabled" <- w914
          }
          frame True {
          }
        }
        n378 = local write "pb.Run Profile"(w895) -> ()
        n379 = local write "Recording"(w894) -> ()
        n380 = local write "PressureCMD"(w893) -> ()
        n381 = local write "Controller\nCMD"(w892) -> ()
        n382 = local write "Power Supply Cmd:"(w891) -> ()
        n383 = local write "Power Relay"(w890) -> ()
        n384 = local write "Ignition Relay"(w889) -> ()
        n385 = local write "WebDAV Push"(w888) -> ()
        n386 = local write "Concat Data"(w887) -> ()
        n387 = Insert Into Array(array=w912, index=0, new element=w898) -> (w913:T19[])
      }
      frame "Stop Profile" {
        w929 = T19[] [enum."Write Outputs", enum."Update Controls"] items=["Main", "Init Files", "Init", "Unused", "Save As", "Start Profile", "Check Step Time", "Alarm", "Alarm Dismiss", "Run Step", "Stop Profile", "Cycle Reset", "Time Reset", "Time Reset All", "Time Set", "Tare CTs", "Save Profile", "Open Profile", "Get Profiles", "Update Screen", "Update Controls", "Save App Config", "Write Outputs", "Disable Background", "Enable Background", "Get/Release Control", "Log Fuel Change", "Fuel Change Popup", "Read Inputs", "Remote Timer Reset", "Controller Change", "Get Alarms", "Init Alarms", "Save Alarms", "Voltage Selection", "Set Watlow Temp 1", "Set Watlow Temp 2", "Get Pressure", "Write Tare Pressure", "Adjust Controls", "Reinit ADC", "Write Initial Times", "Write Pumps Present", "HMI Command", "Save Pump Times"]
        w935 = T4 {"Pump 1"=FALSE, "Pump 2"=FALSE, "Pump 3"=FALSE, "Pump 4"=FALSE, "Pump 5"=FALSE, "Pump 6"=FALSE} ("Power Relay")
        n388 = Unbundle By Name(w934) -> ("Controller Config.Stop Command"=w933:dbl)
        n389 = Initialize Array(w933, 6 ("dimension size")) -> (w931:dbl[])
        n390 = call "Data Logger Main.vi"("Data Logger Mode"=Data_Logger_Mode."Stop") -> ()  [unwired: 19 in]
        n391 = property on="Main Tab" class="TabCtl (strict)"("DisabledEnum"=T25."Enabled" ("Disabled")) -> ()  [unwired: 2 in, 2 out]
        n392 = Bundle By Name(cluster=w934, "Run Profile"=FALSE, "Controller CMDs"=w931, "Power Relay"=w935, "Ignition Relay"=w935, "Tank CMDs.Press CMD"=0.0, "Recording"=FALSE) -> (w927:T20)
        n393 = Insert Into Array(array=w938, index=0, new element=w929) -> (w937:T19[])
      }
      frame "Save As" {
        n394 = property on="Save As Tab" class="TabCtl (strict)"("Visible"=TRUE) -> (error out=w945:errorcluster)  [unwired: 2 in, 1 out]
        n395 = while {
          tunnel: ["pb.Save As OK"] -> w951
          tunnel: w945 -> [_]
          stop <- w953 stop-if-true
          n396 = Wait (ms)(milliseconds to wait=u32 10) -> ()  [unwired: 1 out]
          n397 = Or(x="pb.Save As OK", y="pb.Save As Cancel") -> (x .or. y?=w953:bool)
        }
        n398 = Unbundle By Name(w949) -> ("App Config.Profiles Path"=w950:path, "Profile"=w947:string[][])
        n399 = case shown="True" w951 {
          tunnel: w950 -> [_ w961]
          tunnel: [w956 w958] -> w942
          tunnel: w949 -> [w957 w963]
          tunnel: [w957 w962] -> w948
          tunnel: w947 -> [_ w960]
          frame False {
            w956 = T19[] [enum."Enable Background"] items=["Main", "Init Files", "Init", "Unused", "Save As", "Start Profile", "Check Step Time", "Alarm", "Alarm Dismiss", "Run Step", "Stop Profile", "Cycle Reset", "Time Reset", "Time Reset All", "Time Set", "Tare CTs", "Save Profile", "Open Profile", "Get Profiles", "Update Screen", "Update Controls", "Save App Config", "Write Outputs", "Disable Background", "Enable Background", "Get/Release Control", "Log Fuel Change", "Fuel Change Popup", "Read Inputs", "Remote Timer Reset", "Controller Change", "Get Alarms", "Init Alarms", "Save Alarms", "Voltage Selection", "Set Watlow Temp 1", "Set Watlow Temp 2", "Get Pressure", "Write Tare Pressure", "Adjust Controls", "Reinit ADC", "Write Initial Times", "Write Pumps Present", "HMI Command", "Save Pump Times"]
          }
          frame True {
            w958 = T19[] [enum."Enable Background", enum."Get Profiles"] items=["Main", "Init Files", "Init", "Unused", "Save As", "Start Profile", "Check Step Time", "Alarm", "Alarm Dismiss", "Run Step", "Stop Profile", "Cycle Reset", "Time Reset", "Time Reset All", "Time Set", "Tare CTs", "Save Profile", "Open Profile", "Get Profiles", "Update Screen", "Update Controls", "Save App Config", "Write Outputs", "Disable Background", "Enable Background", "Get/Release Control", "Log Fuel Change", "Fuel Change Popup", "Read Inputs", "Remote Timer Reset", "Controller Change", "Get Alarms", "Init Alarms", "Save Alarms", "Voltage Selection", "Set Watlow Temp 1", "Set Watlow Temp 2", "Get Pressure", "Write Tare Pressure", "Adjust Controls", "Reinit ADC", "Write Initial Times", "Write Pumps Present", "HMI Command", "Save Pump Times"]
            n400 = call "Save Profile.vi"("Profile"=w960, "Current Profile"="New Profile Name:", "Profiles Path"=w961) -> ()  [unwired: 8 in, 1 out]
            n401 = Bundle By Name(cluster=w963, "App Config.Current Profile"="New Profile Name:") -> (w962:T20)
          }
        }
        n402 = Insert Into Array(array=w944, index=0, new element=w942) -> (w943:T19[])
      }
      frame "Save App Config" {
        n403 = Unbundle By Name(w972) -> ("App Config"=w971:T1)
        n404 = call <vilib>:"Open Config Data.vi"("create file if necessary (T)"=TRUE, "configuration file path"=path "c:/App Config.ini") -> ("error out"=w965:errorcluster, "refnum"=w969:T39)  [unwired: 7 in, 1 out]
        n405 = call "Read Write App Config.vi"("Write (F)"=TRUE, "Error IN"=w965, "App Config"=w971, "Refnum in"=w969) -> ("Error OUT"=w967:errorcluster, "Refnum out"=w968:T39)  [unwired: 5 in, 1 out]
        n406 = call <vilib>:"Close Config Data.vi"("error in (no error)"=w967, "refnum"=w968) -> ()  [unwired: 8 in, 2 out]
      }
      frame "Save Pump Times" {
        n407 = Unbundle By Name(w978) -> ("Pump Data.Elapsed Time:"=w977:dbl[])
        n408 = Array Size(array=w977) -> (size(s)=w976:i32)
        n409 = Equal?(x=w976, y=6) -> (x = y?=w974:bool)
        n410 = case shown="True" w974 {
          tunnel: w977 -> [_ w981]
          frame False {
          }
          frame True {
            n411 = Write to Binary File(file (use dialog)=path "c:/ElapsedTimes", data=w981) -> (refnum out=w982:refnum<file>, error out=w983:errorcluster)  [unwired: 4 in, 1 out]
            n412 = Close File(refnum=w982, error in=w983) -> ()  [unwired: 2 out]
          }
        }
      }
      frame "Disable Background" {
        w984 = T25."Disabled and Grayed Out" ("Disabled")
        n413 = property on="Main Tab" class="TabCtl (strict)"("DisabledEnum"=w984) -> ()  [unwired: 2 in, 2 out]
        n414 = property on="pb.Stop Profile" class="Bool"("DisabledEnum"=w984) -> ()  [unwired: 2 in, 2 out]
        n415 = property on="Monitoring Tab" class="TabCtl (strict)"("DisabledEnum"=w984) -> ()  [unwired: 2 in, 2 out]
        n416 = property on="Title Tab" class="TabCtl (strict)"("DisabledEnum"=w984) -> ()  [unwired: 2 in, 2 out]
        n417 = property on="CPU Usage:" class="DigNum (strict)"("DisabledEnum"=w984) -> ()  [unwired: 2 in, 2 out]
        n418 = property on="Pump Timers Tab" class="TabCtl (strict)"("DisabledEnum"=w984) -> ()  [unwired: 2 in, 2 out]
        n419 = property on="Live Data Tab" class="TabCtl (strict)"("DisabledEnum"=w984) -> ()  [unwired: 2 in, 2 out]
      }
      frame "Enable Background" {
        w989 = FALSE ("Visible")
        w987 = T25."Enabled" ("Disabled")
        n420 = xnode "Read/Write Control"("FPGA VI Reference In"=w991, "Timer Resets"=bool[] [FALSE, FALSE, FALSE, FALSE, FALSE, FALSE] ("array")) -> ()  [unwired: 1 in, 2 out]
        n421 = property on="Save As Tab" class="TabCtl (strict)"("Visible"=w989) -> ()  [unwired: 2 in, 2 out]
        n422 = property on="Reset Tab" class="TabCtl (strict)"("Visible"=w989) -> ()  [unwired: 2 in, 2 out]
        n423 = property on="Set Time Tab" class="TabCtl (strict)"("Visible"=w989) -> ()  [unwired: 2 in, 2 out]
        n424 = property on="Alarm Tab" class="TabCtl (strict)"("Visible"=w989) -> ()  [unwired: 2 in, 2 out]
        n425 = property on="Fuel Change Tab" class="TabCtl (strict)"("Visible"=w989) -> ()  [unwired: 2 in, 2 out]
        n426 = property on="Main Tab" class="TabCtl (strict)"("DisabledEnum"=w987) -> ()  [unwired: 2 in, 2 out]
        n427 = property on="pb.Stop Profile" class="Bool"("DisabledEnum"=w987) -> ()  [unwired: 2 in, 2 out]
        n428 = property on="Monitoring Tab" class="TabCtl (strict)"("DisabledEnum"=w987) -> ()  [unwired: 2 in, 2 out]
        n429 = property on="Title Tab" class="TabCtl (strict)"("DisabledEnum"=w987) -> ()  [unwired: 2 in, 2 out]
        n430 = property on="CPU Usage:" class="DigNum (strict)"("DisabledEnum"=w987) -> ()  [unwired: 2 in, 2 out]
        n431 = property on="Alarm Tab" class="TabCtl (strict)"("DisabledEnum"=w987) -> ()  [unwired: 2 in, 2 out]
        n432 = property on="Pump Timers Tab" class="TabCtl (strict)"("DisabledEnum"=w987) -> ()  [unwired: 2 in, 2 out]
        n433 = property on="Live Data Tab" class="TabCtl (strict)"("DisabledEnum"=w987) -> ()  [unwired: 2 in, 2 out]
      }
      frame "Cycle Reset".."Time Reset All" {
        w994 = T19[] [enum."Enable Background", enum."Write Initial Times"] items=["Main", "Init Files", "Init", "Unused", "Save As", "Start Profile", "Check Step Time", "Alarm", "Alarm Dismiss", "Run Step", "Stop Profile", "Cycle Reset", "Time Reset", "Time Reset All", "Time Set", "Tare CTs", "Save Profile", "Open Profile", "Get Profiles", "Update Screen", "Update Controls", "Save App Config", "Write Outputs", "Disable Background", "Enable Background", "Get/Release Control", "Log Fuel Change", "Fuel Change Popup", "Read Inputs", "Remote Timer Reset", "Controller Change", "Get Alarms", "Init Alarms", "Save Alarms", "Voltage Selection", "Set Watlow Temp 1", "Set Watlow Temp 2", "Get Pressure", "Write Tare Pressure", "Adjust Controls", "Reinit ADC", "Write Initial Times", "Write Pumps Present", "HMI Command", "Save Pump Times"]
        n434 = property on="Reset Tab" class="TabCtl (strict)"("Visible"=TRUE) -> (error out=w999:errorcluster)  [unwired: 2 in, 1 out]
        n435 = while {
          tunnel: ["pb.Reset OK"] -> w1006
          tunnel: w999 -> [_]
          stop <- w1009 stop-if-true
          n436 = Wait (ms)(milliseconds to wait=u32 10) -> ()  [unwired: 1 out]
          n437 = Or(x="pb.Reset Cancel", y="pb.Reset OK") -> (x .or. y?=w1009:bool)
        }
        n438 = Unbundle By Name(w998) -> ("pb.Resets"=w1005:bool[], "Initial Times"=w1002:dbl[])
        n439 = Search 1D Array(1D array=w1005, element=TRUE) -> (index of element=w1003:i32)  [unwired: 1 in]
        n440 = case shown="True" w1006 {
          tunnel: [w1012 w1018] -> w1007
          tunnel: w998 -> [w1012 w1017]
          tunnel: w1003 -> [_ w1016]
          tunnel: w1002 -> [_ w1015]
          tunnel: w1001 -> [_ w1014]
          tunnel: w997 -> [_ w1013]
          frame False {
          }
          frame True {
            n441 = case shown="\"Time Reset\"" w1013 {
              tunnel: w1017 -> [w1021 w1031 w1036]
              tunnel: [w1020 w1030 w1035] -> w1018
              tunnel: w1016 -> [_ w1026 _]
              tunnel: w1015 -> [_ w1029 _]
              tunnel: w1014 -> [_ w1024 w1034]
              frame "Cycle Reset", Default {
                n442 = Bundle By Name(cluster=w1021, "App Config.Cycles Completed"=u32 0) -> (w1020:T20)
              }
              frame "Time Reset" {
                n443 = Replace Array Subset(array=w1029, new element=0.0 ("new element/subarray"), index=w1026) -> (w1022:dbl[])
                n444 = Replace Array Subset(array=bool[] [FALSE, FALSE, FALSE, FALSE, FALSE, FALSE], new element=TRUE ("new element/subarray"), index=w1026) -> (w1027:bool[])
                n445 = xnode "Read/Write Control"("FPGA VI Reference In"=w1024, "Timer Resets"=w1027) -> ()  [unwired: 1 in, 2 out]
                n446 = Bundle By Name(cluster=w1031, "Initial Times"=w1022) -> (w1030:T20)
              }
              frame "Time Reset All" {
                n447 = xnode "Read/Write Control"("FPGA VI Reference In"=w1034, "Timer Resets"=bool[] [TRUE, TRUE, TRUE, TRUE, TRUE, TRUE] ("array")) -> ()  [unwired: 1 in, 2 out]
                n448 = Bundle By Name(cluster=w1036, "Initial Times"=dbl[] [0.0, 0.0, 0.0, 0.0, 0.0, 0.0] ("Intitial Times")) -> (w1035:T20)
              }
            }
          }
        }
        n449 = Insert Into Array(array=w996, index=0, new element=w994) -> (w995:T19[])
      }
      frame "Alarm" {
        w1045 = T19[] [] items=["Main", "Init Files", "Init", "Unused", "Save As", "Start Profile", "Check Step Time", "Alarm", "Alarm Dismiss", "Run Step", "Stop Profile", "Cycle Reset", "Time Reset", "Time Reset All", "Time Set", "Tare CTs", "Save Profile", "Open Profile", "Get Profiles", "Update Screen", "Update Controls", "Save App Config", "Write Outputs", "Disable Background", "Enable Background", "Get/Release Control", "Log Fuel Change", "Fuel Change Popup", "Read Inputs", "Remote Timer Reset", "Controller Change", "Get Alarms", "Init Alarms", "Save Alarms", "Voltage Selection", "Set Watlow Temp 1", "Set Watlow Temp 2", "Get Pressure", "Write Tare Pressure", "Adjust Controls", "Reinit ADC", "Write Initial Times", "Write Pumps Present", "HMI Command", "Save Pump Times"]
        n450 = Unbundle By Name(w1052) -> ("Alarm Message 1"=w1041:string, "Alarm Message 2"=w1048:string, "App Config.Location"=w1049:string, "App Config.Email Handler IP"=w1038:string, "Email Alarms Disabled"=w1037:bool)
        n451 = Format Into String(format string="%s\n\n%s", w1041, w1048) -> (resulting string=w1046:string)  [unwired: 2 in, 1 out]
        n452 = Concatenate Strings(w1049, " ALARM!" ("string")) -> (w1047:string)
        n453 = case shown="False" w1037 {
          tunnel: w1047 -> [w1055 _]
          tunnel: w1046 -> [w1054 _]
          tunnel: w1038 -> [w1053 _]
          frame False {
            n454 = flat-sequence {
              tunnel: w1055 -> [w1059]
              tunnel: w1054 -> [w1058]
              tunnel: w1053 -> [w1056]
              frame #0 {
                n455 = call "Email to Handler.vi"("Email Mode"=Email_Mode."Trigger Email", "Email Handler IP"=w1056, "Message:"=w1058, "Subject:"=w1059) -> ()  [unwired: 8 in]
              }
              frame #1 {
                n456 = call "Email Global.vi"("Write (F)"=TRUE, "Send Email"=TRUE) -> ()  [unwired: 9 in, 1 out]
              }
            }
          }
          frame True {
          }
        }
        n457 = flat-sequence {
          tunnel: w1046 -> [w1062]
          frame #0 {
            "Alarm Message" <- w1062
          }
          frame #1 {
            n458 = property on="Alarm Tab" class="TabCtl (strict)"("Visible"=TRUE) -> ()  [unwired: 2 in, 2 out]
          }
        }
        n459 = Bundle By Name(cluster=w1052, "Restart Alarm"=FALSE) -> (w1051:T20)
        n460 = Insert Into Array(array=w1043, index=0, new element=w1045) -> (w1042:T19[])
      }
      frame "Alarm Dismiss" {
        w1070 = T19[] [enum."Enable Background"] items=["Main", "Init Files", "Init", "Unused", "Save As", "Start Profile", "Check Step Time", "Alarm", "Alarm Dismiss", "Run Step", "Stop Profile", "Cycle Reset", "Time Reset", "Time Reset All", "Time Set", "Tare CTs", "Save Profile", "Open Profile", "Get Profiles", "Update Screen", "Update Controls", "Save App Config", "Write Outputs", "Disable Background", "Enable Background", "Get/Release Control", "Log Fuel Change", "Fuel Change Popup", "Read Inputs", "Remote Timer Reset", "Controller Change", "Get Alarms", "Init Alarms", "Save Alarms", "Voltage Selection", "Set Watlow Temp 1", "Set Watlow Temp 2", "Get Pressure", "Write Tare Pressure", "Adjust Controls", "Reinit ADC", "Write Initial Times", "Write Pumps Present", "HMI Command", "Save Pump Times"]
        n461 = Bundle By Name(cluster=w1066, "Alarm Latch"=FALSE) -> (w1065:T20)
        n462 = Insert Into Array(array=w1068, index=0, new element=w1070) -> (w1067:T19[])
      }
      frame "Time Set" {
        w1074 = T19[] [enum."Enable Background", enum."Write Initial Times"] items=["Main", "Init Files", "Init", "Unused", "Save As", "Start Profile", "Check Step Time", "Alarm", "Alarm Dismiss", "Run Step", "Stop Profile", "Cycle Reset", "Time Reset", "Time Reset All", "Time Set", "Tare CTs", "Save Profile", "Open Profile", "Get Profiles", "Update Screen", "Update Controls", "Save App Config", "Write Outputs", "Disable Background", "Enable Background", "Get/Release Control", "Log Fuel Change", "Fuel Change Popup", "Read Inputs", "Remote Timer Reset", "Controller Change", "Get Alarms", "Init Alarms", "Save Alarms", "Voltage Selection", "Set Watlow Temp 1", "Set Watlow Temp 2", "Get Pressure", "Write Tare Pressure", "Adjust Controls", "Reinit ADC", "Write Initial Times", "Write Pumps Present", "HMI Command", "Save Pump Times"]
        n463 = Unbundle By Name(w1084) -> ("pb.Sets"=w1083:bool[], "Initial Times"=w1078:dbl[], "Pump Data.Elapsed Time:"=w1081:dbl[])
        n464 = Search 1D Array(1D array=w1083, element=TRUE) -> (index of element=w1080:i32)  [unwired: 1 in]
        n465 = Index Array(array=w1081, index=w1080) -> (element=w1079:dbl)
        n466 = local write "New Time"(w1079) -> ()
        n467 = property on="Set Time Tab" class="TabCtl (strict)"("Visible"=TRUE) -> (error out=w1075:errorcluster)  [unwired: 2 in, 1 out]
        n468 = while {
          tunnel: ["pb.Set Time OK"] -> w1086
          tunnel: w1079 -> [_]
          tunnel: w1075 -> [_]
          stop <- w1089 stop-if-true
          n469 = Wait (ms)(milliseconds to wait=u32 10) -> ()  [unwired: 1 out]
          n470 = Or(x="pb.Set Time Cancel", y="pb.Set Time OK") -> (x .or. y?=w1089:bool)
        }
        n471 = case shown="True" w1086 {
          tunnel: w1084 -> [w1091 w1097]
          tunnel: [w1091 w1096] -> w1085
          tunnel: w1080 -> [_ w1093]
          tunnel: w1078 -> [_ w1095]
          tunnel: w1077 -> [_ w1094]
          frame False {
          }
          frame True {
            n472 = xnode "Read/Write Control"("FPGA VI Reference In"=w1094) -> ("FPGA VI Reference Out"=w1100:T21, "Timer Resets"=w1101:bool[])  [unwired: 1 in, 1 out]
            n473 = Replace Array Subset(array=w1095, new element="New Time", index=w1093) -> (w1102:dbl[])
            n474 = Replace Array Subset(array=w1101, new element=TRUE ("new element/subarray"), index=w1093) -> (w1099:bool[])
            n475 = Bundle By Name(cluster=w1097, "Initial Times"=w1102) -> (w1096:T20)
            n476 = xnode "Read/Write Control"("FPGA VI Reference In"=w1100, "Timer Resets"=w1099) -> ()  [unwired: 1 in, 2 out]
          }
        }
        n477 = Insert Into Array(array=w1072, index=0, new element=w1074) -> (w1071:T19[])
      }
      frame "Remote Timer Reset" {
        w1106 = T19[] [enum."Write Initial Times"] items=["Main", "Init Files", "Init", "Unused", "Save As", "Start Profile", "Check Step Time", "Alarm", "Alarm Dismiss", "Run Step", "Stop Profile", "Cycle Reset", "Time Reset", "Time Reset All", "Time Set", "Tare CTs", "Save Profile", "Open Profile", "Get Profiles", "Update Screen", "Update Controls", "Save App Config", "Write Outputs", "Disable Background", "Enable Background", "Get/Release Control", "Log Fuel Change", "Fuel Change Popup", "Read Inputs", "Remote Timer Reset", "Controller Change", "Get Alarms", "Init Alarms", "Save Alarms", "Voltage Selection", "Set Watlow Temp 1", "Set Watlow Temp 2", "Get Pressure", "Write Tare Pressure", "Adjust Controls", "Reinit ADC", "Write Initial Times", "Write Pumps Present", "HMI Command", "Save Pump Times"]
        n478 = xnode "Read/Write Control"("FPGA VI Reference In"=w1113, "Timer Resets"=bool[] [TRUE, TRUE, TRUE, TRUE, TRUE, TRUE] ("pb.Resets")) -> ("FPGA VI Reference Out"=w1110:T21)  [unwired: 1 in, 1 out]
        n479 = flat-sequence {
          tunnel: w1110 -> [w1115]
          tunnel: [w1115] -> w1109
          frame #0 {
            n480 = Wait (ms)(milliseconds to wait=u32 20) -> ()  [unwired: 1 out]
          }
        }
        n481 = xnode "Read/Write Control"("FPGA VI Reference In"=w1109, "Timer Resets"=bool[] [FALSE, FALSE, FALSE, FALSE, FALSE, FALSE] ("pb.Resets")) -> ()  [unwired: 1 in, 2 out]
        n482 = Bundle By Name(cluster=w1112, "Initial Times"=dbl[] [0.0, 0.0, 0.0, 0.0, 0.0, 0.0] ("Intitial Times")) -> (w1114:T20)
        n483 = Insert Into Array(array=w1103, index=0, new element=w1106) -> (w1104:T19[])
      }
      frame "Get/Release Control" {
        n484 = Unbundle By Name(w1121) -> ("Login"=w1118:bool)
        n485 = case shown="True" w1118 {
          tunnel: [T25."Disabled" ("Disabled") T25."Enabled" ("Disabled")] -> w1120
          frame False {
          }
          frame True {
          }
        }
        n486 = local write "Main Tab"(T5."Main" ("Main Tab")) -> ()
        n487 = property on="Main Tab" class="TabCtl (strict)"("DisabledEnum"=w1120) -> ()  [unwired: 2 in, 2 out]
        n488 = property on="pb.Stop Profile" class="Bool"("DisabledEnum"=w1120) -> ()  [unwired: 2 in, 2 out]
        n489 = property on="Monitoring Tab" class="TabCtl (strict)"("DisabledEnum"=w1120) -> ()  [unwired: 2 in, 2 out]
      }
      frame "Log Fuel Change" {
        n490 = Get Date/Time In Seconds() -> (seconds since 1Jan1904=w1129:timestamp)
        n491 = Unbundle By Name(w1131) -> ("Fuel Log Path"=w1128:path)
        n492 = Format Date/Time String(seconds (now)=w1129) -> (date/time string=w1127:string)  [unwired: 2 in]
        n493 = Build Array(w1127) -> (w1126:string[])
        n494 = call-poly <vilib>:"Write To Spreadsheet File.vi"("delimiter (\\t)"="," ("delimiter (\\t)"), "append to file? (new file:F)"=TRUE, "1D data"=w1126, "file path (dialog if empty)"=w1128) -> ()  [unwired: 4 in, 1 out]
      }
      frame "Fuel Change Popup" {
        w1132 = T19[] [enum."Enable Background"] items=["Main", "Init Files", "Init", "Unused", "Save As", "Start Profile", "Check Step Time", "Alarm", "Alarm Dismiss", "Run Step", "Stop Profile", "Cycle Reset", "Time Reset", "Time Reset All", "Time Set", "Tare CTs", "Save Profile", "Open Profile", "Get Profiles", "Update Screen", "Update Controls", "Save App Config", "Write Outputs", "Disable Background", "Enable Background", "Get/Release Control", "Log Fuel Change", "Fuel Change Popup", "Read Inputs", "Remote Timer Reset", "Controller Change", "Get Alarms", "Init Alarms", "Save Alarms", "Voltage Selection", "Set Watlow Temp 1", "Set Watlow Temp 2", "Get Pressure", "Write Tare Pressure", "Adjust Controls", "Reinit ADC", "Write Initial Times", "Write Pumps Present", "HMI Command", "Save Pump Times"]
        n495 = while {
          stop <- "pb.Fuel Change OK" stop-if-true
          n496 = property on="Fuel Change Tab" class="TabCtl (strict)"("Visible"=TRUE) -> ()  [unwired: 2 in, 2 out]
          n497 = Wait (ms)(milliseconds to wait=u32 20) -> ()  [unwired: 1 out]
        }
        n498 = Insert Into Array(array=w1136, index=0, new element=w1132) -> (w1135:T19[])
      }
      frame "Controller Change" {
        n499 = flat-sequence {
          tunnel: [w1149] -> w1148
          tunnel: [w1171] -> w1147
          tunnel: [w1157] -> w1144
          tunnel: w1145 -> [w1158]
          tunnel: w1146 -> [w1166]
          tunnel: w1145 -> [w1170]
          tunnel: w1148 -> [w1184]
          tunnel: w1147 -> [w1177]
          frame #0 {
            w1153 = dbl[] [0.0, 0.0, 0.0, 0.0, 0.0, 0.0] ("ControllerCurrent")
            n500 = Unbundle By Name(w1170) -> ("Controller List"=w1150:T18, "App Config.Controller Type:"=w1156:T2)
            n501 = Index Array(array=w1150, index=w1156) -> (element=w1152:T41)
            n502 = Unbundle By Name(w1152) -> ("Frequency"=w1154:i32, "CommSeg"=w1155:i32, "Controller?"=w1171:bool, "High Command"=w1160:dbl, "Low Command"=w1161:dbl, "Command Step"=w1162:dbl, "Stop Command"=w1163:dbl, "Invert PWM"=w1151:bool)
            n503 = Equal?(x=1, y=w1155) -> (x = y?=w1149:bool)
            n504 = case shown="False" w1149 {
              tunnel: [w1172 fxp<+,32,16> 1.0 ("CommFactor")] -> w1168
              tunnel: w1155 -> [w1173 _]
              frame False {
                n505 = case shown="10, Default" w1173 {
                  tunnel: [fxp<+,32,16> 4.0 ("CommFactor") fxp<+,32,16> 5.0 ("CommFactor")] -> w1172
                  frame 8 {
                  }
                  frame 10, Default {
                  }
                }
              }
              frame True {
              }
            }
            n506 = property on="ControllerCurrent" class="Arr (strict)"("Value"=w1153) -> ()  [unwired: 2 in, 2 out]
            n507 = local write "ControllerCurrent"(w1153) -> ()
            n508 = Divide(x=40000000.0 ("40 MHz"), y=w1154) -> (x/y=w1165:dbl)
            n509 = To Unsigned Long Integer(number=w1165) -> (unsigned 32bit integer=w1159:u32)
            n510 = xnode "Read/Write Control"("FPGA VI Reference In"=w1166, "Brushless"=w1149, "CommFactor"=w1168, "RPMhyst"="RPMhyst", "PWM Period (Ticks)"=w1159, "InvertPWM?"=w1151) -> ()  [unwired: 1 in, 2 out]
            n511 = Bundle By Name(cluster=w1158, "Stop Cmd"=w1163, "Controller Config"=w1152) -> (w1157:T20)
            n512 = property on="Numeric" class="DigNum (strict)"("Maximum"=w1160, "Minimum"=w1161, "Increment"=w1162) -> ()  [unwired: 2 in, 2 out]
          }
          frame #1 {
            n513 = Select(t="Pump\nCurrent\n(RMS)" ("Label.Text"), s=w1184, f="Pump\nCurrent\n(DC)" ("Label.Text")) -> (s? t:f=w1179:string)
            n514 = Select(t=T25."Enabled" ("Disabled"), s=w1177, f=T25."Disabled and Grayed Out" ("Disabled")) -> (s? t:f=w1180:T25)
            n515 = property on="PumpCurrent" class="Arr (strict)"("Caption.Text"=w1179) -> ()  [unwired: 2 in, 2 out]
            n516 = property on="ControllerCurrent" class="Arr (strict)"("DisabledEnum"=w1180) -> ()  [unwired: 2 in, 2 out]
          }
        }
        n517 = Insert Into Array(array=w1143, index=0, new element=Sequence_States."Voltage Selection" ("new element/subarray")) -> (w1142:T19[])
      }
      frame "Voltage Selection" {
        # "Delete out controller voltage\nrows to make array correct size"
        n518 = Unbundle By Name(w1194) -> ("Controller Config.Controller?"=w1186:bool, "CalArray"=w1191:dbl[][])
        n519 = Delete From Array(array=w1191, length=6, index (row)=48) -> (deleted portion=w1187:dbl[][], array with subset deleted=w1188:dbl[][])  [unwired: 1 in]
        n520 = case shown="False" w1186 {
          tunnel: w1188 -> [w1198 w1201]
          tunnel: w1187 -> [_ w1200]
          tunnel: [w1198 w1199] -> w1185
          frame False {
            # "Voltage @ Pump\nNo Change"
          }
          frame True {
            # "Switch Voltage\ncoefficients to \nthe controller"
            n521 = for {
              tunnel: w1200 -> [w1204] mode=indexing
              shift-right: [w1203] -> w1199
              shift-left: w1201 -> [w1205]
              i -> [w1202]
              n522 = Replace Array Subset(array=w1205, new element=w1204, index (row)=w1202) -> (w1203:dbl[][])  [unwired: 1 in]
            }
          }
        }
        n523 = Select(t="Controller\nVoltage\n(V)" ("Caption.Text"), s=w1186, f="Pump\nVoltage\n(V)" ("Caption.Text")) -> (s? t:f=w1197:string)
        n524 = property on="Voltages" class="Arr (strict)"("Caption.Text"=w1197) -> ()  [unwired: 2 in, 2 out]
        n525 = call "Tank Data Global.vi"("Pump Data Mode"=Pump_Data_Mode."Write Cal", "Cal Coefficients"=w1185) -> ()  [unwired: 10 in, 4 out]
      }
      frame "Set Watlow Temp 1", "Set Watlow Temp 2" {
        n526 = Unbundle By Name(w1214) -> ("Tank CMDs.Temp 1 CMD"=w1213:dbl, "Tank CMDs.Temp 2 CMD"=w1212:dbl)
        n527 = To Single Precision Float(number=w1213) -> (single precision float=w1211:sgl)
        n528 = To Single Precision Float(number=w1212) -> (single precision float=w1210:sgl)
        n529 = case shown="\"Set Watlow Temp 2\"" w1209 {
          tunnel: [Modbus_Mode."Tank 1 Write" ("Modbus Mode") Modbus_Mode."Tank 2 Write" ("Modbus Mode")] -> w1208
          tunnel: [Modbus_Variable."Setpoint" ("Variable") Modbus_Variable."Setpoint" ("Variable")] -> w1207
          tunnel: [w1216 w1219] -> w1206
          tunnel: w1211 -> [w1216 _]
          tunnel: w1210 -> [_ w1219]
          frame "Set Watlow Temp 1", Default {
          }
          frame "Set Watlow Temp 2" {
          }
        }
        n530 = call "Watlow Modbus.vi"("Modbus Mode"=w1208, "Data Write"=w1206, "Variable"=w1207) -> ()  [unwired: 7 in, 2 out]
      }
      frame "Get Pressure" {
        w1238 = T19[] [enum."Write Tare Pressure"] items=["Main", "Init Files", "Init", "Unused", "Save As", "Start Profile", "Check Step Time", "Alarm", "Alarm Dismiss", "Run Step", "Stop Profile", "Cycle Reset", "Time Reset", "Time Reset All", "Time Set", "Tare CTs", "Save Profile", "Open Profile", "Get Profiles", "Update Screen", "Update Controls", "Save App Config", "Write Outputs", "Disable Background", "Enable Background", "Get/Release Control", "Log Fuel Change", "Fuel Change Popup", "Read Inputs", "Remote Timer Reset", "Controller Change", "Get Alarms", "Init Alarms", "Save Alarms", "Voltage Selection", "Set Watlow Temp 1", "Set Watlow Temp 2", "Get Pressure", "Write Tare Pressure", "Adjust Controls", "Reinit ADC", "Write Initial Times", "Write Pumps Present", "HMI Command", "Save Pump Times"]
        n531 = flat-sequence {
          tunnel: [w1242] -> w1230
          frame #0 {
            n532 = call "Tank Data Global.vi"("Pump Data Mode"=Pump_Data_Mode."Write Pressure Offsets", "Pressure Offsets"=dbl[] [0.0, 0.0, 0.0, 0.0, 0.0, 0.0]) -> ()  [unwired: 10 in, 4 out]
          }
          frame #1 {
            # "Wait for write to occur."
            n533 = Wait (ms)(milliseconds to wait=u32 500) -> ()  [unwired: 1 out]
          }
          frame #2 {
            n534 = call "Tank Data Global.vi"("Pump Data Mode"=Pump_Data_Mode."Read") -> ("Tank Data OUT"=w1242:dbl[])  [unwired: 11 in, 3 out]
          }
        }
        n535 = Array Subset(array=w1230, index=30, length=6) -> (w1222:dbl[])
        n536 = Bundle By Name(cluster=w1231, "Pressure Offsets"=w1222) -> (w1232:T20)
        n537 = To Double Precision Float(number=w1222) -> (double precision float=w1227:dbl[])
        n538 = Array To Spreadsheet String(delimiter (Tab)=",", array=w1227, 3:"%.2f" ("format string")) -> (spreadsheet string=w1225:string)
        n539 = Write to Text File(file (use dialog)=path "c:/PressureOffsets", text=w1225) -> (refnum out=w1224:refnum<file>, error out=w1223:errorcluster)  [unwired: 2 in, 1 out]
        n540 = Close File(refnum=w1224, error in=w1223) -> ()  [unwired: 2 out]
        n541 = Insert Into Array(array=w1236, index=0, new element=w1238) -> (w1235:T19[])
      }
      frame "Write Tare Pressure" {
        n542 = Unbundle By Name(w1246) -> ("Pressure Offsets"=w1244:dbl[])
        n543 = call "Tank Data Global.vi"("Pump Data Mode"=Pump_Data_Mode."Write Pressure Offsets", "Pressure Offsets"=w1244) -> ()  [unwired: 10 in, 4 out]
      }
      frame "Adjust Controls" {
        n544 = Unbundle By Name(w1255) -> ("App Config.Voltage Limits"=w1249:T35, "App Config.Voltage Far PI"=w1250:T36, "App Config.Voltage Mid PI"=w1251:T37, "App Config.Voltage Close PI"=w1252:T38, "App Config.Voltage Scale"=w1253:cluster{"V_FFm":dbl, "V_FFb":dbl}, "App Config.Voltage Cutoffs"=w1248:cluster{"V_MidCutoff":dbl, "V_CloseCutoff":dbl})
        n545 = call "PI with FF.vi"("Cutoffs"=w1248, "FFcluster"=w1253, "ClosePIcluster"=w1252, "MidPIcluster"=w1251, "FarPIcluster"=w1250, "LimitCluster"=w1249, "Init (F)"=TRUE) -> ()  [unwired: 8 in, 1 out]
      }
      frame "Reinit ADC" {
        n546 = call "Init FPGA.vi"("FPGA Ref"=w1259) -> ("error out"=w1257:errorcluster, "FPGA Ref Out"=w1258:T21)  [unwired: 9 in]
        n547 = feedback #4(0) -> (w1260:i32)
        "ADC Errors" <- w1260
        n548 = Increment(x=w1260) -> (x+1=w1261:i32)
        n549 = feedback-in #4(w1261) -> ()
        n550 = call "Init ADCs.vi"("Error IN"=w1257, "FPGA Ref"=w1258) -> ()  [unwired: 7 in, 3 out]
      }
      frame "Write Initial Times" {
        n551 = Unbundle By Name(w1266) -> ("Initial Times"=w1265:dbl[])
        n552 = call "Tank Data Global.vi"("Pump Data Mode"=Pump_Data_Mode."Write Initial Times", "Intitial Times"=w1265) -> ()  [unwired: 10 in, 4 out]
      }
      frame "Write Pumps Present" {
        w1284 = T19[] [enum."Write Outputs", enum."Update Controls"] items=["Main", "Init Files", "Init", "Unused", "Save As", "Start Profile", "Check Step Time", "Alarm", "Alarm Dismiss", "Run Step", "Stop Profile", "Cycle Reset", "Time Reset", "Time Reset All", "Time Set", "Tare CTs", "Save Profile", "Open Profile", "Get Profiles", "Update Screen", "Update Controls", "Save App Config", "Write Outputs", "Disable Background", "Enable Background", "Get/Release Control", "Log Fuel Change", "Fuel Change Popup", "Read Inputs", "Remote Timer Reset", "Controller Change", "Get Alarms", "Init Alarms", "Save Alarms", "Voltage Selection", "Set Watlow Temp 1", "Set Watlow Temp 2", "Get Pressure", "Write Tare Pressure", "Adjust Controls", "Reinit ADC", "Write Initial Times", "Write Pumps Present", "HMI Command", "Save Pump Times"]
        # "Power and Ignition relays can only turn of if pumps are present."
        n553 = Unbundle By Name(w1273) -> ("App Config.Pumps Present"=w1276:T4, "Power Relay"=w1280:T4, "Ignition Relay"=w1279:T4)
        n554 = Cluster To Array(cluster=w1276) -> (array=w1269:bool[])
        n555 = Cluster To Array(cluster=w1280) -> (array=w1278:bool[])
        n556 = Cluster To Array(cluster=w1279) -> (array=w1277:bool[])
        n557 = call "Tank Data Global.vi"("Pump Data Mode"=Pump_Data_Mode."Write Pumps Present", "Pumps Present"=w1269) -> ()  [unwired: 10 in, 4 out]
        n558 = And(x=w1278, y=w1269) -> (x .and. y?=w1275:bool[])
        n559 = And(x=w1277, y=w1269) -> (x .and. y?=w1274:bool[])
        n560 = Array To Cluster(array=w1275) -> (cluster=w1271:T42)
        n561 = Array To Cluster(array=w1274) -> (cluster=w1270:T42)
        n562 = Bundle By Name(cluster=w1273, "Power Relay"=w1271, "Ignition Relay"=w1270) -> (w1272:T20)
        n563 = Insert Into Array(array=w1282, index=0, new element=w1284) -> (w1281:T19[])
      }
      frame "HMI Command" {
        w1299 = T19[] [] items=["Main", "Init Files", "Init", "Unused", "Save As", "Start Profile", "Check Step Time", "Alarm", "Alarm Dismiss", "Run Step", "Stop Profile", "Cycle Reset", "Time Reset", "Time Reset All", "Time Set", "Tare CTs", "Save Profile", "Open Profile", "Get Profiles", "Update Screen", "Update Controls", "Save App Config", "Write Outputs", "Disable Background", "Enable Background", "Get/Release Control", "Log Fuel Change", "Fuel Change Popup", "Read Inputs", "Remote Timer Reset", "Controller Change", "Get Alarms", "Init Alarms", "Save Alarms", "Voltage Selection", "Set Watlow Temp 1", "Set Watlow Temp 2", "Get Pressure", "Write Tare Pressure", "Adjust Controls", "Reinit ADC", "Write Initial Times", "Write Pumps Present", "HMI Command", "Save Pump Times"]
        n564 = flat-sequence {
          tunnel: [w1301] -> w1286
          frame #0 {
            n565 = call "RPi HMI Global.vi"("Mode"=HMI_Global_Mode."Reset Cmd") -> ()  [unwired: 10 in, 1 out]
          }
          frame #1 {
            n566 = call "RPi HMI Global.vi"("Mode"=HMI_Global_Mode."Read") -> ("HMI Cluster OUT"=w1301:T10)  [unwired: 10 in]
          }
        }
        n567 = Unbundle By Name(w1286) -> ("Power Relays"=w1295:T4, "Pump CMDs"=w1294:dbl[], "Tank CMDs.PS CMD"=w1293:dbl, "Tank CMDs.Press CMD"=w1292:dbl, "Tank CMDs.Temp 1 CMD"=w1291:dbl, "Tank CMDs.Temp 2 CMD"=w1290:dbl, "HMI Tog Buttons.Start Test"=w1289:bool)
        n568 = local write "Power Relay"(w1295) -> ()
        n569 = local write "Controller\nCMD"(w1294) -> ()
        n570 = local write "Power Supply Cmd:"(w1293) -> ()
        n571 = local write "PressureCMD"(w1292) -> ()
        n572 = local write "Tank 1 Temp Cmd:"(w1291) -> ()
        n573 = local write "Tank 2 Temp Cmd:"(w1290) -> ()
        n574 = local write "pb.Run Profile"(w1289) -> ()
        n575 = Insert Into Array(array=w1297, index=0, new element=w1299) -> (w1296:T19[])
        n576 = Bundle By Name(cluster=w1288, "HMI"=w1286) -> (w1287:T20)
      }
    }
  }
  n577 = flat-sequence {
    tunnel: w6 -> [_]
    tunnel: w5 -> [w1303]
    frame #0 {
      n578 = call "Data Loop.vi"("FPGA Ref"=w1303) -> ()  [unwired: 10 in, 1 out]
      n579 = call "Power Supply Loop.vi"("FPGA Ref"=w1303) -> ()  [unwired: 11 in]
      n580 = call "Data Logger Loop.vi"() -> ()  [unwired: 20 in]
      n581 = call "CAN Loop.vi"() -> ()  [unwired: 12 in]
      n582 = call "Email Loop.vi"() -> ()  [unwired: 12 in]
      n583 = call "Watlow Loop.vi"() -> ()  [unwired: 12 in]
      n584 = call "App Loop.vi"() -> ()  [unwired: 12 in]
      n585 = call "RPi HMI Loop.vi"() -> ()  [unwired: 20 in]
    }
  }
